vi "Washer HCC Newfi Main.vi"() -> ()   [LabVIEW 2018]
uses:
  Utility/Save File/Public/Type Definitions/Save File Washer.ctl
  Utility/Save File/File Setup (Public)/Type Definition/Save File DISH Dishwasher Details.ctl
  <vilib>/Platform/fileVersionInfo.llb/FileVersionInformation.ctl
  Washer DOE/Type Definitions/DOE Appliance Common.ctl
  Utility/Custom Pallet Controls/Custom Pallet String.ctl
  Utility/Save File/File Setup (Public)/Type Definition/DPT IMC Data.ctl
  Washer DOE/Type Definitions/DOE Dryer Standard.ctl
  Utility/Save File/Public/Type Definitions/Save File Appliance Display.ctl
  Utility/Save File/Public/Type Definitions/Save File Unit Type.ctl
  Utility/Save File/File Setup (Public)/Type Definition/Save File DOE File Path Control.ctl
  Utility/Save File/File Setup (Public)/Type Definition/Save File DOE Data Save Filepaths.ctl
  Type Definitions/HCC Station Group.ctl
  Utility/Save File/Save File.lvlib
  Drivers/Agilent 34972/Agilent 34970.lvlib
  Utility/Save File/File Setup.lvlib
panel:
  out "Network Var Set":u8
  in  "Quit":bool
  in  "Tab Control":enum32{"Main", "Settings"}(tab)
  in  "Array 4":T1[](array[typedef])=[{"Appliance Details"={"FileVersionInfo"={"FileVersion"="", "ProductName"="", "InternalName"="", "CompanyName"="", "LegalCopyright"="", "FileDescription"=""}, "Dishwasher Info"={"Open Cup Weight (gm):"=0.0, "Auto Cup Weight (gm):"=0.0, "Detergent-Dish:"="", "Inlet Temperature-Dish:"="", "Cycle Mode-Dish:"="", "Unit Control-Dish:"="", "Manufacturer-Dish:"=""}, "Washer Info"={"Hot Water Temperature (Fahrenheit):"="", "Cold Water Temperature (Fahrenheit):"="", "Capacity (cu.ft):"=0.0, "Initial Cloth Weight:"=0.0, "Cloth Lot:"=0, "Model Family:"="", "Program Name:"="", "Cycle Selection:"="", "Wash Temperature:"="", "Rinse Temperature:"="", "Load Size:"=""}, "File Name Output Array"=[], "Calibration Output Array"=[], "Appliance Common"={"Engineer:"="", "Model Number:"="", "Serial Number:"="", "Comments:"="", "Station ID:"="", "Technician:"="", "TR Number:"="", "Lab ID:"="", "Voltage:"="", "Water Pressure (PSI):"="", "Test Date:"="", "Computer Name:"="", "IP Address:"="", "Ambient RH:"="", "Frequency:"="", "Build:"="", "Filename:"="", "Test Type:"="", "Load Run #:"=0, "Ambient Temperature (F):"="", "File Path:"=path "", "Cycles Per Year"=60}, "Water Heater"={"Heating Mode:"=""}, "Dryer"={"Heat Setting:"="", "Washer Water Temperature (60 ± 5°F):"=60, "Water Hardness (PPM):"=17, "Dryness Setting:"="", "Dryer Type:"="", "Exhaust:"="", "Drying Cycle:"="", "Load Type:"="", "Nominal Load Weight"="", "Dryer Initial IMC Data"={"Measured IMC (lbs)"=7.0, "Actual Initial RMC (%)"=7.0, "RMC (Desired %)"=100.0, "Bone Dry Wt(lbs)"=7.0, "Tolerance(%)"=5.0, "Actual Final RMC (%)"=7.0, "CEF (lbf/kWh)"=0.0, "Minimum Weight (lbf)"=0.0, "Average Weight (lbf)"=0.0, "Maximum Weight (lbf)"=0.0, "Measured IMC In Range?"=FALSE, "Moisture Reduction Factor"=55.5, "Field Use Factor"=1.04, "Empty Dryer Cold Weigth"=0.0, "Energy Standard"=enum."D2-Automatic Dryer", "Weight Cloth (lbs)"=0.0, "Relative Moisture Content (%)"=0.0, "Relative Moisture Content - Avg (%)"=0.0}}}, "Display Data (RLT)"={"Status Color"=0, "Serial Number Display"="", "Cycle Count Display"=0, "Station Label Display"="", "Current Run Start Time Display"=0.0, "Board ID Display"="", "RPM Display"=0, "Current Display"=0.0, "Current Path Display"=path "", "Saving Display"=FALSE, "Unit Type Display"=enum."", "Total Time On Display"=0.0, "UI Button"=FALSE}}, {"Appliance Details"={"FileVersionInfo"={"FileVersion"="", "ProductName"="", "InternalName"="", "CompanyName"="", "LegalCopyright"="", "FileDescription"=""}, "Dishwasher Info"={"Open Cup Weight (gm):"=0.0, "Auto Cup Weight (gm):"=0.0, "Detergent-Dish:"="", "Inlet Temperature-Dish:"="", "Cycle Mode-Dish:"="", "Unit Control-Dish:"="", "Manufacturer-Dish:"=""}, "Washer Info"={"Hot Water Temperature (Fahrenheit):"="", "Cold Water Temperature (Fahrenheit):"="", "Capacity (cu.ft):"=0.0, "Initial Cloth Weight:"=0.0, "Cloth Lot:"=0, "Model Family:"="", "Program Name:"="", "Cycle Selection:"="", "Wash Temperature:"="", "Rinse Temperature:"="", "Load Size:"=""}, "File Name Output Array"=[], "Calibration Output Array"=[], "Appliance Common"={"Engineer:"="", "Model Number:"="", "Serial Number:"="", "Comments:"="", "Station ID:"="", "Technician:"="", "TR Number:"="", "Lab ID:"="", "Voltage:"="", "Water Pressure (PSI):"="", "Test Date:"="", "Computer Name:"="", "IP Address:"="", "Ambient RH:"="", "Frequency:"="", "Build:"="", "Filename:"="", "Test Type:"="", "Load Run #:"=0, "Ambient Temperature (F):"="", "File Path:"=path "", "Cycles Per Year"=60}, "Water Heater"={"Heating Mode:"=""}, "Dryer"={"Heat Setting:"="", "Washer Water Temperature (60 ± 5°F):"=60, "Water Hardness (PPM):"=17, "Dryness Setting:"="", "Dryer Type:"="", "Exhaust:"="", "Drying Cycle:"="", "Load Type:"="", "Nominal Load Weight"="", "Dryer Initial IMC Data"={"Measured IMC (lbs)"=7.0, "Actual Initial RMC (%)"=7.0, "RMC (Desired %)"=100.0, "Bone Dry Wt(lbs)"=7.0, "Tolerance(%)"=5.0, "Actual Final RMC (%)"=7.0, "CEF (lbf/kWh)"=0.0, "Minimum Weight (lbf)"=0.0, "Average Weight (lbf)"=0.0, "Maximum Weight (lbf)"=0.0, "Measured IMC In Range?"=FALSE, "Moisture Reduction Factor"=55.5, "Field Use Factor"=1.04, "Empty Dryer Cold Weigth"=0.0, "Energy Standard"=enum."D2-Automatic Dryer", "Weight Cloth (lbs)"=0.0, "Relative Moisture Content (%)"=0.0, "Relative Moisture Content - Avg (%)"=0.0}}}, "Display Data (RLT)"={"Status Color"=0, "Serial Number Display"="", "Cycle Count Display"=0, "Station Label Display"="", "Current Run Start Time Display"=0.0, "Board ID Display"="", "RPM Display"=0, "Current Display"=0.0, "Current Path Display"=path "", "Saving Display"=FALSE, "Unit Type Display"=enum."", "Total Time On Display"=0.0, "UI Button"=FALSE}}, {"Appliance Details"={"FileVersionInfo"={"FileVersion"="", "ProductName"="", "InternalName"="", "CompanyName"="", "LegalCopyright"="", "FileDescription"=""}, "Dishwasher Info"={"Open Cup Weight (gm):"=0.0, "Auto Cup Weight (gm):"=0.0, "Detergent-Dish:"="", "Inlet Temperature-Dish:"="", "Cycle Mode-Dish:"="", "Unit Control-Dish:"="", "Manufacturer-Dish:"=""}, "Washer Info"={"Hot Water Temperature (Fahrenheit):"="", "Cold Water Temperature (Fahrenheit):"="", "Capacity (cu.ft):"=0.0, "Initial Cloth Weight:"=0.0, "Cloth Lot:"=0, "Model Family:"="", "Program Name:"="", "Cycle Selection:"="", "Wash Temperature:"="", "Rinse Temperature:"="", "Load Size:"=""}, "File Name Output Array"=[], "Calibration Output Array"=[], "Appliance Common"={"Engineer:"="", "Model Number:"="", "Serial Number:"="", "Comments:"="", "Station ID:"="", "Technician:"="", "TR Number:"="", "Lab ID:"="", "Voltage:"="", "Water Pressure (PSI):"="", "Test Date:"="", "Computer Name:"="", "IP Address:"="", "Ambient RH:"="", "Frequency:"="", "Build:"="", "Filename:"="", "Test Type:"="", "Load Run #:"=0, "Ambient Temperature (F):"="", "File Path:"=path "", "Cycles Per Year"=60}, "Water Heater"={"Heating Mode:"=""}, "Dryer"={"Heat Setting:"="", "Washer Water Temperature (60 ± 5°F):"=60, "Water Hardness (PPM):"=17, "Dryness Setting:"="", "Dryer Type:"="", "Exhaust:"="", "Drying Cycle:"="", "Load Type:"="", "Nominal Load Weight"="", "Dryer Initial IMC Data"={"Measured IMC (lbs)"=7.0, "Actual Initial RMC (%)"=7.0, "RMC (Desired %)"=100.0, "Bone Dry Wt(lbs)"=7.0, "Tolerance(%)"=5.0, "Actual Final RMC (%)"=7.0, "CEF (lbf/kWh)"=0.0, "Minimum Weight (lbf)"=0.0, "Average Weight (lbf)"=0.0, "Maximum Weight (lbf)"=0.0, "Measured IMC In Range?"=FALSE, "Moisture Reduction Factor"=55.5, "Field Use Factor"=1.04, "Empty Dryer Cold Weigth"=0.0, "Energy Standard"=enum."D2-Automatic Dryer", "Weight Cloth (lbs)"=0.0, "Relative Moisture Content (%)"=0.0, "Relative Moisture Content - Avg (%)"=0.0}}}, "Display Data (RLT)"={"Status Color"=0, "Serial Number Display"="", "Cycle Count Display"=0, "Station Label Display"="", "Current Run Start Time Display"=0.0, "Board ID Display"="", "RPM Display"=0, "Current Display"=0.0, "Current Path Display"=path "", "Saving Display"=FALSE, "Unit Type Display"=enum."", "Total Time On Display"=0.0, "UI Button"=FALSE}}, {"Appliance Details"={"FileVersionInfo"={"FileVersion"="", "ProductName"="", "InternalName"="", "CompanyName"="", "LegalCopyright"="", "FileDescription"=""}, "Dishwasher Info"={"Open Cup Weight (gm):"=0.0, "Auto Cup Weight (gm):"=0.0, "Detergent-Dish:"="", "Inlet Temperature-Dish:"="", "Cycle Mode-Dish:"="", "Unit Control-Dish:"="", "Manufacturer-Dish:"=""}, "Washer Info"={"Hot Water Temperature (Fahrenheit):"="", "Cold Water Temperature (Fahrenheit):"="", "Capacity (cu.ft):"=0.0, "Initial Cloth Weight:"=0.0, "Cloth Lot:"=0, "Model Family:"="", "Program Name:"="", "Cycle Selection:"="", "Wash Temperature:"="", "Rinse Temperature:"="", "Load Size:"=""}, "File Name Output Array"=[], "Calibration Output Array"=[], "Appliance Common"={"Engineer:"="", "Model Number:"="", "Serial Number:"="", "Comments:"="", "Station ID:"="", "Technician:"="", "TR Number:"="", "Lab ID:"="", "Voltage:"="", "Water Pressure (PSI):"="", "Test Date:"="", "Computer Name:"="", "IP Address:"="", "Ambient RH:"="", "Frequency:"="", "Build:"="", "Filename:"="", "Test Type:"="", "Load Run #:"=0, "Ambient Temperature (F):"="", "File Path:"=path "", "Cycles Per Year"=60}, "Water Heater"={"Heating Mode:"=""}, "Dryer"={"Heat Setting:"="", "Washer Water Temperature (60 ± 5°F):"=60, "Water Hardness (PPM):"=17, "Dryness Setting:"="", "Dryer Type:"="", "Exhaust:"="", "Drying Cycle:"="", "Load Type:"="", "Nominal Load Weight"="", "Dryer Initial IMC Data"={"Measured IMC (lbs)"=7.0, "Actual Initial RMC (%)"=7.0, "RMC (Desired %)"=100.0, "Bone Dry Wt(lbs)"=7.0, "Tolerance(%)"=5.0, "Actual Final RMC (%)"=7.0, "CEF (lbf/kWh)"=0.0, "Minimum Weight (lbf)"=0.0, "Average Weight (lbf)"=0.0, "Maximum Weight (lbf)"=0.0, "Measured IMC In Range?"=FALSE, "Moisture Reduction Factor"=55.5, "Field Use Factor"=1.04, "Empty Dryer Cold Weigth"=0.0, "Energy Standard"=enum."D2-Automatic Dryer", "Weight Cloth (lbs)"=0.0, "Relative Moisture Content (%)"=0.0, "Relative Moisture Content - Avg (%)"=0.0}}}, "Display Data (RLT)"={"Status Color"=0, "Serial Number Display"="", "Cycle Count Display"=0, "Station Label Display"="", "Current Run Start Time Display"=0.0, "Board ID Display"="", "RPM Display"=0, "Current Display"=0.0, "Current Path Display"=path "", "Saving Display"=FALSE, "Unit Type Display"=enum."", "Total Time On Display"=0.0, "UI Button"=FALSE}}, {"Appliance Details"={"FileVersionInfo"={"FileVersion"="", "ProductName"="", "InternalName"="", "CompanyName"="", "LegalCopyright"="", "FileDescription"=""}, "Dishwasher Info"={"Open Cup Weight (gm):"=0.0, "Auto Cup Weight (gm):"=0.0, "Detergent-Dish:"="", "Inlet Temperature-Dish:"="", "Cycle Mode-Dish:"="", "Unit Control-Dish:"="", "Manufacturer-Dish:"=""}, "Washer Info"={"Hot Water Temperature (Fahrenheit):"="", "Cold Water Temperature (Fahrenheit):"="", "Capacity (cu.ft):"=0.0, "Initial Cloth Weight:"=0.0, "Cloth Lot:"=0, "Model Family:"="", "Program Name:"="", "Cycle Selection:"="", "Wash Temperature:"="", "Rinse Temperature:"="", "Load Size:"=""}, "File Name Output Array"=[], "Calibration Output Array"=[], "Appliance Common"={"Engineer:"="", "Model Number:"="", "Serial Number:"="", "Comments:"="", "Station ID:"="", "Technician:"="", "TR Number:"="", "Lab ID:"="", "Voltage:"="", "Water Pressure (PSI):"="", "Test Date:"="", "Computer Name:"="", "IP Address:"="", "Ambient RH:"="", "Frequency:"="", "Build:"="", "Filename:"="", "Test Type:"="", "Load Run #:"=0, "Ambient Temperature (F):"="", "File Path:"=path "", "Cycles Per Year"=60}, "Water Heater"={"Heating Mode:"=""}, "Dryer"={"Heat Setting:"="", "Washer Water Temperature (60 ± 5°F):"=60, "Water Hardness (PPM):"=17, "Dryness Setting:"="", "Dryer Type:"="", "Exhaust:"="", "Drying Cycle:"="", "Load Type:"="", "Nominal Load Weight"="", "Dryer Initial IMC Data"={"Measured IMC (lbs)"=7.0, "Actual Initial RMC (%)"=7.0, "RMC (Desired %)"=100.0, "Bone Dry Wt(lbs)"=7.0, "Tolerance(%)"=5.0, "Actual Final RMC (%)"=7.0, "CEF (lbf/kWh)"=0.0, "Minimum Weight (lbf)"=0.0, "Average Weight (lbf)"=0.0, "Maximum Weight (lbf)"=0.0, "Measured IMC In Range?"=FALSE, "Moisture Reduction Factor"=55.5, "Field Use Factor"=1.04, "Empty Dryer Cold Weigth"=0.0, "Energy Standard"=enum."D2-Automatic Dryer", "Weight Cloth (lbs)"=0.0, "Relative Moisture Content (%)"=0.0, "Relative Moisture Content - Avg (%)"=0.0}}}, "Display Data (RLT)"={"Status Color"=0, "Serial Number Display"="", "Cycle Count Display"=0, "Station Label Display"="", "Current Run Start Time Display"=0.0, "Board ID Display"="", "RPM Display"=0, "Current Display"=0.0, "Current Path Display"=path "", "Saving Display"=FALSE, "Unit Type Display"=enum."", "Total Time On Display"=0.0, "UI Button"=FALSE}}, {"Appliance Details"={"FileVersionInfo"={"FileVersion"="", "ProductName"="", "InternalName"="", "CompanyName"="", "LegalCopyright"="", "FileDescription"=""}, "Dishwasher Info"={"Open Cup Weight (gm):"=0.0, "Auto Cup Weight (gm):"=0.0, "Detergent-Dish:"="", "Inlet Temperature-Dish:"="", "Cycle Mode-Dish:"="", "Unit Control-Dish:"="", "Manufacturer-Dish:"=""}, "Washer Info"={"Hot Water Temperature (Fahrenheit):"="", "Cold Water Temperature (Fahrenheit):"="", "Capacity (cu.ft):"=0.0, "Initial Cloth Weight:"=0.0, "Cloth Lot:"=0, "Model Family:"="", "Program Name:"="", "Cycle Selection:"="", "Wash Temperature:"="", "Rinse Temperature:"="", "Load Size:"=""}, "File Name Output Array"=[], "Calibration Output Array"=[], "Appliance Common"={"Engineer:"="", "Model Number:"="", "Serial Number:"="", "Comments:"="", "Station ID:"="", "Technician:"="", "TR Number:"="", "Lab ID:"="", "Voltage:"="", "Water Pressure (PSI):"="", "Test Date:"="", "Computer Name:"="", "IP Address:"="", "Ambient RH:"="", "Frequency:"="", "Build:"="", "Filename:"="", "Test Type:"="", "Load Run #:"=0, "Ambient Temperature (F):"="", "File Path:"=path "", "Cycles Per Year"=60}, "Water Heater"={"Heating Mode:"=""}, "Dryer"={"Heat Setting:"="", "Washer Water Temperature (60 ± 5°F):"=60, "Water Hardness (PPM):"=17, "Dryness Setting:"="", "Dryer Type:"="", "Exhaust:"="", "Drying Cycle:"="", "Load Type:"="", "Nominal Load Weight"="", "Dryer Initial IMC Data"={"Measured IMC (lbs)"=7.0, "Actual Initial RMC (%)"=7.0, "RMC (Desired %)"=100.0, "Bone Dry Wt(lbs)"=7.0, "Tolerance(%)"=5.0, "Actual Final RMC (%)"=7.0, "CEF (lbf/kWh)"=0.0, "Minimum Weight (lbf)"=0.0, "Average Weight (lbf)"=0.0, "Maximum Weight (lbf)"=0.0, "Measured IMC In Range?"=FALSE, "Moisture Reduction Factor"=55.5, "Field Use Factor"=1.04, "Empty Dryer Cold Weigth"=0.0, "Energy Standard"=enum."D2-Automatic Dryer", "Weight Cloth (lbs)"=0.0, "Relative Moisture Content (%)"=0.0, "Relative Moisture Content - Avg (%)"=0.0}}}, "Display Data (RLT)"={"Status Color"=0, "Serial Number Display"="", "Cycle Count Display"=0, "Station Label Display"="", "Current Run Start Time Display"=0.0, "Board ID Display"="", "RPM Display"=0, "Current Display"=0.0, "Current Path Display"=path "", "Saving Display"=FALSE, "Unit Type Display"=enum."", "Total Time On Display"=0.0, "UI Button"=FALSE}}] {"Display Data (RLT)"."Current Display" format="%.2f"; "Display Data (RLT)"."Cycle Count Display" format="%04d"; "Appliance Details"."Dryer"."Dryer Initial IMC Data"."Maximum Weight (lbf)" format="%03_6g"; "Appliance Details"."Dryer"."Dryer Initial IMC Data"."Average Weight (lbf)" format="%03_6g"; "Appliance Details"."Dryer"."Dryer Initial IMC Data"."Minimum Weight (lbf)" format="%03_6g"; "Appliance Details"."Dryer"."Dryer Initial IMC Data"."CEF (lbf/kWh)" format="%03_6g"; "Appliance Details"."Dryer"."Dryer Initial IMC Data"."Actual Final RMC (%)" format="%03_6g"; "Appliance Details"."Dryer"."Dryer Initial IMC Data"."Tolerance(%)" format="%0#_6g"; "Appliance Details"."Dryer"."Dryer Initial IMC Data"."Bone Dry Wt(lbs)" format="%03_6g"; "Appliance Details"."Dryer"."Dryer Initial IMC Data"."RMC (Desired %)" format="%0#_6g"; "Appliance Details"."Dryer"."Dryer Initial IMC Data"."Actual Initial RMC (%)" format="%03_6g"; "Appliance Details"."Dryer"."Dryer Initial IMC Data"."Measured IMC (lbs)" format="%0#_6g"}
  in  "Array 3":T1[](array[typedef])=[{"Appliance Details"={"FileVersionInfo"={"FileVersion"="", "ProductName"="", "InternalName"="", "CompanyName"="", "LegalCopyright"="", "FileDescription"=""}, "Dishwasher Info"={"Open Cup Weight (gm):"=0.0, "Auto Cup Weight (gm):"=0.0, "Detergent-Dish:"="", "Inlet Temperature-Dish:"="", "Cycle Mode-Dish:"="", "Unit Control-Dish:"="", "Manufacturer-Dish:"=""}, "Washer Info"={"Hot Water Temperature (Fahrenheit):"="", "Cold Water Temperature (Fahrenheit):"="", "Capacity (cu.ft):"=0.0, "Initial Cloth Weight:"=0.0, "Cloth Lot:"=0, "Model Family:"="", "Program Name:"="", "Cycle Selection:"="", "Wash Temperature:"="", "Rinse Temperature:"="", "Load Size:"=""}, "File Name Output Array"=[], "Calibration Output Array"=[], "Appliance Common"={"Engineer:"="", "Model Number:"="", "Serial Number:"="", "Comments:"="", "Station ID:"="", "Technician:"="", "TR Number:"="", "Lab ID:"="", "Voltage:"="", "Water Pressure (PSI):"="", "Test Date:"="", "Computer Name:"="", "IP Address:"="", "Ambient RH:"="", "Frequency:"="", "Build:"="", "Filename:"="", "Test Type:"="", "Load Run #:"=0, "Ambient Temperature (F):"="", "File Path:"=path "", "Cycles Per Year"=60}, "Water Heater"={"Heating Mode:"=""}, "Dryer"={"Heat Setting:"="", "Washer Water Temperature (60 ± 5°F):"=60, "Water Hardness (PPM):"=17, "Dryness Setting:"="", "Dryer Type:"="", "Exhaust:"="", "Drying Cycle:"="", "Load Type:"="", "Nominal Load Weight"="", "Dryer Initial IMC Data"={"Measured IMC (lbs)"=7.0, "Actual Initial RMC (%)"=7.0, "RMC (Desired %)"=100.0, "Bone Dry Wt(lbs)"=7.0, "Tolerance(%)"=5.0, "Actual Final RMC (%)"=7.0, "CEF (lbf/kWh)"=0.0, "Minimum Weight (lbf)"=0.0, "Average Weight (lbf)"=0.0, "Maximum Weight (lbf)"=0.0, "Measured IMC In Range?"=FALSE, "Moisture Reduction Factor"=55.5, "Field Use Factor"=1.04, "Empty Dryer Cold Weigth"=0.0, "Energy Standard"=enum."D2-Automatic Dryer", "Weight Cloth (lbs)"=0.0, "Relative Moisture Content (%)"=0.0, "Relative Moisture Content - Avg (%)"=0.0}}}, "Display Data (RLT)"={"Status Color"=0, "Serial Number Display"="", "Cycle Count Display"=0, "Station Label Display"="", "Current Run Start Time Display"=0.0, "Board ID Display"="", "RPM Display"=0, "Current Display"=0.0, "Current Path Display"=path "", "Saving Display"=FALSE, "Unit Type Display"=enum."", "Total Time On Display"=0.0, "UI Button"=FALSE}}, {"Appliance Details"={"FileVersionInfo"={"FileVersion"="", "ProductName"="", "InternalName"="", "CompanyName"="", "LegalCopyright"="", "FileDescription"=""}, "Dishwasher Info"={"Open Cup Weight (gm):"=0.0, "Auto Cup Weight (gm):"=0.0, "Detergent-Dish:"="", "Inlet Temperature-Dish:"="", "Cycle Mode-Dish:"="", "Unit Control-Dish:"="", "Manufacturer-Dish:"=""}, "Washer Info"={"Hot Water Temperature (Fahrenheit):"="", "Cold Water Temperature (Fahrenheit):"="", "Capacity (cu.ft):"=0.0, "Initial Cloth Weight:"=0.0, "Cloth Lot:"=0, "Model Family:"="", "Program Name:"="", "Cycle Selection:"="", "Wash Temperature:"="", "Rinse Temperature:"="", "Load Size:"=""}, "File Name Output Array"=[], "Calibration Output Array"=[], "Appliance Common"={"Engineer:"="", "Model Number:"="", "Serial Number:"="", "Comments:"="", "Station ID:"="", "Technician:"="", "TR Number:"="", "Lab ID:"="", "Voltage:"="", "Water Pressure (PSI):"="", "Test Date:"="", "Computer Name:"="", "IP Address:"="", "Ambient RH:"="", "Frequency:"="", "Build:"="", "Filename:"="", "Test Type:"="", "Load Run #:"=0, "Ambient Temperature (F):"="", "File Path:"=path "", "Cycles Per Year"=60}, "Water Heater"={"Heating Mode:"=""}, "Dryer"={"Heat Setting:"="", "Washer Water Temperature (60 ± 5°F):"=60, "Water Hardness (PPM):"=17, "Dryness Setting:"="", "Dryer Type:"="", "Exhaust:"="", "Drying Cycle:"="", "Load Type:"="", "Nominal Load Weight"="", "Dryer Initial IMC Data"={"Measured IMC (lbs)"=7.0, "Actual Initial RMC (%)"=7.0, "RMC (Desired %)"=100.0, "Bone Dry Wt(lbs)"=7.0, "Tolerance(%)"=5.0, "Actual Final RMC (%)"=7.0, "CEF (lbf/kWh)"=0.0, "Minimum Weight (lbf)"=0.0, "Average Weight (lbf)"=0.0, "Maximum Weight (lbf)"=0.0, "Measured IMC In Range?"=FALSE, "Moisture Reduction Factor"=55.5, "Field Use Factor"=1.04, "Empty Dryer Cold Weigth"=0.0, "Energy Standard"=enum."D2-Automatic Dryer", "Weight Cloth (lbs)"=0.0, "Relative Moisture Content (%)"=0.0, "Relative Moisture Content - Avg (%)"=0.0}}}, "Display Data (RLT)"={"Status Color"=0, "Serial Number Display"="", "Cycle Count Display"=0, "Station Label Display"="", "Current Run Start Time Display"=0.0, "Board ID Display"="", "RPM Display"=0, "Current Display"=0.0, "Current Path Display"=path "", "Saving Display"=FALSE, "Unit Type Display"=enum."", "Total Time On Display"=0.0, "UI Button"=FALSE}}, {"Appliance Details"={"FileVersionInfo"={"FileVersion"="", "ProductName"="", "InternalName"="", "CompanyName"="", "LegalCopyright"="", "FileDescription"=""}, "Dishwasher Info"={"Open Cup Weight (gm):"=0.0, "Auto Cup Weight (gm):"=0.0, "Detergent-Dish:"="", "Inlet Temperature-Dish:"="", "Cycle Mode-Dish:"="", "Unit Control-Dish:"="", "Manufacturer-Dish:"=""}, "Washer Info"={"Hot Water Temperature (Fahrenheit):"="", "Cold Water Temperature (Fahrenheit):"="", "Capacity (cu.ft):"=0.0, "Initial Cloth Weight:"=0.0, "Cloth Lot:"=0, "Model Family:"="", "Program Name:"="", "Cycle Selection:"="", "Wash Temperature:"="", "Rinse Temperature:"="", "Load Size:"=""}, "File Name Output Array"=[], "Calibration Output Array"=[], "Appliance Common"={"Engineer:"="", "Model Number:"="", "Serial Number:"="", "Comments:"="", "Station ID:"="", "Technician:"="", "TR Number:"="", "Lab ID:"="", "Voltage:"="", "Water Pressure (PSI):"="", "Test Date:"="", "Computer Name:"="", "IP Address:"="", "Ambient RH:"="", "Frequency:"="", "Build:"="", "Filename:"="", "Test Type:"="", "Load Run #:"=0, "Ambient Temperature (F):"="", "File Path:"=path "", "Cycles Per Year"=60}, "Water Heater"={"Heating Mode:"=""}, "Dryer"={"Heat Setting:"="", "Washer Water Temperature (60 ± 5°F):"=60, "Water Hardness (PPM):"=17, "Dryness Setting:"="", "Dryer Type:"="", "Exhaust:"="", "Drying Cycle:"="", "Load Type:"="", "Nominal Load Weight"="", "Dryer Initial IMC Data"={"Measured IMC (lbs)"=7.0, "Actual Initial RMC (%)"=7.0, "RMC (Desired %)"=100.0, "Bone Dry Wt(lbs)"=7.0, "Tolerance(%)"=5.0, "Actual Final RMC (%)"=7.0, "CEF (lbf/kWh)"=0.0, "Minimum Weight (lbf)"=0.0, "Average Weight (lbf)"=0.0, "Maximum Weight (lbf)"=0.0, "Measured IMC In Range?"=FALSE, "Moisture Reduction Factor"=55.5, "Field Use Factor"=1.04, "Empty Dryer Cold Weigth"=0.0, "Energy Standard"=enum."D2-Automatic Dryer", "Weight Cloth (lbs)"=0.0, "Relative Moisture Content (%)"=0.0, "Relative Moisture Content - Avg (%)"=0.0}}}, "Display Data (RLT)"={"Status Color"=0, "Serial Number Display"="", "Cycle Count Display"=0, "Station Label Display"="", "Current Run Start Time Display"=0.0, "Board ID Display"="", "RPM Display"=0, "Current Display"=0.0, "Current Path Display"=path "", "Saving Display"=FALSE, "Unit Type Display"=enum."", "Total Time On Display"=0.0, "UI Button"=FALSE}}, {"Appliance Details"={"FileVersionInfo"={"FileVersion"="", "ProductName"="", "InternalName"="", "CompanyName"="", "LegalCopyright"="", "FileDescription"=""}, "Dishwasher Info"={"Open Cup Weight (gm):"=0.0, "Auto Cup Weight (gm):"=0.0, "Detergent-Dish:"="", "Inlet Temperature-Dish:"="", "Cycle Mode-Dish:"="", "Unit Control-Dish:"="", "Manufacturer-Dish:"=""}, "Washer Info"={"Hot Water Temperature (Fahrenheit):"="", "Cold Water Temperature (Fahrenheit):"="", "Capacity (cu.ft):"=0.0, "Initial Cloth Weight:"=0.0, "Cloth Lot:"=0, "Model Family:"="", "Program Name:"="", "Cycle Selection:"="", "Wash Temperature:"="", "Rinse Temperature:"="", "Load Size:"=""}, "File Name Output Array"=[], "Calibration Output Array"=[], "Appliance Common"={"Engineer:"="", "Model Number:"="", "Serial Number:"="", "Comments:"="", "Station ID:"="", "Technician:"="", "TR Number:"="", "Lab ID:"="", "Voltage:"="", "Water Pressure (PSI):"="", "Test Date:"="", "Computer Name:"="", "IP Address:"="", "Ambient RH:"="", "Frequency:"="", "Build:"="", "Filename:"="", "Test Type:"="", "Load Run #:"=0, "Ambient Temperature (F):"="", "File Path:"=path "", "Cycles Per Year"=60}, "Water Heater"={"Heating Mode:"=""}, "Dryer"={"Heat Setting:"="", "Washer Water Temperature (60 ± 5°F):"=60, "Water Hardness (PPM):"=17, "Dryness Setting:"="", "Dryer Type:"="", "Exhaust:"="", "Drying Cycle:"="", "Load Type:"="", "Nominal Load Weight"="", "Dryer Initial IMC Data"={"Measured IMC (lbs)"=7.0, "Actual Initial RMC (%)"=7.0, "RMC (Desired %)"=100.0, "Bone Dry Wt(lbs)"=7.0, "Tolerance(%)"=5.0, "Actual Final RMC (%)"=7.0, "CEF (lbf/kWh)"=0.0, "Minimum Weight (lbf)"=0.0, "Average Weight (lbf)"=0.0, "Maximum Weight (lbf)"=0.0, "Measured IMC In Range?"=FALSE, "Moisture Reduction Factor"=55.5, "Field Use Factor"=1.04, "Empty Dryer Cold Weigth"=0.0, "Energy Standard"=enum."D2-Automatic Dryer", "Weight Cloth (lbs)"=0.0, "Relative Moisture Content (%)"=0.0, "Relative Moisture Content - Avg (%)"=0.0}}}, "Display Data (RLT)"={"Status Color"=0, "Serial Number Display"="", "Cycle Count Display"=0, "Station Label Display"="", "Current Run Start Time Display"=0.0, "Board ID Display"="", "RPM Display"=0, "Current Display"=0.0, "Current Path Display"=path "", "Saving Display"=FALSE, "Unit Type Display"=enum."", "Total Time On Display"=0.0, "UI Button"=FALSE}}, {"Appliance Details"={"FileVersionInfo"={"FileVersion"="", "ProductName"="", "InternalName"="", "CompanyName"="", "LegalCopyright"="", "FileDescription"=""}, "Dishwasher Info"={"Open Cup Weight (gm):"=0.0, "Auto Cup Weight (gm):"=0.0, "Detergent-Dish:"="", "Inlet Temperature-Dish:"="", "Cycle Mode-Dish:"="", "Unit Control-Dish:"="", "Manufacturer-Dish:"=""}, "Washer Info"={"Hot Water Temperature (Fahrenheit):"="", "Cold Water Temperature (Fahrenheit):"="", "Capacity (cu.ft):"=0.0, "Initial Cloth Weight:"=0.0, "Cloth Lot:"=0, "Model Family:"="", "Program Name:"="", "Cycle Selection:"="", "Wash Temperature:"="", "Rinse Temperature:"="", "Load Size:"=""}, "File Name Output Array"=[], "Calibration Output Array"=[], "Appliance Common"={"Engineer:"="", "Model Number:"="", "Serial Number:"="", "Comments:"="", "Station ID:"="", "Technician:"="", "TR Number:"="", "Lab ID:"="", "Voltage:"="", "Water Pressure (PSI):"="", "Test Date:"="", "Computer Name:"="", "IP Address:"="", "Ambient RH:"="", "Frequency:"="", "Build:"="", "Filename:"="", "Test Type:"="", "Load Run #:"=0, "Ambient Temperature (F):"="", "File Path:"=path "", "Cycles Per Year"=60}, "Water Heater"={"Heating Mode:"=""}, "Dryer"={"Heat Setting:"="", "Washer Water Temperature (60 ± 5°F):"=60, "Water Hardness (PPM):"=17, "Dryness Setting:"="", "Dryer Type:"="", "Exhaust:"="", "Drying Cycle:"="", "Load Type:"="", "Nominal Load Weight"="", "Dryer Initial IMC Data"={"Measured IMC (lbs)"=7.0, "Actual Initial RMC (%)"=7.0, "RMC (Desired %)"=100.0, "Bone Dry Wt(lbs)"=7.0, "Tolerance(%)"=5.0, "Actual Final RMC (%)"=7.0, "CEF (lbf/kWh)"=0.0, "Minimum Weight (lbf)"=0.0, "Average Weight (lbf)"=0.0, "Maximum Weight (lbf)"=0.0, "Measured IMC In Range?"=FALSE, "Moisture Reduction Factor"=55.5, "Field Use Factor"=1.04, "Empty Dryer Cold Weigth"=0.0, "Energy Standard"=enum."D2-Automatic Dryer", "Weight Cloth (lbs)"=0.0, "Relative Moisture Content (%)"=0.0, "Relative Moisture Content - Avg (%)"=0.0}}}, "Display Data (RLT)"={"Status Color"=0, "Serial Number Display"="", "Cycle Count Display"=0, "Station Label Display"="", "Current Run Start Time Display"=0.0, "Board ID Display"="", "RPM Display"=0, "Current Display"=0.0, "Current Path Display"=path "", "Saving Display"=FALSE, "Unit Type Display"=enum."", "Total Time On Display"=0.0, "UI Button"=FALSE}}, {"Appliance Details"={"FileVersionInfo"={"FileVersion"="", "ProductName"="", "InternalName"="", "CompanyName"="", "LegalCopyright"="", "FileDescription"=""}, "Dishwasher Info"={"Open Cup Weight (gm):"=0.0, "Auto Cup Weight (gm):"=0.0, "Detergent-Dish:"="", "Inlet Temperature-Dish:"="", "Cycle Mode-Dish:"="", "Unit Control-Dish:"="", "Manufacturer-Dish:"=""}, "Washer Info"={"Hot Water Temperature (Fahrenheit):"="", "Cold Water Temperature (Fahrenheit):"="", "Capacity (cu.ft):"=0.0, "Initial Cloth Weight:"=0.0, "Cloth Lot:"=0, "Model Family:"="", "Program Name:"="", "Cycle Selection:"="", "Wash Temperature:"="", "Rinse Temperature:"="", "Load Size:"=""}, "File Name Output Array"=[], "Calibration Output Array"=[], "Appliance Common"={"Engineer:"="", "Model Number:"="", "Serial Number:"="", "Comments:"="", "Station ID:"="", "Technician:"="", "TR Number:"="", "Lab ID:"="", "Voltage:"="", "Water Pressure (PSI):"="", "Test Date:"="", "Computer Name:"="", "IP Address:"="", "Ambient RH:"="", "Frequency:"="", "Build:"="", "Filename:"="", "Test Type:"="", "Load Run #:"=0, "Ambient Temperature (F):"="", "File Path:"=path "", "Cycles Per Year"=60}, "Water Heater"={"Heating Mode:"=""}, "Dryer"={"Heat Setting:"="", "Washer Water Temperature (60 ± 5°F):"=60, "Water Hardness (PPM):"=17, "Dryness Setting:"="", "Dryer Type:"="", "Exhaust:"="", "Drying Cycle:"="", "Load Type:"="", "Nominal Load Weight"="", "Dryer Initial IMC Data"={"Measured IMC (lbs)"=7.0, "Actual Initial RMC (%)"=7.0, "RMC (Desired %)"=100.0, "Bone Dry Wt(lbs)"=7.0, "Tolerance(%)"=5.0, "Actual Final RMC (%)"=7.0, "CEF (lbf/kWh)"=0.0, "Minimum Weight (lbf)"=0.0, "Average Weight (lbf)"=0.0, "Maximum Weight (lbf)"=0.0, "Measured IMC In Range?"=FALSE, "Moisture Reduction Factor"=55.5, "Field Use Factor"=1.04, "Empty Dryer Cold Weigth"=0.0, "Energy Standard"=enum."D2-Automatic Dryer", "Weight Cloth (lbs)"=0.0, "Relative Moisture Content (%)"=0.0, "Relative Moisture Content - Avg (%)"=0.0}}}, "Display Data (RLT)"={"Status Color"=0, "Serial Number Display"="", "Cycle Count Display"=0, "Station Label Display"="", "Current Run Start Time Display"=0.0, "Board ID Display"="", "RPM Display"=0, "Current Display"=0.0, "Current Path Display"=path "", "Saving Display"=FALSE, "Unit Type Display"=enum."", "Total Time On Display"=0.0, "UI Button"=FALSE}}] {"Display Data (RLT)"."Current Display" format="%.2f"; "Display Data (RLT)"."Cycle Count Display" format="%04d"; "Appliance Details"."Dryer"."Dryer Initial IMC Data"."Maximum Weight (lbf)" format="%03_6g"; "Appliance Details"."Dryer"."Dryer Initial IMC Data"."Average Weight (lbf)" format="%03_6g"; "Appliance Details"."Dryer"."Dryer Initial IMC Data"."Minimum Weight (lbf)" format="%03_6g"; "Appliance Details"."Dryer"."Dryer Initial IMC Data"."CEF (lbf/kWh)" format="%03_6g"; "Appliance Details"."Dryer"."Dryer Initial IMC Data"."Actual Final RMC (%)" format="%03_6g"; "Appliance Details"."Dryer"."Dryer Initial IMC Data"."Tolerance(%)" format="%0#_6g"; "Appliance Details"."Dryer"."Dryer Initial IMC Data"."Bone Dry Wt(lbs)" format="%03_6g"; "Appliance Details"."Dryer"."Dryer Initial IMC Data"."RMC (Desired %)" format="%0#_6g"; "Appliance Details"."Dryer"."Dryer Initial IMC Data"."Actual Initial RMC (%)" format="%03_6g"; "Appliance Details"."Dryer"."Dryer Initial IMC Data"."Measured IMC (lbs)" format="%0#_6g"}
  in  "Array":T1[](array[typedef])=[{"Appliance Details"={"FileVersionInfo"={"FileVersion"="", "ProductName"="", "InternalName"="", "CompanyName"="", "LegalCopyright"="", "FileDescription"=""}, "Dishwasher Info"={"Open Cup Weight (gm):"=0.0, "Auto Cup Weight (gm):"=0.0, "Detergent-Dish:"="", "Inlet Temperature-Dish:"="", "Cycle Mode-Dish:"="", "Unit Control-Dish:"="", "Manufacturer-Dish:"=""}, "Washer Info"={"Hot Water Temperature (Fahrenheit):"="", "Cold Water Temperature (Fahrenheit):"="", "Capacity (cu.ft):"=0.0, "Initial Cloth Weight:"=0.0, "Cloth Lot:"=0, "Model Family:"="", "Program Name:"="", "Cycle Selection:"="", "Wash Temperature:"="", "Rinse Temperature:"="", "Load Size:"=""}, "File Name Output Array"=[], "Calibration Output Array"=[], "Appliance Common"={"Engineer:"="", "Model Number:"="", "Serial Number:"="", "Comments:"="", "Station ID:"="", "Technician:"="", "TR Number:"="", "Lab ID:"="", "Voltage:"="", "Water Pressure (PSI):"="", "Test Date:"="", "Computer Name:"="", "IP Address:"="", "Ambient RH:"="", "Frequency:"="", "Build:"="", "Filename:"="", "Test Type:"="", "Load Run #:"=0, "Ambient Temperature (F):"="", "File Path:"=path "", "Cycles Per Year"=60}, "Water Heater"={"Heating Mode:"=""}, "Dryer"={"Heat Setting:"="", "Washer Water Temperature (60 ± 5°F):"=60, "Water Hardness (PPM):"=17, "Dryness Setting:"="", "Dryer Type:"="", "Exhaust:"="", "Drying Cycle:"="", "Load Type:"="", "Nominal Load Weight"="", "Dryer Initial IMC Data"={"Measured IMC (lbs)"=7.0, "Actual Initial RMC (%)"=7.0, "RMC (Desired %)"=100.0, "Bone Dry Wt(lbs)"=7.0, "Tolerance(%)"=5.0, "Actual Final RMC (%)"=7.0, "CEF (lbf/kWh)"=0.0, "Minimum Weight (lbf)"=0.0, "Average Weight (lbf)"=0.0, "Maximum Weight (lbf)"=0.0, "Measured IMC In Range?"=FALSE, "Moisture Reduction Factor"=55.5, "Field Use Factor"=1.04, "Empty Dryer Cold Weigth"=0.0, "Energy Standard"=enum."D2-Automatic Dryer", "Weight Cloth (lbs)"=0.0, "Relative Moisture Content (%)"=0.0, "Relative Moisture Content - Avg (%)"=0.0}}}, "Display Data (RLT)"={"Status Color"=0, "Serial Number Display"="", "Cycle Count Display"=0, "Station Label Display"="", "Current Run Start Time Display"=0.0, "Board ID Display"="", "RPM Display"=0, "Current Display"=0.0, "Current Path Display"=path "", "Saving Display"=FALSE, "Unit Type Display"=enum."", "Total Time On Display"=0.0, "UI Button"=FALSE}}, {"Appliance Details"={"FileVersionInfo"={"FileVersion"="", "ProductName"="", "InternalName"="", "CompanyName"="", "LegalCopyright"="", "FileDescription"=""}, "Dishwasher Info"={"Open Cup Weight (gm):"=0.0, "Auto Cup Weight (gm):"=0.0, "Detergent-Dish:"="", "Inlet Temperature-Dish:"="", "Cycle Mode-Dish:"="", "Unit Control-Dish:"="", "Manufacturer-Dish:"=""}, "Washer Info"={"Hot Water Temperature (Fahrenheit):"="", "Cold Water Temperature (Fahrenheit):"="", "Capacity (cu.ft):"=0.0, "Initial Cloth Weight:"=0.0, "Cloth Lot:"=0, "Model Family:"="", "Program Name:"="", "Cycle Selection:"="", "Wash Temperature:"="", "Rinse Temperature:"="", "Load Size:"=""}, "File Name Output Array"=[], "Calibration Output Array"=[], "Appliance Common"={"Engineer:"="", "Model Number:"="", "Serial Number:"="", "Comments:"="", "Station ID:"="", "Technician:"="", "TR Number:"="", "Lab ID:"="", "Voltage:"="", "Water Pressure (PSI):"="", "Test Date:"="", "Computer Name:"="", "IP Address:"="", "Ambient RH:"="", "Frequency:"="", "Build:"="", "Filename:"="", "Test Type:"="", "Load Run #:"=0, "Ambient Temperature (F):"="", "File Path:"=path "", "Cycles Per Year"=60}, "Water Heater"={"Heating Mode:"=""}, "Dryer"={"Heat Setting:"="", "Washer Water Temperature (60 ± 5°F):"=60, "Water Hardness (PPM):"=17, "Dryness Setting:"="", "Dryer Type:"="", "Exhaust:"="", "Drying Cycle:"="", "Load Type:"="", "Nominal Load Weight"="", "Dryer Initial IMC Data"={"Measured IMC (lbs)"=7.0, "Actual Initial RMC (%)"=7.0, "RMC (Desired %)"=100.0, "Bone Dry Wt(lbs)"=7.0, "Tolerance(%)"=5.0, "Actual Final RMC (%)"=7.0, "CEF (lbf/kWh)"=0.0, "Minimum Weight (lbf)"=0.0, "Average Weight (lbf)"=0.0, "Maximum Weight (lbf)"=0.0, "Measured IMC In Range?"=FALSE, "Moisture Reduction Factor"=55.5, "Field Use Factor"=1.04, "Empty Dryer Cold Weigth"=0.0, "Energy Standard"=enum."D2-Automatic Dryer", "Weight Cloth (lbs)"=0.0, "Relative Moisture Content (%)"=0.0, "Relative Moisture Content - Avg (%)"=0.0}}}, "Display Data (RLT)"={"Status Color"=0, "Serial Number Display"="", "Cycle Count Display"=0, "Station Label Display"="", "Current Run Start Time Display"=0.0, "Board ID Display"="", "RPM Display"=0, "Current Display"=0.0, "Current Path Display"=path "", "Saving Display"=FALSE, "Unit Type Display"=enum."", "Total Time On Display"=0.0, "UI Button"=FALSE}}, {"Appliance Details"={"FileVersionInfo"={"FileVersion"="", "ProductName"="", "InternalName"="", "CompanyName"="", "LegalCopyright"="", "FileDescription"=""}, "Dishwasher Info"={"Open Cup Weight (gm):"=0.0, "Auto Cup Weight (gm):"=0.0, "Detergent-Dish:"="", "Inlet Temperature-Dish:"="", "Cycle Mode-Dish:"="", "Unit Control-Dish:"="", "Manufacturer-Dish:"=""}, "Washer Info"={"Hot Water Temperature (Fahrenheit):"="", "Cold Water Temperature (Fahrenheit):"="", "Capacity (cu.ft):"=0.0, "Initial Cloth Weight:"=0.0, "Cloth Lot:"=0, "Model Family:"="", "Program Name:"="", "Cycle Selection:"="", "Wash Temperature:"="", "Rinse Temperature:"="", "Load Size:"=""}, "File Name Output Array"=[], "Calibration Output Array"=[], "Appliance Common"={"Engineer:"="", "Model Number:"="", "Serial Number:"="", "Comments:"="", "Station ID:"="", "Technician:"="", "TR Number:"="", "Lab ID:"="", "Voltage:"="", "Water Pressure (PSI):"="", "Test Date:"="", "Computer Name:"="", "IP Address:"="", "Ambient RH:"="", "Frequency:"="", "Build:"="", "Filename:"="", "Test Type:"="", "Load Run #:"=0, "Ambient Temperature (F):"="", "File Path:"=path "", "Cycles Per Year"=60}, "Water Heater"={"Heating Mode:"=""}, "Dryer"={"Heat Setting:"="", "Washer Water Temperature (60 ± 5°F):"=60, "Water Hardness (PPM):"=17, "Dryness Setting:"="", "Dryer Type:"="", "Exhaust:"="", "Drying Cycle:"="", "Load Type:"="", "Nominal Load Weight"="", "Dryer Initial IMC Data"={"Measured IMC (lbs)"=7.0, "Actual Initial RMC (%)"=7.0, "RMC (Desired %)"=100.0, "Bone Dry Wt(lbs)"=7.0, "Tolerance(%)"=5.0, "Actual Final RMC (%)"=7.0, "CEF (lbf/kWh)"=0.0, "Minimum Weight (lbf)"=0.0, "Average Weight (lbf)"=0.0, "Maximum Weight (lbf)"=0.0, "Measured IMC In Range?"=FALSE, "Moisture Reduction Factor"=55.5, "Field Use Factor"=1.04, "Empty Dryer Cold Weigth"=0.0, "Energy Standard"=enum."D2-Automatic Dryer", "Weight Cloth (lbs)"=0.0, "Relative Moisture Content (%)"=0.0, "Relative Moisture Content - Avg (%)"=0.0}}}, "Display Data (RLT)"={"Status Color"=0, "Serial Number Display"="", "Cycle Count Display"=0, "Station Label Display"="", "Current Run Start Time Display"=0.0, "Board ID Display"="", "RPM Display"=0, "Current Display"=0.0, "Current Path Display"=path "", "Saving Display"=FALSE, "Unit Type Display"=enum."", "Total Time On Display"=0.0, "UI Button"=FALSE}}, {"Appliance Details"={"FileVersionInfo"={"FileVersion"="", "ProductName"="", "InternalName"="", "CompanyName"="", "LegalCopyright"="", "FileDescription"=""}, "Dishwasher Info"={"Open Cup Weight (gm):"=0.0, "Auto Cup Weight (gm):"=0.0, "Detergent-Dish:"="", "Inlet Temperature-Dish:"="", "Cycle Mode-Dish:"="", "Unit Control-Dish:"="", "Manufacturer-Dish:"=""}, "Washer Info"={"Hot Water Temperature (Fahrenheit):"="", "Cold Water Temperature (Fahrenheit):"="", "Capacity (cu.ft):"=0.0, "Initial Cloth Weight:"=0.0, "Cloth Lot:"=0, "Model Family:"="", "Program Name:"="", "Cycle Selection:"="", "Wash Temperature:"="", "Rinse Temperature:"="", "Load Size:"=""}, "File Name Output Array"=[], "Calibration Output Array"=[], "Appliance Common"={"Engineer:"="", "Model Number:"="", "Serial Number:"="", "Comments:"="", "Station ID:"="", "Technician:"="", "TR Number:"="", "Lab ID:"="", "Voltage:"="", "Water Pressure (PSI):"="", "Test Date:"="", "Computer Name:"="", "IP Address:"="", "Ambient RH:"="", "Frequency:"="", "Build:"="", "Filename:"="", "Test Type:"="", "Load Run #:"=0, "Ambient Temperature (F):"="", "File Path:"=path "", "Cycles Per Year"=60}, "Water Heater"={"Heating Mode:"=""}, "Dryer"={"Heat Setting:"="", "Washer Water Temperature (60 ± 5°F):"=60, "Water Hardness (PPM):"=17, "Dryness Setting:"="", "Dryer Type:"="", "Exhaust:"="", "Drying Cycle:"="", "Load Type:"="", "Nominal Load Weight"="", "Dryer Initial IMC Data"={"Measured IMC (lbs)"=7.0, "Actual Initial RMC (%)"=7.0, "RMC (Desired %)"=100.0, "Bone Dry Wt(lbs)"=7.0, "Tolerance(%)"=5.0, "Actual Final RMC (%)"=7.0, "CEF (lbf/kWh)"=0.0, "Minimum Weight (lbf)"=0.0, "Average Weight (lbf)"=0.0, "Maximum Weight (lbf)"=0.0, "Measured IMC In Range?"=FALSE, "Moisture Reduction Factor"=55.5, "Field Use Factor"=1.04, "Empty Dryer Cold Weigth"=0.0, "Energy Standard"=enum."D2-Automatic Dryer", "Weight Cloth (lbs)"=0.0, "Relative Moisture Content (%)"=0.0, "Relative Moisture Content - Avg (%)"=0.0}}}, "Display Data (RLT)"={"Status Color"=0, "Serial Number Display"="", "Cycle Count Display"=0, "Station Label Display"="", "Current Run Start Time Display"=0.0, "Board ID Display"="", "RPM Display"=0, "Current Display"=0.0, "Current Path Display"=path "", "Saving Display"=FALSE, "Unit Type Display"=enum."", "Total Time On Display"=0.0, "UI Button"=FALSE}}, {"Appliance Details"={"FileVersionInfo"={"FileVersion"="", "ProductName"="", "InternalName"="", "CompanyName"="", "LegalCopyright"="", "FileDescription"=""}, "Dishwasher Info"={"Open Cup Weight (gm):"=0.0, "Auto Cup Weight (gm):"=0.0, "Detergent-Dish:"="", "Inlet Temperature-Dish:"="", "Cycle Mode-Dish:"="", "Unit Control-Dish:"="", "Manufacturer-Dish:"=""}, "Washer Info"={"Hot Water Temperature (Fahrenheit):"="", "Cold Water Temperature (Fahrenheit):"="", "Capacity (cu.ft):"=0.0, "Initial Cloth Weight:"=0.0, "Cloth Lot:"=0, "Model Family:"="", "Program Name:"="", "Cycle Selection:"="", "Wash Temperature:"="", "Rinse Temperature:"="", "Load Size:"=""}, "File Name Output Array"=[], "Calibration Output Array"=[], "Appliance Common"={"Engineer:"="", "Model Number:"="", "Serial Number:"="", "Comments:"="", "Station ID:"="", "Technician:"="", "TR Number:"="", "Lab ID:"="", "Voltage:"="", "Water Pressure (PSI):"="", "Test Date:"="", "Computer Name:"="", "IP Address:"="", "Ambient RH:"="", "Frequency:"="", "Build:"="", "Filename:"="", "Test Type:"="", "Load Run #:"=0, "Ambient Temperature (F):"="", "File Path:"=path "", "Cycles Per Year"=60}, "Water Heater"={"Heating Mode:"=""}, "Dryer"={"Heat Setting:"="", "Washer Water Temperature (60 ± 5°F):"=60, "Water Hardness (PPM):"=17, "Dryness Setting:"="", "Dryer Type:"="", "Exhaust:"="", "Drying Cycle:"="", "Load Type:"="", "Nominal Load Weight"="", "Dryer Initial IMC Data"={"Measured IMC (lbs)"=7.0, "Actual Initial RMC (%)"=7.0, "RMC (Desired %)"=100.0, "Bone Dry Wt(lbs)"=7.0, "Tolerance(%)"=5.0, "Actual Final RMC (%)"=7.0, "CEF (lbf/kWh)"=0.0, "Minimum Weight (lbf)"=0.0, "Average Weight (lbf)"=0.0, "Maximum Weight (lbf)"=0.0, "Measured IMC In Range?"=FALSE, "Moisture Reduction Factor"=55.5, "Field Use Factor"=1.04, "Empty Dryer Cold Weigth"=0.0, "Energy Standard"=enum."D2-Automatic Dryer", "Weight Cloth (lbs)"=0.0, "Relative Moisture Content (%)"=0.0, "Relative Moisture Content - Avg (%)"=0.0}}}, "Display Data (RLT)"={"Status Color"=0, "Serial Number Display"="", "Cycle Count Display"=0, "Station Label Display"="", "Current Run Start Time Display"=0.0, "Board ID Display"="", "RPM Display"=0, "Current Display"=0.0, "Current Path Display"=path "", "Saving Display"=FALSE, "Unit Type Display"=enum."", "Total Time On Display"=0.0, "UI Button"=FALSE}}, {"Appliance Details"={"FileVersionInfo"={"FileVersion"="", "ProductName"="", "InternalName"="", "CompanyName"="", "LegalCopyright"="", "FileDescription"=""}, "Dishwasher Info"={"Open Cup Weight (gm):"=0.0, "Auto Cup Weight (gm):"=0.0, "Detergent-Dish:"="", "Inlet Temperature-Dish:"="", "Cycle Mode-Dish:"="", "Unit Control-Dish:"="", "Manufacturer-Dish:"=""}, "Washer Info"={"Hot Water Temperature (Fahrenheit):"="", "Cold Water Temperature (Fahrenheit):"="", "Capacity (cu.ft):"=0.0, "Initial Cloth Weight:"=0.0, "Cloth Lot:"=0, "Model Family:"="", "Program Name:"="", "Cycle Selection:"="", "Wash Temperature:"="", "Rinse Temperature:"="", "Load Size:"=""}, "File Name Output Array"=[], "Calibration Output Array"=[], "Appliance Common"={"Engineer:"="", "Model Number:"="", "Serial Number:"="", "Comments:"="", "Station ID:"="", "Technician:"="", "TR Number:"="", "Lab ID:"="", "Voltage:"="", "Water Pressure (PSI):"="", "Test Date:"="", "Computer Name:"="", "IP Address:"="", "Ambient RH:"="", "Frequency:"="", "Build:"="", "Filename:"="", "Test Type:"="", "Load Run #:"=0, "Ambient Temperature (F):"="", "File Path:"=path "", "Cycles Per Year"=60}, "Water Heater"={"Heating Mode:"=""}, "Dryer"={"Heat Setting:"="", "Washer Water Temperature (60 ± 5°F):"=60, "Water Hardness (PPM):"=17, "Dryness Setting:"="", "Dryer Type:"="", "Exhaust:"="", "Drying Cycle:"="", "Load Type:"="", "Nominal Load Weight"="", "Dryer Initial IMC Data"={"Measured IMC (lbs)"=7.0, "Actual Initial RMC (%)"=7.0, "RMC (Desired %)"=100.0, "Bone Dry Wt(lbs)"=7.0, "Tolerance(%)"=5.0, "Actual Final RMC (%)"=7.0, "CEF (lbf/kWh)"=0.0, "Minimum Weight (lbf)"=0.0, "Average Weight (lbf)"=0.0, "Maximum Weight (lbf)"=0.0, "Measured IMC In Range?"=FALSE, "Moisture Reduction Factor"=55.5, "Field Use Factor"=1.04, "Empty Dryer Cold Weigth"=0.0, "Energy Standard"=enum."D2-Automatic Dryer", "Weight Cloth (lbs)"=0.0, "Relative Moisture Content (%)"=0.0, "Relative Moisture Content - Avg (%)"=0.0}}}, "Display Data (RLT)"={"Status Color"=0, "Serial Number Display"="", "Cycle Count Display"=0, "Station Label Display"="", "Current Run Start Time Display"=0.0, "Board ID Display"="", "RPM Display"=0, "Current Display"=0.0, "Current Path Display"=path "", "Saving Display"=FALSE, "Unit Type Display"=enum."", "Total Time On Display"=0.0, "UI Button"=FALSE}}] {"Display Data (RLT)"."Current Display" format="%.2f"; "Display Data (RLT)"."Cycle Count Display" format="%04d"; "Appliance Details"."Dryer"."Dryer Initial IMC Data"."Maximum Weight (lbf)" format="%03_6g"; "Appliance Details"."Dryer"."Dryer Initial IMC Data"."Average Weight (lbf)" format="%03_6g"; "Appliance Details"."Dryer"."Dryer Initial IMC Data"."Minimum Weight (lbf)" format="%03_6g"; "Appliance Details"."Dryer"."Dryer Initial IMC Data"."CEF (lbf/kWh)" format="%03_6g"; "Appliance Details"."Dryer"."Dryer Initial IMC Data"."Actual Final RMC (%)" format="%03_6g"; "Appliance Details"."Dryer"."Dryer Initial IMC Data"."Tolerance(%)" format="%0#_6g"; "Appliance Details"."Dryer"."Dryer Initial IMC Data"."Bone Dry Wt(lbs)" format="%03_6g"; "Appliance Details"."Dryer"."Dryer Initial IMC Data"."RMC (Desired %)" format="%0#_6g"; "Appliance Details"."Dryer"."Dryer Initial IMC Data"."Actual Initial RMC (%)" format="%03_6g"; "Appliance Details"."Dryer"."Dryer Initial IMC Data"."Measured IMC (lbs)" format="%0#_6g"}
  in  "Array 2":T1[](array[typedef])=[{"Appliance Details"={"FileVersionInfo"={"FileVersion"="", "ProductName"="", "InternalName"="", "CompanyName"="", "LegalCopyright"="", "FileDescription"=""}, "Dishwasher Info"={"Open Cup Weight (gm):"=0.0, "Auto Cup Weight (gm):"=0.0, "Detergent-Dish:"="", "Inlet Temperature-Dish:"="", "Cycle Mode-Dish:"="", "Unit Control-Dish:"="", "Manufacturer-Dish:"=""}, "Washer Info"={"Hot Water Temperature (Fahrenheit):"="", "Cold Water Temperature (Fahrenheit):"="", "Capacity (cu.ft):"=0.0, "Initial Cloth Weight:"=0.0, "Cloth Lot:"=0, "Model Family:"="", "Program Name:"="", "Cycle Selection:"="", "Wash Temperature:"="", "Rinse Temperature:"="", "Load Size:"=""}, "File Name Output Array"=[], "Calibration Output Array"=[], "Appliance Common"={"Engineer:"="", "Model Number:"="", "Serial Number:"="", "Comments:"="", "Station ID:"="", "Technician:"="", "TR Number:"="", "Lab ID:"="", "Voltage:"="", "Water Pressure (PSI):"="", "Test Date:"="", "Computer Name:"="", "IP Address:"="", "Ambient RH:"="", "Frequency:"="", "Build:"="", "Filename:"="", "Test Type:"="", "Load Run #:"=0, "Ambient Temperature (F):"="", "File Path:"=path "", "Cycles Per Year"=60}, "Water Heater"={"Heating Mode:"=""}, "Dryer"={"Heat Setting:"="", "Washer Water Temperature (60 ± 5°F):"=60, "Water Hardness (PPM):"=17, "Dryness Setting:"="", "Dryer Type:"="", "Exhaust:"="", "Drying Cycle:"="", "Load Type:"="", "Nominal Load Weight"="", "Dryer Initial IMC Data"={"Measured IMC (lbs)"=7.0, "Actual Initial RMC (%)"=7.0, "RMC (Desired %)"=100.0, "Bone Dry Wt(lbs)"=7.0, "Tolerance(%)"=5.0, "Actual Final RMC (%)"=7.0, "CEF (lbf/kWh)"=0.0, "Minimum Weight (lbf)"=0.0, "Average Weight (lbf)"=0.0, "Maximum Weight (lbf)"=0.0, "Measured IMC In Range?"=FALSE, "Moisture Reduction Factor"=55.5, "Field Use Factor"=1.04, "Empty Dryer Cold Weigth"=0.0, "Energy Standard"=enum."D2-Automatic Dryer", "Weight Cloth (lbs)"=0.0, "Relative Moisture Content (%)"=0.0, "Relative Moisture Content - Avg (%)"=0.0}}}, "Display Data (RLT)"={"Status Color"=0, "Serial Number Display"="", "Cycle Count Display"=0, "Station Label Display"="", "Current Run Start Time Display"=0.0, "Board ID Display"="", "RPM Display"=0, "Current Display"=0.0, "Current Path Display"=path "", "Saving Display"=FALSE, "Unit Type Display"=enum."", "Total Time On Display"=0.0, "UI Button"=FALSE}}, {"Appliance Details"={"FileVersionInfo"={"FileVersion"="", "ProductName"="", "InternalName"="", "CompanyName"="", "LegalCopyright"="", "FileDescription"=""}, "Dishwasher Info"={"Open Cup Weight (gm):"=0.0, "Auto Cup Weight (gm):"=0.0, "Detergent-Dish:"="", "Inlet Temperature-Dish:"="", "Cycle Mode-Dish:"="", "Unit Control-Dish:"="", "Manufacturer-Dish:"=""}, "Washer Info"={"Hot Water Temperature (Fahrenheit):"="", "Cold Water Temperature (Fahrenheit):"="", "Capacity (cu.ft):"=0.0, "Initial Cloth Weight:"=0.0, "Cloth Lot:"=0, "Model Family:"="", "Program Name:"="", "Cycle Selection:"="", "Wash Temperature:"="", "Rinse Temperature:"="", "Load Size:"=""}, "File Name Output Array"=[], "Calibration Output Array"=[], "Appliance Common"={"Engineer:"="", "Model Number:"="", "Serial Number:"="", "Comments:"="", "Station ID:"="", "Technician:"="", "TR Number:"="", "Lab ID:"="", "Voltage:"="", "Water Pressure (PSI):"="", "Test Date:"="", "Computer Name:"="", "IP Address:"="", "Ambient RH:"="", "Frequency:"="", "Build:"="", "Filename:"="", "Test Type:"="", "Load Run #:"=0, "Ambient Temperature (F):"="", "File Path:"=path "", "Cycles Per Year"=60}, "Water Heater"={"Heating Mode:"=""}, "Dryer"={"Heat Setting:"="", "Washer Water Temperature (60 ± 5°F):"=60, "Water Hardness (PPM):"=17, "Dryness Setting:"="", "Dryer Type:"="", "Exhaust:"="", "Drying Cycle:"="", "Load Type:"="", "Nominal Load Weight"="", "Dryer Initial IMC Data"={"Measured IMC (lbs)"=7.0, "Actual Initial RMC (%)"=7.0, "RMC (Desired %)"=100.0, "Bone Dry Wt(lbs)"=7.0, "Tolerance(%)"=5.0, "Actual Final RMC (%)"=7.0, "CEF (lbf/kWh)"=0.0, "Minimum Weight (lbf)"=0.0, "Average Weight (lbf)"=0.0, "Maximum Weight (lbf)"=0.0, "Measured IMC In Range?"=FALSE, "Moisture Reduction Factor"=55.5, "Field Use Factor"=1.04, "Empty Dryer Cold Weigth"=0.0, "Energy Standard"=enum."D2-Automatic Dryer", "Weight Cloth (lbs)"=0.0, "Relative Moisture Content (%)"=0.0, "Relative Moisture Content - Avg (%)"=0.0}}}, "Display Data (RLT)"={"Status Color"=0, "Serial Number Display"="", "Cycle Count Display"=0, "Station Label Display"="", "Current Run Start Time Display"=0.0, "Board ID Display"="", "RPM Display"=0, "Current Display"=0.0, "Current Path Display"=path "", "Saving Display"=FALSE, "Unit Type Display"=enum."", "Total Time On Display"=0.0, "UI Button"=FALSE}}, {"Appliance Details"={"FileVersionInfo"={"FileVersion"="", "ProductName"="", "InternalName"="", "CompanyName"="", "LegalCopyright"="", "FileDescription"=""}, "Dishwasher Info"={"Open Cup Weight (gm):"=0.0, "Auto Cup Weight (gm):"=0.0, "Detergent-Dish:"="", "Inlet Temperature-Dish:"="", "Cycle Mode-Dish:"="", "Unit Control-Dish:"="", "Manufacturer-Dish:"=""}, "Washer Info"={"Hot Water Temperature (Fahrenheit):"="", "Cold Water Temperature (Fahrenheit):"="", "Capacity (cu.ft):"=0.0, "Initial Cloth Weight:"=0.0, "Cloth Lot:"=0, "Model Family:"="", "Program Name:"="", "Cycle Selection:"="", "Wash Temperature:"="", "Rinse Temperature:"="", "Load Size:"=""}, "File Name Output Array"=[], "Calibration Output Array"=[], "Appliance Common"={"Engineer:"="", "Model Number:"="", "Serial Number:"="", "Comments:"="", "Station ID:"="", "Technician:"="", "TR Number:"="", "Lab ID:"="", "Voltage:"="", "Water Pressure (PSI):"="", "Test Date:"="", "Computer Name:"="", "IP Address:"="", "Ambient RH:"="", "Frequency:"="", "Build:"="", "Filename:"="", "Test Type:"="", "Load Run #:"=0, "Ambient Temperature (F):"="", "File Path:"=path "", "Cycles Per Year"=60}, "Water Heater"={"Heating Mode:"=""}, "Dryer"={"Heat Setting:"="", "Washer Water Temperature (60 ± 5°F):"=60, "Water Hardness (PPM):"=17, "Dryness Setting:"="", "Dryer Type:"="", "Exhaust:"="", "Drying Cycle:"="", "Load Type:"="", "Nominal Load Weight"="", "Dryer Initial IMC Data"={"Measured IMC (lbs)"=7.0, "Actual Initial RMC (%)"=7.0, "RMC (Desired %)"=100.0, "Bone Dry Wt(lbs)"=7.0, "Tolerance(%)"=5.0, "Actual Final RMC (%)"=7.0, "CEF (lbf/kWh)"=0.0, "Minimum Weight (lbf)"=0.0, "Average Weight (lbf)"=0.0, "Maximum Weight (lbf)"=0.0, "Measured IMC In Range?"=FALSE, "Moisture Reduction Factor"=55.5, "Field Use Factor"=1.04, "Empty Dryer Cold Weigth"=0.0, "Energy Standard"=enum."D2-Automatic Dryer", "Weight Cloth (lbs)"=0.0, "Relative Moisture Content (%)"=0.0, "Relative Moisture Content - Avg (%)"=0.0}}}, "Display Data (RLT)"={"Status Color"=0, "Serial Number Display"="", "Cycle Count Display"=0, "Station Label Display"="", "Current Run Start Time Display"=0.0, "Board ID Display"="", "RPM Display"=0, "Current Display"=0.0, "Current Path Display"=path "", "Saving Display"=FALSE, "Unit Type Display"=enum."", "Total Time On Display"=0.0, "UI Button"=FALSE}}, {"Appliance Details"={"FileVersionInfo"={"FileVersion"="", "ProductName"="", "InternalName"="", "CompanyName"="", "LegalCopyright"="", "FileDescription"=""}, "Dishwasher Info"={"Open Cup Weight (gm):"=0.0, "Auto Cup Weight (gm):"=0.0, "Detergent-Dish:"="", "Inlet Temperature-Dish:"="", "Cycle Mode-Dish:"="", "Unit Control-Dish:"="", "Manufacturer-Dish:"=""}, "Washer Info"={"Hot Water Temperature (Fahrenheit):"="", "Cold Water Temperature (Fahrenheit):"="", "Capacity (cu.ft):"=0.0, "Initial Cloth Weight:"=0.0, "Cloth Lot:"=0, "Model Family:"="", "Program Name:"="", "Cycle Selection:"="", "Wash Temperature:"="", "Rinse Temperature:"="", "Load Size:"=""}, "File Name Output Array"=[], "Calibration Output Array"=[], "Appliance Common"={"Engineer:"="", "Model Number:"="", "Serial Number:"="", "Comments:"="", "Station ID:"="", "Technician:"="", "TR Number:"="", "Lab ID:"="", "Voltage:"="", "Water Pressure (PSI):"="", "Test Date:"="", "Computer Name:"="", "IP Address:"="", "Ambient RH:"="", "Frequency:"="", "Build:"="", "Filename:"="", "Test Type:"="", "Load Run #:"=0, "Ambient Temperature (F):"="", "File Path:"=path "", "Cycles Per Year"=60}, "Water Heater"={"Heating Mode:"=""}, "Dryer"={"Heat Setting:"="", "Washer Water Temperature (60 ± 5°F):"=60, "Water Hardness (PPM):"=17, "Dryness Setting:"="", "Dryer Type:"="", "Exhaust:"="", "Drying Cycle:"="", "Load Type:"="", "Nominal Load Weight"="", "Dryer Initial IMC Data"={"Measured IMC (lbs)"=7.0, "Actual Initial RMC (%)"=7.0, "RMC (Desired %)"=100.0, "Bone Dry Wt(lbs)"=7.0, "Tolerance(%)"=5.0, "Actual Final RMC (%)"=7.0, "CEF (lbf/kWh)"=0.0, "Minimum Weight (lbf)"=0.0, "Average Weight (lbf)"=0.0, "Maximum Weight (lbf)"=0.0, "Measured IMC In Range?"=FALSE, "Moisture Reduction Factor"=55.5, "Field Use Factor"=1.04, "Empty Dryer Cold Weigth"=0.0, "Energy Standard"=enum."D2-Automatic Dryer", "Weight Cloth (lbs)"=0.0, "Relative Moisture Content (%)"=0.0, "Relative Moisture Content - Avg (%)"=0.0}}}, "Display Data (RLT)"={"Status Color"=0, "Serial Number Display"="", "Cycle Count Display"=0, "Station Label Display"="", "Current Run Start Time Display"=0.0, "Board ID Display"="", "RPM Display"=0, "Current Display"=0.0, "Current Path Display"=path "", "Saving Display"=FALSE, "Unit Type Display"=enum."", "Total Time On Display"=0.0, "UI Button"=FALSE}}, {"Appliance Details"={"FileVersionInfo"={"FileVersion"="", "ProductName"="", "InternalName"="", "CompanyName"="", "LegalCopyright"="", "FileDescription"=""}, "Dishwasher Info"={"Open Cup Weight (gm):"=0.0, "Auto Cup Weight (gm):"=0.0, "Detergent-Dish:"="", "Inlet Temperature-Dish:"="", "Cycle Mode-Dish:"="", "Unit Control-Dish:"="", "Manufacturer-Dish:"=""}, "Washer Info"={"Hot Water Temperature (Fahrenheit):"="", "Cold Water Temperature (Fahrenheit):"="", "Capacity (cu.ft):"=0.0, "Initial Cloth Weight:"=0.0, "Cloth Lot:"=0, "Model Family:"="", "Program Name:"="", "Cycle Selection:"="", "Wash Temperature:"="", "Rinse Temperature:"="", "Load Size:"=""}, "File Name Output Array"=[], "Calibration Output Array"=[], "Appliance Common"={"Engineer:"="", "Model Number:"="", "Serial Number:"="", "Comments:"="", "Station ID:"="", "Technician:"="", "TR Number:"="", "Lab ID:"="", "Voltage:"="", "Water Pressure (PSI):"="", "Test Date:"="", "Computer Name:"="", "IP Address:"="", "Ambient RH:"="", "Frequency:"="", "Build:"="", "Filename:"="", "Test Type:"="", "Load Run #:"=0, "Ambient Temperature (F):"="", "File Path:"=path "", "Cycles Per Year"=60}, "Water Heater"={"Heating Mode:"=""}, "Dryer"={"Heat Setting:"="", "Washer Water Temperature (60 ± 5°F):"=60, "Water Hardness (PPM):"=17, "Dryness Setting:"="", "Dryer Type:"="", "Exhaust:"="", "Drying Cycle:"="", "Load Type:"="", "Nominal Load Weight"="", "Dryer Initial IMC Data"={"Measured IMC (lbs)"=7.0, "Actual Initial RMC (%)"=7.0, "RMC (Desired %)"=100.0, "Bone Dry Wt(lbs)"=7.0, "Tolerance(%)"=5.0, "Actual Final RMC (%)"=7.0, "CEF (lbf/kWh)"=0.0, "Minimum Weight (lbf)"=0.0, "Average Weight (lbf)"=0.0, "Maximum Weight (lbf)"=0.0, "Measured IMC In Range?"=FALSE, "Moisture Reduction Factor"=55.5, "Field Use Factor"=1.04, "Empty Dryer Cold Weigth"=0.0, "Energy Standard"=enum."D2-Automatic Dryer", "Weight Cloth (lbs)"=0.0, "Relative Moisture Content (%)"=0.0, "Relative Moisture Content - Avg (%)"=0.0}}}, "Display Data (RLT)"={"Status Color"=0, "Serial Number Display"="", "Cycle Count Display"=0, "Station Label Display"="", "Current Run Start Time Display"=0.0, "Board ID Display"="", "RPM Display"=0, "Current Display"=0.0, "Current Path Display"=path "", "Saving Display"=FALSE, "Unit Type Display"=enum."", "Total Time On Display"=0.0, "UI Button"=FALSE}}, {"Appliance Details"={"FileVersionInfo"={"FileVersion"="", "ProductName"="", "InternalName"="", "CompanyName"="", "LegalCopyright"="", "FileDescription"=""}, "Dishwasher Info"={"Open Cup Weight (gm):"=0.0, "Auto Cup Weight (gm):"=0.0, "Detergent-Dish:"="", "Inlet Temperature-Dish:"="", "Cycle Mode-Dish:"="", "Unit Control-Dish:"="", "Manufacturer-Dish:"=""}, "Washer Info"={"Hot Water Temperature (Fahrenheit):"="", "Cold Water Temperature (Fahrenheit):"="", "Capacity (cu.ft):"=0.0, "Initial Cloth Weight:"=0.0, "Cloth Lot:"=0, "Model Family:"="", "Program Name:"="", "Cycle Selection:"="", "Wash Temperature:"="", "Rinse Temperature:"="", "Load Size:"=""}, "File Name Output Array"=[], "Calibration Output Array"=[], "Appliance Common"={"Engineer:"="", "Model Number:"="", "Serial Number:"="", "Comments:"="", "Station ID:"="", "Technician:"="", "TR Number:"="", "Lab ID:"="", "Voltage:"="", "Water Pressure (PSI):"="", "Test Date:"="", "Computer Name:"="", "IP Address:"="", "Ambient RH:"="", "Frequency:"="", "Build:"="", "Filename:"="", "Test Type:"="", "Load Run #:"=0, "Ambient Temperature (F):"="", "File Path:"=path "", "Cycles Per Year"=60}, "Water Heater"={"Heating Mode:"=""}, "Dryer"={"Heat Setting:"="", "Washer Water Temperature (60 ± 5°F):"=60, "Water Hardness (PPM):"=17, "Dryness Setting:"="", "Dryer Type:"="", "Exhaust:"="", "Drying Cycle:"="", "Load Type:"="", "Nominal Load Weight"="", "Dryer Initial IMC Data"={"Measured IMC (lbs)"=7.0, "Actual Initial RMC (%)"=7.0, "RMC (Desired %)"=100.0, "Bone Dry Wt(lbs)"=7.0, "Tolerance(%)"=5.0, "Actual Final RMC (%)"=7.0, "CEF (lbf/kWh)"=0.0, "Minimum Weight (lbf)"=0.0, "Average Weight (lbf)"=0.0, "Maximum Weight (lbf)"=0.0, "Measured IMC In Range?"=FALSE, "Moisture Reduction Factor"=55.5, "Field Use Factor"=1.04, "Empty Dryer Cold Weigth"=0.0, "Energy Standard"=enum."D2-Automatic Dryer", "Weight Cloth (lbs)"=0.0, "Relative Moisture Content (%)"=0.0, "Relative Moisture Content - Avg (%)"=0.0}}}, "Display Data (RLT)"={"Status Color"=0, "Serial Number Display"="", "Cycle Count Display"=0, "Station Label Display"="", "Current Run Start Time Display"=0.0, "Board ID Display"="", "RPM Display"=0, "Current Display"=0.0, "Current Path Display"=path "", "Saving Display"=FALSE, "Unit Type Display"=enum."", "Total Time On Display"=0.0, "UI Button"=FALSE}}] {"Display Data (RLT)"."Current Display" format="%.2f"; "Display Data (RLT)"."Cycle Count Display" format="%04d"; "Appliance Details"."Dryer"."Dryer Initial IMC Data"."Maximum Weight (lbf)" format="%03_6g"; "Appliance Details"."Dryer"."Dryer Initial IMC Data"."Average Weight (lbf)" format="%03_6g"; "Appliance Details"."Dryer"."Dryer Initial IMC Data"."Minimum Weight (lbf)" format="%03_6g"; "Appliance Details"."Dryer"."Dryer Initial IMC Data"."CEF (lbf/kWh)" format="%03_6g"; "Appliance Details"."Dryer"."Dryer Initial IMC Data"."Actual Final RMC (%)" format="%03_6g"; "Appliance Details"."Dryer"."Dryer Initial IMC Data"."Tolerance(%)" format="%0#_6g"; "Appliance Details"."Dryer"."Dryer Initial IMC Data"."Bone Dry Wt(lbs)" format="%03_6g"; "Appliance Details"."Dryer"."Dryer Initial IMC Data"."RMC (Desired %)" format="%0#_6g"; "Appliance Details"."Dryer"."Dryer Initial IMC Data"."Actual Initial RMC (%)" format="%03_6g"; "Appliance Details"."Dryer"."Dryer Initial IMC Data"."Measured IMC (lbs)" format="%0#_6g"}
  out "Collecting Agilent Data":bool
  in  "Agilent Scan Rate (Seconds)":i32=3
  in  "Status Output Locations":path[](array[path])
  out "Time":string="Settings"
  in  "34972-1":refnum<visa-resource-name>="AGILENT_HCC"
  in  "Start DAQ Loop":bool
  in  "Update Status":i32=1000
  in  "Debug Tab":enum32{"Debug Info", "Parsed Current", "States"}(tab)
  in  "Disable Agilent Collection":bool
  out "Agilent Channels DAQ":string
  out "Current":dbl[](array[numeric])
  out "Raw Data (Scaled)":dbl[](array[numeric]) format="%.2f"
  out "Connected Board IDs":string[](array[string])
  out "Find Newfi Error":errorcluster
  out "Save Array":bool[](array[boolean])
  out "Disable Channel = True":bool[](array[boolean])
  out "Unsorted Data":dbl[](array[numeric]) format="%.2f"
  out "read buffer":string
  out "Voltage Indexes":i32[](array[numeric])
  out "Voltage":dbl[](array[numeric])
  in  "Debug":bool
  out "Main Loop":string[](array[string])
  out "DAQ Loop":string[](array[string])
  out "error out":errorcluster
  in  "error in (no error)":errorcluster
  out "Timer 2":dbl format="%<%H:%M:%S>t"
  in  "Connected Board ID's (Newfi)":string[](array[string])
  in  "Board Index":i32[](array[numeric])
  in  "Open Panel":T1={"Appliance Details"={"FileVersionInfo"={"FileVersion"="", "ProductName"="", "InternalName"="", "CompanyName"="", "LegalCopyright"="", "FileDescription"=""}, "Dishwasher Info"={"Open Cup Weight (gm):"=0.0, "Auto Cup Weight (gm):"=0.0, "Detergent-Dish:"="", "Inlet Temperature-Dish:"="", "Cycle Mode-Dish:"="", "Unit Control-Dish:"="", "Manufacturer-Dish:"=""}, "Washer Info"={"Hot Water Temperature (Fahrenheit):"="", "Cold Water Temperature (Fahrenheit):"="", "Capacity (cu.ft):"=0.0, "Initial Cloth Weight:"=0.0, "Cloth Lot:"=0, "Model Family:"="", "Program Name:"="", "Cycle Selection:"="", "Wash Temperature:"="", "Rinse Temperature:"="", "Load Size:"=""}, "File Name Output Array"=[], "Calibration Output Array"=[], "Appliance Common"={"Engineer:"="", "Model Number:"="", "Serial Number:"="", "Comments:"="", "Station ID:"="", "Technician:"="", "TR Number:"="", "Lab ID:"="", "Voltage:"="", "Water Pressure (PSI):"="", "Test Date:"="", "Computer Name:"="", "IP Address:"="", "Ambient RH:"="", "Frequency:"="", "Build:"="", "Filename:"="", "Test Type:"="", "Load Run #:"=0, "Ambient Temperature (F):"="", "File Path:"=path "", "Cycles Per Year"=60}, "Water Heater"={"Heating Mode:"=""}, "Dryer"={"Heat Setting:"="", "Washer Water Temperature (60 ± 5°F):"=60, "Water Hardness (PPM):"=17, "Dryness Setting:"="", "Dryer Type:"="", "Exhaust:"="", "Drying Cycle:"="", "Load Type:"="", "Nominal Load Weight"="", "Dryer Initial IMC Data"={"Measured IMC (lbs)"=7.0, "Actual Initial RMC (%)"=7.0, "RMC (Desired %)"=100.0, "Bone Dry Wt(lbs)"=7.0, "Tolerance(%)"=5.0, "Actual Final RMC (%)"=7.0, "CEF (lbf/kWh)"=0.0, "Minimum Weight (lbf)"=0.0, "Average Weight (lbf)"=0.0, "Maximum Weight (lbf)"=0.0, "Measured IMC In Range?"=FALSE, "Moisture Reduction Factor"=55.5, "Field Use Factor"=1.04, "Empty Dryer Cold Weigth"=0.0, "Energy Standard"=enum."D2-Automatic Dryer", "Weight Cloth (lbs)"=0.0, "Relative Moisture Content (%)"=0.0, "Relative Moisture Content - Avg (%)"=0.0}}}, "Display Data (RLT)"={"Status Color"=0, "Serial Number Display"="", "Cycle Count Display"=0, "Station Label Display"="", "Current Run Start Time Display"=0.0, "Board ID Display"="", "RPM Display"=0, "Current Display"=0.0, "Current Path Display"=path "", "Saving Display"=FALSE, "Unit Type Display"=enum."", "Total Time On Display"=0.0, "UI Button"=FALSE}} {"Display Data (RLT)"."Current Display" format="%.2f"; "Display Data (RLT)"."Cycle Count Display" format="%04d"; "Appliance Details"."Dryer"."Dryer Initial IMC Data"."Maximum Weight (lbf)" format="%03_6g"; "Appliance Details"."Dryer"."Dryer Initial IMC Data"."Average Weight (lbf)" format="%03_6g"; "Appliance Details"."Dryer"."Dryer Initial IMC Data"."Minimum Weight (lbf)" format="%03_6g"; "Appliance Details"."Dryer"."Dryer Initial IMC Data"."CEF (lbf/kWh)" format="%03_6g"; "Appliance Details"."Dryer"."Dryer Initial IMC Data"."Actual Final RMC (%)" format="%03_6g"; "Appliance Details"."Dryer"."Dryer Initial IMC Data"."Tolerance(%)" format="%0#_6g"; "Appliance Details"."Dryer"."Dryer Initial IMC Data"."Bone Dry Wt(lbs)" format="%03_6g"; "Appliance Details"."Dryer"."Dryer Initial IMC Data"."RMC (Desired %)" format="%0#_6g"; "Appliance Details"."Dryer"."Dryer Initial IMC Data"."Actual Initial RMC (%)" format="%03_6g"; "Appliance Details"."Dryer"."Dryer Initial IMC Data"."Measured IMC (lbs)" format="%0#_6g"}
  # "Washer Reliability"
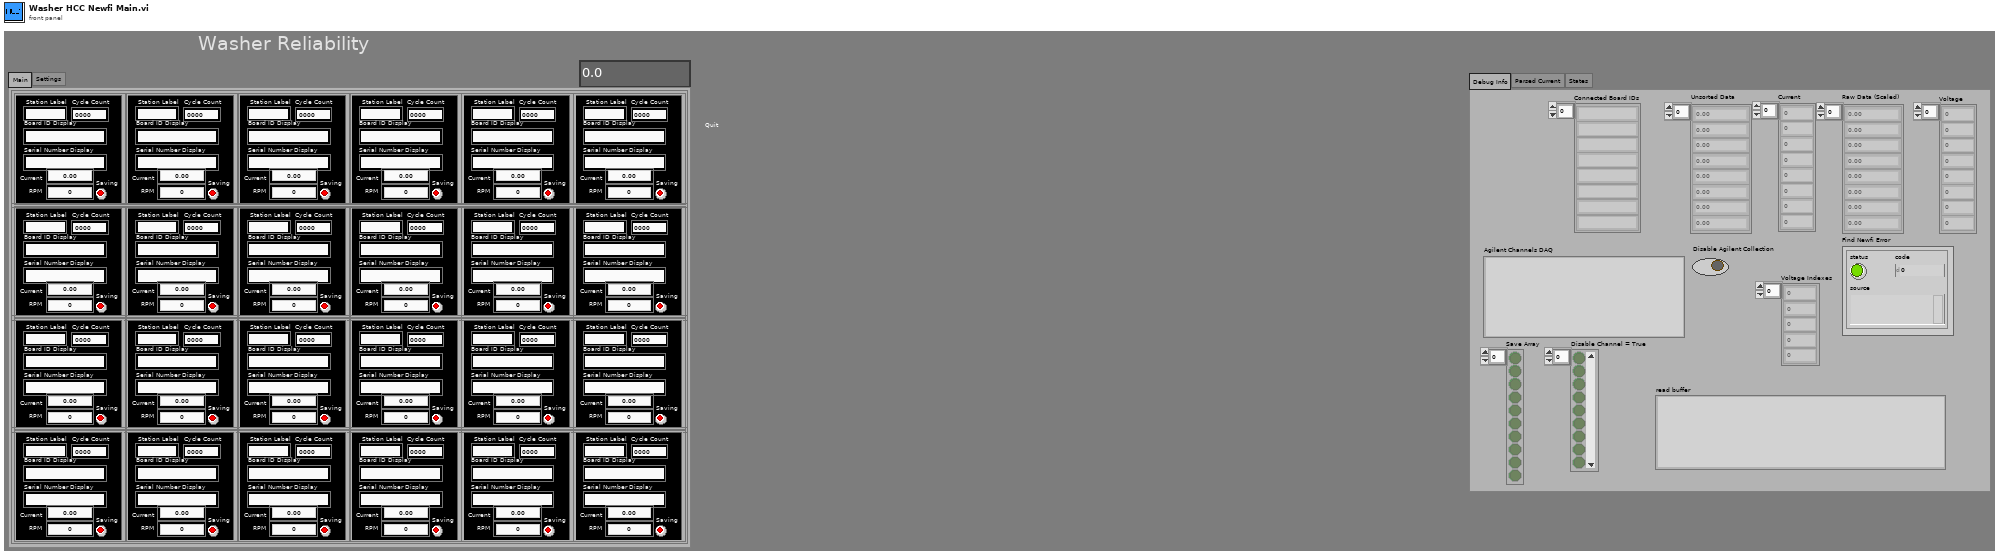
[diagram p1: front panel]
types:
  T1 = typedef "Save File.lvlib/Save File Washer.ctl" = cluster{"Appliance Details":T2, "Display Data (RLT)":T8}
  T2 = typedef "File Setup.lvlib/Save File DISH Dishwasher Details.ctl" = cluster{"FileVersionInfo":T3, "Dishwasher Info":cluster{"Open Cup Weight (gm):":dbl, "Auto Cup Weight (gm):":dbl, "Detergent-Dish:":string, "Inlet Temperature-Dish:":string, "Cycle Mode-Dish:":string, "Unit Control-Dish:":string, "Manufacturer-Dish:":string}, "Washer Info":cluster{"Hot Water Temperature (Fahrenheit):":string, "Cold Water Temperature (Fahrenheit):":string, "Capacity (cu.ft):":dbl, "Initial Cloth Weight:":dbl, "Cloth Lot:":i32, "Model Family:":string, "Program Name:":string, "Cycle Selection:":string, "Wash Temperature:":string, "Rinse Temperature:":string, "Load Size:":string}, "File Name Output Array":string[][], "Calibration Output Array":string[][], "Appliance Common":T4, "Water Heater":cluster{"Heating Mode:":string}, "Dryer":cluster{"Heat Setting:":T5, "Washer Water Temperature (60 ± 5°F):":u16, "Water Hardness (PPM):":u16, "Dryness Setting:":T5, "Dryer Type:":string, "Exhaust:":string, "Drying Cycle:":string, "Load Type:":string, "Nominal Load Weight":string, "Dryer Initial IMC Data":T6}}
  T3 = typedef "FileVersionInformation.ctl" = cluster{"FileVersion":string, "ProductName":string, "InternalName":string, "CompanyName":string, "LegalCopyright":string, "FileDescription":string}
  T4 = typedef "DOE Appliance Common.ctl" = cluster{"Engineer:":string, "Model Number:":string, "Serial Number:":string, "Comments:":string, "Station ID:":string, "Technician:":string, "TR Number:":string, "Lab ID:":string, "Voltage:":string, "Water Pressure (PSI):":string, "Test Date:":string, "Computer Name:":string, "IP Address:":string, "Ambient RH:":string, "Frequency:":string, "Build:":string, "Filename:":string, "Test Type:":string, "Load Run #:":i32, "Ambient Temperature (F):":string, "File Path:":path, "Cycles Per Year":u32}
  T5 = typedef "Custom Pallet String.ctl" = string
  T6 = typedef "DPT IMC Data.ctl" = cluster{"Measured IMC (lbs)":dbl, "Actual Initial RMC (%)":dbl, "RMC (Desired %)":dbl, "Bone Dry Wt(lbs)":dbl, "Tolerance(%)":dbl, "Actual Final RMC (%)":dbl, "CEF (lbf/kWh)":dbl, "Minimum Weight (lbf)":dbl, "Average Weight (lbf)":dbl, "Maximum Weight (lbf)":dbl, "Measured IMC In Range?":bool, "Moisture Reduction Factor":dbl, "Field Use Factor":dbl, "Empty Dryer Cold Weigth":dbl, "Energy Standard":T7, "Weight Cloth (lbs)":dbl, "Relative Moisture Content (%)":dbl, "Relative Moisture Content - Avg (%)":dbl}
  T7 = typedef "DOE Dryer Standard.ctl" = enum16{"D2-Automatic Dryer", "D2-Timer Dryer", "D1-Automatic Dryer", "D1-Timer Dryer", "Other"}
  T8 = typedef "Save File Appliance Display.ctl" = cluster{"Status Color":u32, "Serial Number Display":string, "Cycle Count Display":i32, "Station Label Display":string, "Current Run Start Time Display":dbl, "Board ID Display":string, "RPM Display":u32, "Current Display":dbl, "Current Path Display":path, "Saving Display":bool, "Unit Type Display":T9, "Total Time On Display":dbl, "UI Button":bool}
  T9 = typedef "Save File.lvlib/Save File Unit Type.ctl" = enum32{"", "Viper", "Hawk", "2015"}
  T10 = typedef "HCC Station Group.ctl" = enum16{"Station 1-6", "Station 7-12", "Station 13-18", "Station 19-24"}
  T11 = enum32{"invalid app kind", "Development System", "Run Time System", "Student Edition", "Embedded LabVIEW", "Evaluation", "Custom"}
  T12 = cluster{"Current VI Reference":refnum<vi>, "Close Panel on Exit?":bool}
  T13 = enum32{"Invalid", "Standard", "Closed", "Hidden", "Minimized", "Maximized"}
  T14 = cluster{"Core":cluster{"Current VI Reference":refnum<vi>, "Close Panel on Exit?":bool}, "Open Panel":T1, "Array":T1[], "Array 2":T1[], "Array 3":T1[], "Array 4":T1[], "Status Output Locations":path[], "Board Index":i32[], "Connected Board ID's (Newfi)":string[], "Agilent Channels":string, "Start DAQ Loop":bool, "Station IDs":string[], "Network Var Set":u8}
  T15 = cluster{"34972-1":refnum<visa-resource-name>, "Agilent Scan Rate (Seconds)":i32, "Current":dbl[], "Voltage":dbl[], "Agilent Channels DAQ":string}
  T16 = typedef "File Setup.lvlib/Save File DOE File Path Control.ctl" = cluster{"General Setup Paths":cluster{"Calibration File Path":path, "DOE Capacity Path":path, "Data Folder Path":path, "RLT Backup Data Path":path, "Tool Base Path":path, "General Startup Config Path":path, "File Save Previous Run Path":path, "File Save Configuration Data Path":path}, "Data File Paths":T17, "New Summary Created":bool, "Check Location Interval (Second)":i32}
  T17 = typedef "File Setup.lvlib/Save File DOE Data Save Filepaths.ctl" = cluster{"Data File Path":path, "Debug File Path":path, "Bus Log Path":path, "Current":path, "Summary":path}
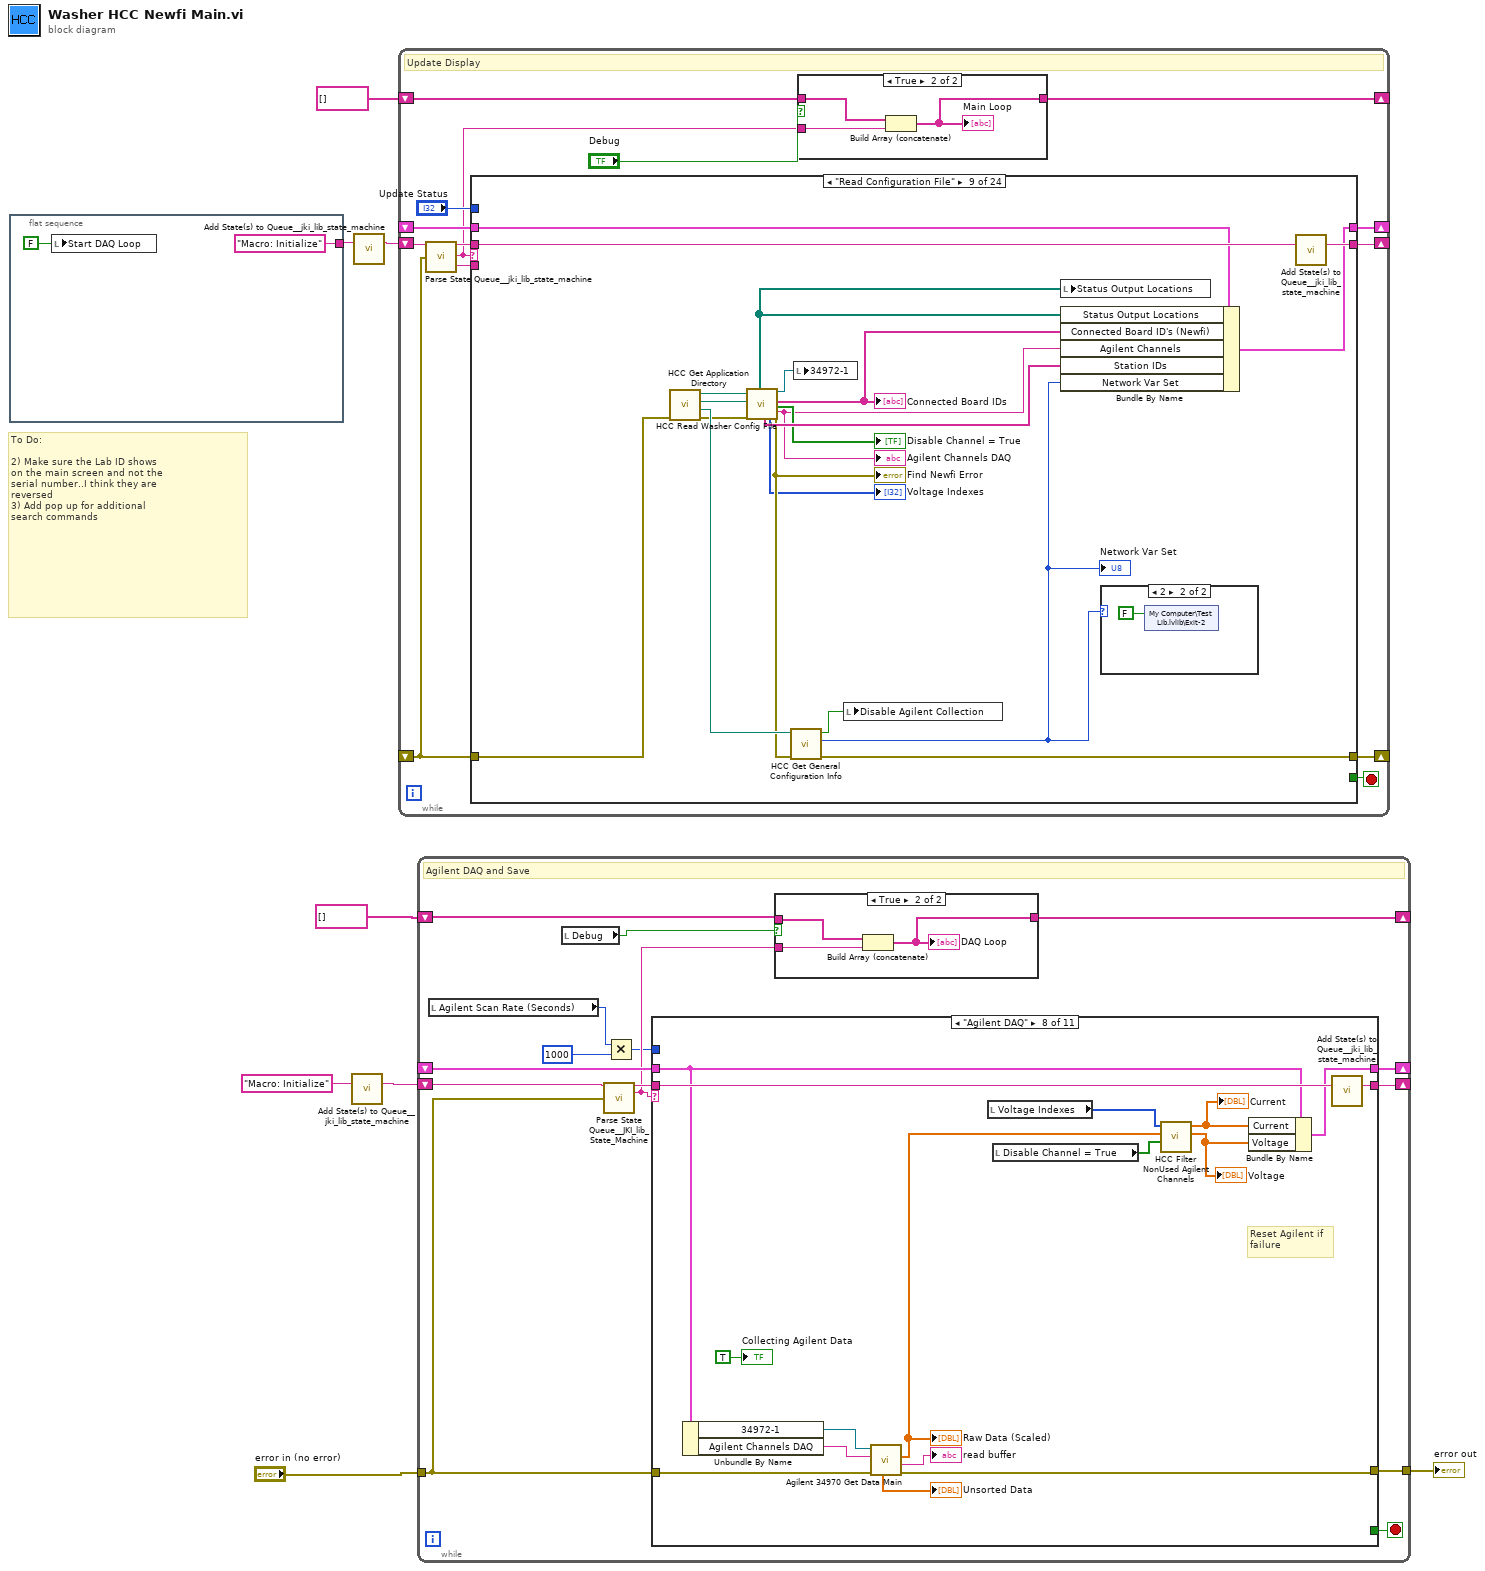
[diagram p0: block diagram]
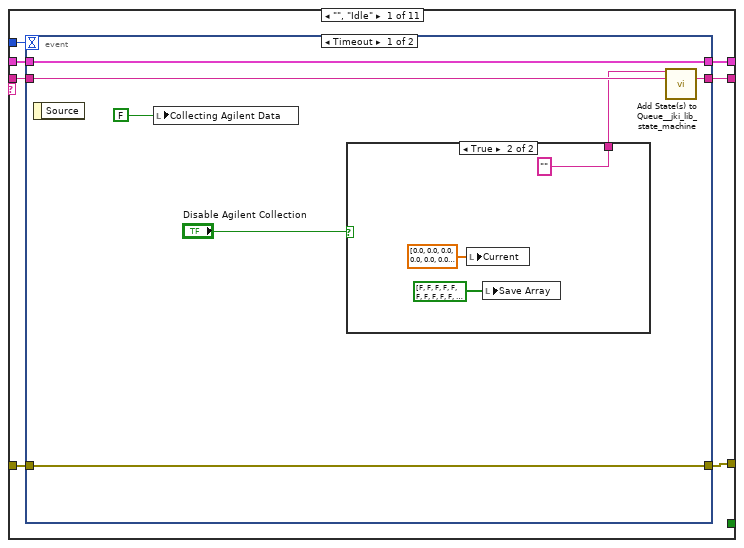
[diagram p3: hidden frame]
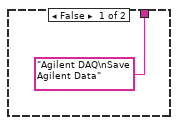
[diagram p4: hidden frame]
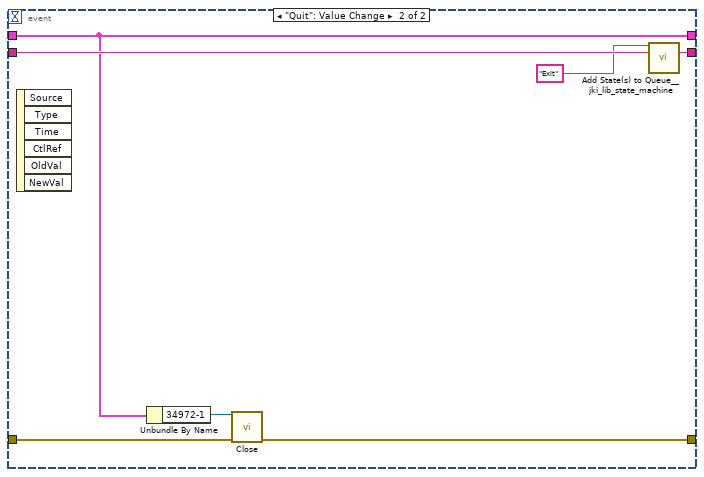
[diagram p5: hidden frame]
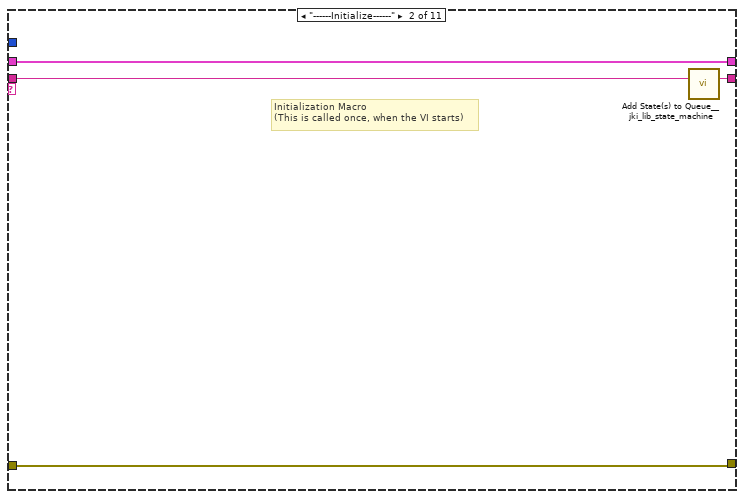
[diagram p6: hidden frame]
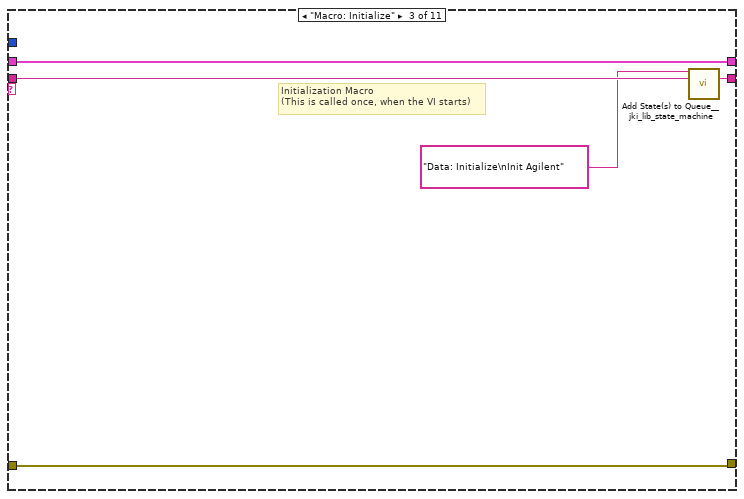
[diagram p7: hidden frame]
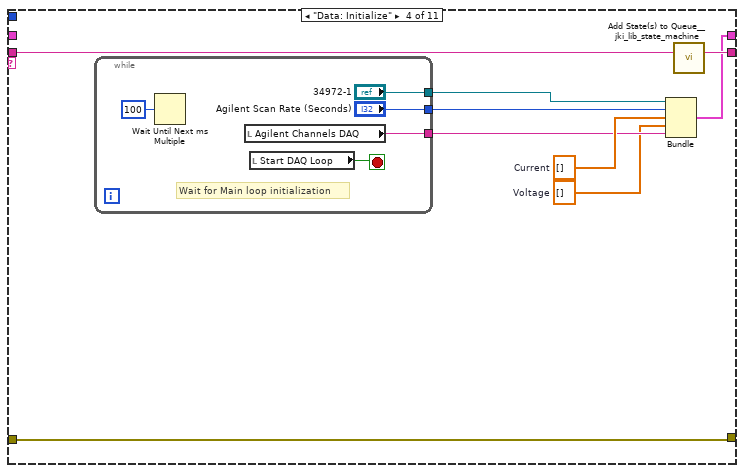
[diagram p8: hidden frame]
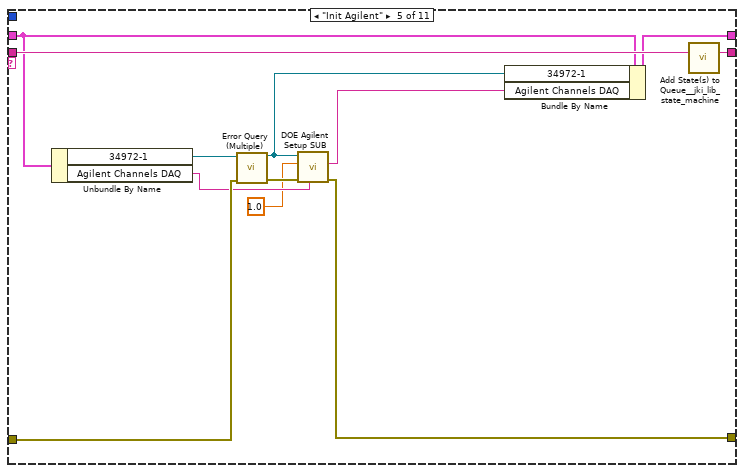
[diagram p9: hidden frame]
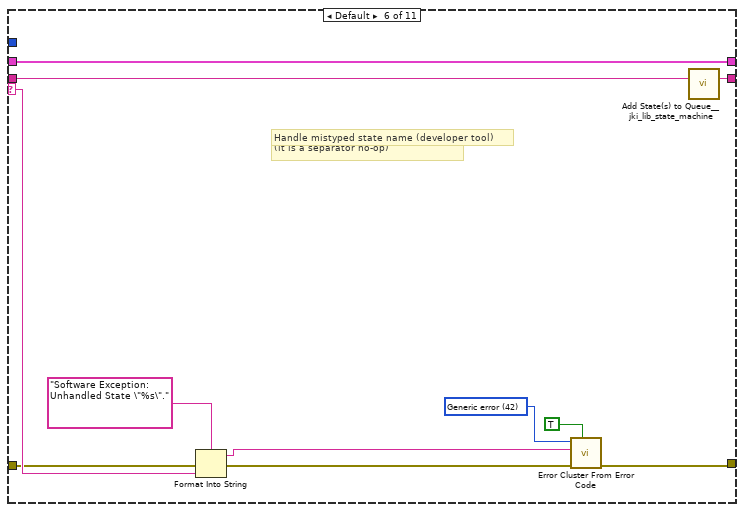
[diagram p10: hidden frame]
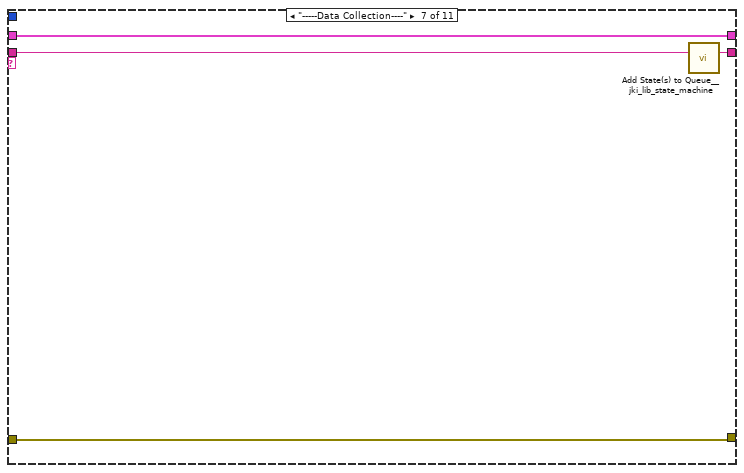
[diagram p11: hidden frame]
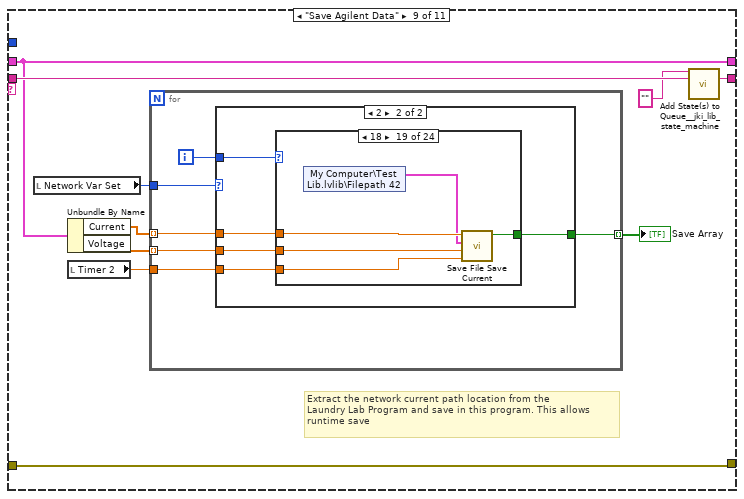
[diagram p12: hidden frame]
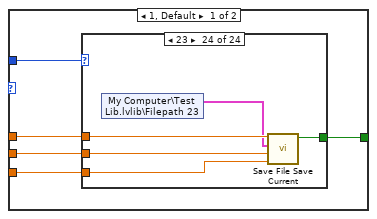
[diagram p13: hidden frame]
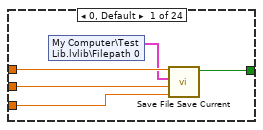
[diagram p14: hidden frame]
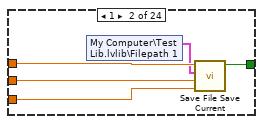
[diagram p15: hidden frame]
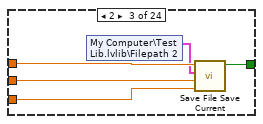
[diagram p16: hidden frame]
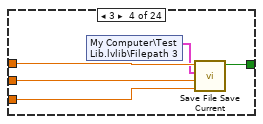
[diagram p17: hidden frame]
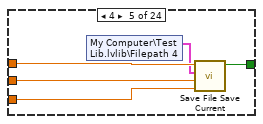
[diagram p18: hidden frame]
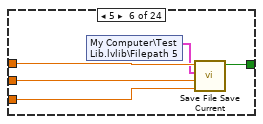
[diagram p19: hidden frame]
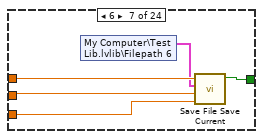
[diagram p20: hidden frame]
diagram:
  # "To Do:\n\n2) Make sure the Lab ID shows\non the main screen and not the \nserial number..I think they are \nreversed\n3) Add pop up for additional\nsearch commands"
  n1 = flat-sequence {
    tunnel: ["Macro: Initialize"] -> w5
    frame #0 {
      n2 = local write "Start DAQ Loop"(FALSE ("Start DAQ Loop")) -> ()
    }
  }
  n3 = call <vilib>:"Add State(s) to Queue__jki_lib_state_machine.vi"("State(s) in (\"\")"="Macro: Initialize") -> ("States Out"=w4:string)  [unwired: 14 in]
  n4 = call <vilib>:"Add State(s) to Queue__jki_lib_state_machine.vi"("State(s) in (\"\")"=w5) -> ("States Out"=w8:string)  [unwired: 14 in]
  n5 = while "Update Display" {
    shift-right: [w18] -> _
    shift-left: _ -> [w17]
    shift-right: [w21] -> _
    shift-left: _ -> [w16]
    shift-right: [w20] -> _
    shift-left: w8 -> [w22]
    shift-right: [w11] -> _
    shift-left: string[] [] -> [w13]
    stop <- w19 stop-if-true
    # "Update Display"
    n6 = call <vilib>:"Parse State Queue__jki_lib_state_machine.vi"("State Queue"=w22, "Error In (no error)"=w16) -> ("Remaining States"=w24:string, "Current State"=w12:string, "Arguments"=w23:string)  [unwired: 11 in]
    n7 = case shown="\"Read Configuration File\"" w12 {
      selector: w12 -> [_ _ w155 _ _ _ _ _ _ _ _ _ _ _ _ _ _ _ _ _ _ _ _ _]
      tunnel: w24 -> [w35 w154 w159 w177 w183 w188 w192 w209 w227 w255 w274 w278 w285 w299 w311 w337 w342 w352 w356 w369 w385 w401 w416 w422]
      tunnel: w23 -> [_ _ _ _ _ _ _ _ _ _ _ _ _ w294 w305 _ _ _ _ _ _ _ _ _]
      tunnel: w17 -> [w33 w151 w157 w168 w180 w186 w189 _ w226 w253 w269 w275 w279 w297 w307 w334 w339 w349 w353 w371 w387 w403 w419 w425]
      tunnel: [w32 w152 w161 w174 errorcluster {"status"=FALSE, "code"=0, "source"=""} ("error out") w185 w190 w206 w217 w254 w270 w276 w282 w295 w308 w335 w340 w350 w354 w362 w378 w394 w410 w424] -> w21
      tunnel: w16 -> [w31 w152 w160 w174 w179 w185 w190 w206 w212 w254 w271 w276 w283 w296 w309 w335 w340 w350 w354 w360 w376 w392 w408 w424]
      tunnel: [w34 w153 w158 w176 w182 w187 w191 w208 w229 w256 w273 w277 w284 w298 w310 w336 w341 w351 w355 w372 w388 w404 w420 w426] -> w20
      tunnel: [_ _ _ _ _ TRUE _ _ _ _ _ _ _ _ _ _ _ _ _ _ _ _ _ _] -> w19
      tunnel: [w30 w151 w157 w175 w180 w186 w189 w207 w225 w252 w269 w275 w280 w297 w307 w334 w339 w349 w353 w370 w386 w402 w418 w425] -> w18
      tunnel: "Update Status" -> [w29 _ _ _ _ _ _ _ _ _ _ _ _ _ _ _ _ _ _ _ _ _ _ _]
      frame "", "Idle" {
        # "This will tell which\nfile location to open (GEA2 or 2015)"
        n8 = event shown="[2] \"Array\": Value Change" {
          selector: _ -> [_ _ _ _ _ _ _]
          dyn-events: _ -> [_ _ _ _ _ _ _]
          timeout: w29 -> [_ _ _ _ _ _ _]
          tunnel: w35 -> [w41 w50 w69 w92 w115 w138 w150]
          tunnel: [w40 w49 w68 w91 w114 w137 w149] -> w34
          tunnel: w33 -> [w38 w43 w66 w87 w110 w133 w147]
          tunnel: [w39 w45 w64 w84 w107 w126 w148] -> w32
          tunnel: w31 -> [w39 w46 w59 w86 w109 w132 w148]
          tunnel: [w38 w43 w67 w89 w112 w135 w147] -> w30
          event Timeout {
            n9 = event-data() -> ()  [unwired: 1 in, 1 out]
            n10 = call "UTILITY E-Time.vi"() -> ("Elapsed Time (sec)"=→"Timer 2":dbl)  [unwired: 9 in, 2 out]
            n11 = call <vilib>:"Add State(s) to Queue__jki_lib_state_machine.vi"("State(s) in Front (\"\")"="Update Status 1\nUpdate Status 2\nUpdate Status 3\nUpdate Status 4", "State(s) in (\"\")"=w41) -> ("States Out"=w40:string)  [unwired: 13 in]
          }
          event "Quit": Value Change {
            n12 = event-data() -> ()  [unwired: 1 in, 1 out]
            n13 = Unbundle By Name(w43) -> ("Network Var Set"=w42:u8)
            n14 = case shown="1, Default" w42 {
              tunnel: "Quit" -> [w51 w52]
              frame 1, Default {
                n15 = shared-variable "My Computer\\Test Lib.lvlib\\Exit"(w51) -> ()  [unwired: 1 in, 1 out]
              }
              frame 2 {
                n16 = shared-variable "My Computer\\Test Lib.lvlib\\Exit-2"(w52) -> ()  [unwired: 1 in, 1 out]
              }
            }
            n17 = call "UTILITY Delay mS.vi"("Error In"=w46, "milliseconds to wait"=u32 6000) -> ("Error Out"=w45:errorcluster)  [unwired: 13 in]
            n18 = call <vilib>:"Add State(s) to Queue__jki_lib_state_machine.vi"("State(s) in Front (\"\")"="Macro: Exit", "State(s) in (\"\")"=w50) -> ("States Out"=w49:string)  [unwired: 13 in]
          }
          event "Array": Value Change {
            # "Search for which button has been\npressed"
            n19 = event-data() -> ("NewVal"=w57:T1[])  [unwired: 1 in, 5 out]
            n20 = Unbundle By Name(w66) -> ("Open Panel"=w65:T1, "Connected Board ID's (Newfi)"=w62:string[], "Status Output Locations"=w61:path[])
            n21 = for {
              tunnel: w57 -> [w75] mode=indexing
              tunnel: [w73] -> w60
              shift-right: [w71] -> w58
              shift-left: w59 -> [w71]
              tunnel: [w70] -> w56 mode=indexing
              i -> [w73]
              stop <- w72 stop-if-true
              n22 = Unbundle By Name(w75) -> ("Display Data (RLT).UI Button"=w70:bool)
              n23 = Equal?(x=w70, y=TRUE) -> (x = y?=w72:bool)
            }
            n24 = Or Array Elements(Boolean array=w56) -> (logical OR=w55:bool)
            n25 = call "HCC Open EXE Handle.vi"("Status Output Locations"=w61, "Connected Board ID's (Newfi)"=w62, "Open Panel"=w65, "Station Group"=HCC_Station_Group."Station 1-6", "NewVal"=w57, "True Or False Event? (Trigger on True)"=w55, "error in (no error)"=w58, "Exe Number"=w60) -> ("Output"=w54:T1, "error out"=w64:errorcluster)  [unwired: 6 in]
            n26 = Bundle By Name(cluster=w66, "Open Panel"=w54) -> (w67:T14)
            n27 = call <vilib>:"Add State(s) to Queue__jki_lib_state_machine.vi"("State(s) in Front (\"\")"="Open Newfi Panel", "State(s) in (\"\")"=w69) -> ("States Out"=w68:string)  [unwired: 13 in]
          }
          event "Array 2": Value Change {
            # "Search for which button has been\npressed"
            n28 = event-data() -> ("NewVal"=w79:T1[])  [unwired: 1 in, 5 out]
            n29 = Unbundle By Name(w87) -> ("Open Panel"=w80:T1, "Connected Board ID's (Newfi)"=w81:string[], "Status Output Locations"=w82:path[])  [unwired: 1 out]
            n30 = for {
              tunnel: w79 -> [w98] mode=indexing
              tunnel: [w95] -> w77
              tunnel: [w94] -> w88 mode=indexing
              shift-right: [w93] -> w85
              shift-left: w86 -> [w93]
              i -> [w95]
              stop <- w96 stop-if-true
              n31 = Unbundle By Name(w98) -> ("Display Data (RLT).UI Button"=w94:bool)
              n32 = Equal?(x=w94, y=TRUE) -> (x = y?=w96:bool)
            }
            n33 = Or Array Elements(Boolean array=w88) -> (logical OR=w78:bool)
            n34 = call "HCC Open EXE Handle.vi"("Status Output Locations"=w82, "Connected Board ID's (Newfi)"=w81, "Open Panel"=w80, "Station Group"=HCC_Station_Group."Station 7-12", "NewVal"=w79, "True Or False Event? (Trigger on True)"=w78, "error in (no error)"=w85, "Exe Number"=w77) -> ("Output"=w83:T1, "error out"=w84:errorcluster)  [unwired: 6 in]
            n35 = call <vilib>:"Add State(s) to Queue__jki_lib_state_machine.vi"("State(s) in Front (\"\")"="Open Newfi Panel", "State(s) in (\"\")"=w92) -> ("States Out"=w91:string)  [unwired: 13 in]
            n36 = Bundle By Name(cluster=w87, "Open Panel"=w83) -> (w89:T14)
          }
          event "Array 3": Value Change {
            # "Search for which button has been\npressed"
            n37 = event-data() -> ("NewVal"=w102:T1[])  [unwired: 1 in, 5 out]
            n38 = for {
              tunnel: w102 -> [w121] mode=indexing
              tunnel: [w118] -> w100
              tunnel: [w117] -> w111 mode=indexing
              shift-right: [w116] -> w108
              shift-left: w109 -> [w116]
              i -> [w118]
              stop <- w119 stop-if-true
              n39 = Unbundle By Name(w121) -> ("Display Data (RLT).UI Button"=w117:bool)
              n40 = Equal?(x=w117, y=TRUE) -> (x = y?=w119:bool)
            }
            n41 = Unbundle By Name(w110) -> ("Open Panel"=w104:T1, "Connected Board ID's (Newfi)"=w105:string[], "Status Output Locations"=w106:path[])
            n42 = Or Array Elements(Boolean array=w111) -> (logical OR=w101:bool)
            n43 = call "HCC Open EXE Handle.vi"("Status Output Locations"=w106, "Connected Board ID's (Newfi)"=w105, "Open Panel"=w104, "Station Group"=HCC_Station_Group."Station 13-18", "NewVal"=w102, "True Or False Event? (Trigger on True)"=w101, "error in (no error)"=w108, "Exe Number"=w100) -> ("Output"=w103:T1, "error out"=w107:errorcluster)  [unwired: 6 in]
            n44 = Bundle By Name(cluster=w110, "Open Panel"=w103) -> (w112:T14)
            n45 = call <vilib>:"Add State(s) to Queue__jki_lib_state_machine.vi"("State(s) in Front (\"\")"="Open Newfi Panel", "State(s) in (\"\")"=w115) -> ("States Out"=w114:string)  [unwired: 13 in]
          }
          event "Array 4": Value Change {
            # "Search for which button has been\npressed"
            n46 = event-data() -> ("NewVal"=w125:T1[])  [unwired: 1 in, 5 out]
            n47 = Unbundle By Name(w133) -> ("Open Panel"=w128:T1, "Connected Board ID's (Newfi)"=w129:string[], "Status Output Locations"=w130:path[])
            n48 = for {
              tunnel: w125 -> [w144] mode=indexing
              tunnel: [w141] -> w123
              tunnel: [w140] -> w134 mode=indexing
              shift-right: [w139] -> w131
              shift-left: w132 -> [w139]
              i -> [w141]
              stop <- w142 stop-if-true
              n49 = Unbundle By Name(w144) -> ("Display Data (RLT).UI Button"=w140:bool)
              n50 = Equal?(x=w140, y=TRUE) -> (x = y?=w142:bool)
            }
            n51 = Or Array Elements(Boolean array=w134) -> (logical OR=w124:bool)
            n52 = call "HCC Open EXE Handle.vi"("Status Output Locations"=w130, "Connected Board ID's (Newfi)"=w129, "Open Panel"=w128, "Station Group"=HCC_Station_Group."Station 19-24", "NewVal"=w125, "True Or False Event? (Trigger on True)"=w124, "error in (no error)"=w131, "Exe Number"=w123) -> ("Output"=w127:T1, "error out"=w126:errorcluster)  [unwired: 6 in]
            n53 = Bundle By Name(cluster=w133, "Open Panel"=w127) -> (w135:T14)
            n54 = call <vilib>:"Add State(s) to Queue__jki_lib_state_machine.vi"("State(s) in Front (\"\")"="Open Newfi Panel", "State(s) in (\"\")"=w138) -> ("States Out"=w137:string)  [unwired: 13 in]
          }
          event Panel Close? {
            n55 = event-data() -> ()  [unwired: 1 in, 1 out]
            n56 = call <vilib>:"Add State(s) to Queue__jki_lib_state_machine.vi"("State(s) in Front (\"\")"="Macro: Exit", "State(s) in (\"\")"=w150) -> ("States Out"=w149:string)  [unwired: 13 in]
            n57 = event-data("Discard?"=TRUE) -> ()  [unwired: 1 in, 1 out]
          }
        }
      }
      frame "---------- Core ----------" {
        n58 = call <vilib>:"Add State(s) to Queue__jki_lib_state_machine.vi"("State(s) in (\"\")"=w154) -> ("States Out"=w153:string)  [unwired: 14 in]
      }
      frame Default {
        w164 = 42 items=["No error", "Argument error", "Memory is full", "Out of zone", "End of file", "File already open", "Generic file I/O error", "File not found", "File permission error", "Disk is full", "Duplicate path", "Too many files open", "System feature not enabled", "Resource file not found", "Cannot add resource", "Resource not found", "Image not found", "Image memory error", "Pen does not exist", "Config type invalid", "Config token not found", "Config parse error", "Config memory error", "Bad external code format", "Bad external code offset", "External code not present", "Null window", "Destroy window error", "Null menu", "Print aborted", "Bad print record", "Print driver error", "Windows error during printing", "Memory error during printing", "Print dialog error", "Generic print error", "Invalid device refnum", "Device not found", "Device parameter error", "Device unit error", "Cannot open device", "Device call aborted", "Generic error", "Cancelled by user", "Object ID too low", "Object ID too high", "Object not in heap", "Unknown heap", "Unknown object (invalid DefProc)", "Unknown object (DefProc not in table)", "Message out of range", "Invalid (null) method", "Unknown message", "Manager call not supported", "Bad address", "Network operation in progress", "Network operation timed out", "Connection is busy", "Network attribute not supported", "Network error", "Address in use", "System out of memory", "Connection aborted", "Connection refused", "Not connected", "Already connected", "Connection closed", "Initialization error (interapplication manager)", "Bad occurrence", "Wait on unbound occurrence handler", "Occurrence queue overflow", "Datalog type conflict", "Unused", "Unrecognized type (interapplication manager)", "Memory corrupt", "Failed to make temporary DLL", "Old CIN version", "Drag socket not found", "Failed to load drop-object", "Failed to register OLE object", "Failed to release OLE object", "Format specifier type mismatch", "Unknown format specifier", "Too few format specifiers", "Too many format specifiers", "Scan failed", "Newer CIN version", "Error converting to variant", "Runtime menu error", "Password tampered", "Variant attribute not found", "Incompatible variant data type", "Event data is not available", "Event Store is not present", "Occurrence is not found", "Event Queue is not created", "Event info is not available", "Refnum passed is NULL", "Error retrieving Class GUID", "Error retrieving CoClass GUID", "Error retrieving TypeLib GUID.", "Bad built application magic bytes.", "Specific driver is different from the specific driver associated with the Logical Name.", "There is no session opened to the class driver.", "Max Error", "MAX - Error with config objects", "MAX - Error loading configuration", "MAX - Group not supported"]
        # "Current State"
        # "Handle mistyped state name (developer tool)"
        n59 = Format Into String(format string="Software Exception: Unhandled State \"%s\"." ("message"), error in=w160, w155) -> (resulting string=w163:string, error out=w162:errorcluster)  [unwired: 1 in]
        n60 = call <vilib>:"Error Cluster From Error Code.vi"("show call chain? (False)"=TRUE, "error in (no error)"=w162, "error message (\"\")"=w163, "error code (0)"=w164) -> ("error out"=w161:errorcluster)  [unwired: 5 in]
        n61 = call <vilib>:"Add State(s) to Queue__jki_lib_state_machine.vi"("State(s) in (\"\")"=w159) -> ("States Out"=w158:string)  [unwired: 14 in]
      }
      frame "Initialize Core Data" {
        # "originally closed?"
        # "exe?"
        # "If panel starts closed or is an EXE, then close it when we exit"
        n62 = property class="VI"() -> ("Front Panel.Open"=w173:bool)  [unwired: 2 in, 2 out]
        n63 = property class="App"() -> ("App.Kind"=w172:T11)  [unwired: 2 in, 2 out]
        n64 = control-ref of="Current VI Reference"() -> (w166:refnum<vi>)
        n65 = Not(x=w173) -> (.not. x?=w170:bool)
        n66 = Equal?(x=w172, y=T11."Run Time System" ("Application:Kind")) -> (x = y?=w169:bool)
        n67 = Or(x=w170, y=w169) -> (x .or. y?=w167:bool)
        n68 = Bundle By Name(cluster=w168, "Core.Current VI Reference"=w166, "Core.Close Panel on Exit?"=w167) -> (w175:T14)
        n69 = call <vilib>:"Add State(s) to Queue__jki_lib_state_machine.vi"("State(s) in (\"\")"=w177) -> ("States Out"=w176:string)  [unwired: 14 in]
      }
      frame "Error Handler" {
        # "Unhandled Error -- Display it"
        # "Handle any errors here.\nYou can also output any states to clean-up after errors occur"
        # "Clear error"
        n70 = call <vilib>:"General Error Handler.vi"("error in (no error)"=w179) -> ()  [unwired: 10 in, 5 out]
        n71 = call <vilib>:"Add State(s) to Queue__jki_lib_state_machine.vi"("State(s) in Front (\"\")"="/* Post Error States", "State(s) in (\"\")"=w183) -> ("States Out"=w182:string)  [unwired: 13 in]
      }
      frame "Exit" {
        n72 = call <vilib>:"Add State(s) to Queue__jki_lib_state_machine.vi"("State(s) in (\"\")"=w188) -> ("States Out"=w187:string)  [unwired: 14 in]
      }
      frame "---------- Data ----------" {
        # "Do not put any code in this frame.\n(It is a separator no-op. You can make a copy of this frame to create a new Data frame)"
        n73 = call <vilib>:"Add State(s) to Queue__jki_lib_state_machine.vi"("State(s) in (\"\")"=w192) -> ("States Out"=w191:string)  [unwired: 14 in]
      }
      frame "Data: Initialize" {
        w193 = u8 1  # Network Var Set
        w199 = string[] []  # Station IDs
        w201 = ""  # Agilent Channels
        n74 = call <vilib>:"Add State(s) to Queue__jki_lib_state_machine.vi"("State(s) in (\"\")"=w209) -> ("States Out"=w208:string)  [unwired: 14 in]
        n75 = Bundle("Core"=T12 {"Current VI Reference"=refnum, "Close Panel on Exit?"=FALSE}, "Open Panel"="Open Panel", "Array"="Array", "Array 2"="Array 2", "Array 3"="Array 3", "Array 4"="Array 4", "Status Output Locations"="Status Output Locations", "Board Index"="Board Index", "Connected Board ID's (Newfi)"="Connected Board ID's (Newfi)", "Agilent Channels"=w201, "Start DAQ Loop"="Start DAQ Loop", "Station IDs"=w199, "Network Var Set"=w193) -> (w207:T14)  [unwired: 1 in]
      }
      frame "Read Configuration File" {
        n76 = call "HCC Get Application Directory.vi"("Error In"=w212) -> ("Error Out"=w211:errorcluster, "General Configuration out"=w219:path, "Configuration Path out"=w228:path, "Station and Board IDs out"=w224:path)  [unwired: 5 in, 2 out]
        n77 = call "HCC Read Washer Config File.vi"("Station and Board IDs"=w224, "Configuration Path"=w228, "Error In"=w211) -> ("Status Output Locations"=w220:path[], "Station IDs"=w223:string[], "Voltage Indexes"=→"Voltage Indexes":i32[], "34972A_1"=w215:refnum<visa-resource-name>, "Board ID's"=w222:string[], "Disable Channel = True"=→"Disable Channel = True":bool[], "Agilent Channels DAQ"=w214:string, "Error Out"=w218:errorcluster)  [unwired: 8 in, 1 out]
        "Agilent Channels DAQ" <- w214
        "Connected Board IDs" <- w222
        "Find Newfi Error" <- w218
        n78 = call "HCC Get General Configuration Info.vi"("Error In"=w218, "General Configuration"=w219) -> ("Error Out"=w217:errorcluster, "Network Var Set"=w210:u8, "Disable Agilent Collection"=w216:bool)  [unwired: 7 in]
        "Network Var Set" <- w210
        n79 = local write "34972-1"(w215) -> ()
        n80 = local write "Disable Agilent Collection"(w216) -> ()
        n81 = local write "Status Output Locations"(w220) -> ()
        n82 = Bundle By Name(cluster=w226, "Status Output Locations"=w220, "Connected Board ID's (Newfi)"=w222, "Agilent Channels"=w214, "Station IDs"=w223, "Network Var Set"=w210) -> (w225:T14)
        n83 = case shown="2" w210 {
          frame 1, Default {
            n84 = shared-variable "My Computer\\Test Lib.lvlib\\Exit"(FALSE ("Exit")) -> ()  [unwired: 1 in, 1 out]
          }
          frame 2 {
            n85 = shared-variable "My Computer\\Test Lib.lvlib\\Exit-2"(FALSE ("Exit-2")) -> ()  [unwired: 1 in, 1 out]
          }
        }
        n86 = call <vilib>:"Add State(s) to Queue__jki_lib_state_machine.vi"("State(s) in (\"\")"=w227) -> ("States Out"=w229:string)  [unwired: 14 in]
      }
      frame "Show Station Labels" {
        n87 = Unbundle By Name(w253) -> ("Array"=w244:T1[], "Station IDs"=w246:string[], "Array 2"=w243:T1[], "Station IDs"=w241:string[], "Array 3"=w238:T1[], "Station IDs"=w236:string[], "Array 4"=w234:T1[], "Station IDs"=w233:string[])
        n88 = call "HCC Extract Rows.vi"("Station Group"=HCC_Station_Group."Station 1-6", "String"=w246) -> ("String Output"=w247:string[])  [unwired: 6 in, 3 out]
        n89 = call "HCC Extract Rows.vi"("Station Group"=HCC_Station_Group."Station 7-12", "String"=w241) -> ("String Output"=w242:string[])  [unwired: 6 in, 3 out]
        n90 = call "HCC Extract Rows.vi"("Station Group"=HCC_Station_Group."Station 13-18", "String"=w236) -> ("String Output"=w239:string[])  [unwired: 6 in, 3 out]
        n91 = call "HCC Extract Rows.vi"("Station Group"=HCC_Station_Group."Station 19-24", "String"=w233) -> ("String Output"=w235:string[])  [unwired: 6 in, 3 out]
        n92 = for {
          tunnel: w247 -> [w267] mode=indexing
          tunnel: w244 -> [w268] mode=indexing
          tunnel: [w266] -> w245 mode=indexing
          n93 = Bundle By Name(cluster=w268, "Display Data (RLT).Station Label Display"=w267) -> (w266:T1)
        }
        n94 = for {
          tunnel: w242 -> [w264] mode=indexing
          tunnel: w243 -> [w265] mode=indexing
          tunnel: [w263] -> w240 mode=indexing
          n95 = Bundle By Name(cluster=w265, "Display Data (RLT).Station Label Display"=w264) -> (w263:T1)
        }
        n96 = for {
          tunnel: w239 -> [w261] mode=indexing
          tunnel: w238 -> [w262] mode=indexing
          tunnel: [w260] -> w237 mode=indexing
          n97 = Bundle By Name(cluster=w262, "Display Data (RLT).Station Label Display"=w261) -> (w260:T1)
        }
        n98 = for {
          tunnel: w235 -> [w258] mode=indexing
          tunnel: w234 -> [w259] mode=indexing
          tunnel: [w257] -> w232 mode=indexing
          n99 = Bundle By Name(cluster=w259, "Display Data (RLT).Station Label Display"=w258) -> (w257:T1)
        }
        n100 = Bundle By Name(cluster=w253, "Array"=w245, "Array 2"=w240, "Array 3"=w237, "Array 4"=w232) -> (w252:T14)
        n101 = call <vilib>:"Add State(s) to Queue__jki_lib_state_machine.vi"("State(s) in (\"\")"=w255) -> ("States Out"=w256:string)  [unwired: 14 in]
      }
      frame "Data: Cleanup" {
        n102 = Unbundle By Name(w269) -> ("Core.Current VI Reference"=w272:refnum<vi>)
        n103 = Close Reference(reference=w272, error in (no error)=w271) -> (error out=w270:errorcluster)
        n104 = call <vilib>:"Add State(s) to Queue__jki_lib_state_machine.vi"("State(s) in (\"\")"=w274) -> ("States Out"=w273:string)  [unwired: 14 in]
      }
      frame "---------- UI ----------" {
        # "Do not put any code in this frame.\n(It is a separator no-op. You can make a copy of this frame to create a new UI frame)"
        n105 = call <vilib>:"Add State(s) to Queue__jki_lib_state_machine.vi"("State(s) in (\"\")"=w278) -> ("States Out"=w277:string)  [unwired: 14 in]
      }
      frame "UI: Initialize" {
        n106 = flat-sequence {
          tunnel: w283 -> [w289]
          tunnel: [w288] -> w281
          tunnel: w279 -> [w287]
          tunnel: [w293] -> w282
          tunnel: w281 -> [w293]
          tunnel: w279 -> [w291]
          tunnel: [w290] -> w280
          frame #0 {
            n107 = Unbundle By Name(w287) -> ("Network Var Set"=w286:u8)
            n108 = call "HCC Set Network Variables.vi"("Error In"=w289, "Network Var Set"=w286) -> ("Error Out"=w288:errorcluster)  [unwired: 9 in]
          }
          frame #1 {
            w292 = T1[] [{"Appliance Details"={"FileVersionInfo"={"FileVersion"="", "ProductName"="", "InternalName"="", "CompanyName"="", "LegalCopyright"="", "FileDescription"=""}, "Dishwasher Info"={"Open Cup Weight (gm):"=0.0, "Auto Cup Weight (gm):"=0.0, "Detergent-Dish:"="", "Inlet Temperature-Dish:"="", "Cycle Mode-Dish:"="", "Unit Control-Dish:"="", "Manufacturer-Dish:"=""}, "Washer Info"={"Hot Water Temperature (Fahrenheit):"="", "Cold Water Temperature (Fahrenheit):"="", "Capacity (cu.ft):"=0.0, "Initial Cloth Weight:"=0.0, "Cloth Lot:"=0, "Model Family:"="", "Program Name:"="", "Cycle Selection:"="", "Wash Temperature:"="", "Rinse Temperature:"="", "Load Size:"=""}, "File Name Output Array"=[], "Calibration Output Array"=[], "Appliance Common"={"Engineer:"="", "Model Number:"="", "Serial Number:"="", "Comments:"="", "Station ID:"="", "Technician:"="", "TR Number:"="", "Lab ID:"="", "Voltage:"="", "Water Pressure (PSI):"="", "Test Date:"="", "Computer Name:"="", "IP Address:"="", "Ambient RH:"="", "Frequency:"="", "Build:"="", "Filename:"="", "Test Type:"="", "Load Run #:"=0, "Ambient Temperature (F):"="", "File Path:"=path "", "Cycles Per Year"=60}, "Water Heater"={"Heating Mode:"=""}, "Dryer"={"Heat Setting:"="", "Washer Water Temperature (60 ± 5°F):"=60, "Water Hardness (PPM):"=17, "Dryness Setting:"="", "Dryer Type:"="", "Exhaust:"="", "Drying Cycle:"="", "Load Type:"="", "Nominal Load Weight"="", "Dryer Initial IMC Data"={"Measured IMC (lbs)"=7.0, "Actual Initial RMC (%)"=7.0, "RMC (Desired %)"=100.0, "Bone Dry Wt(lbs)"=7.0, "Tolerance(%)"=5.0, "Actual Final RMC (%)"=7.0, "CEF (lbf/kWh)"=0.0, "Minimum Weight (lbf)"=0.0, "Average Weight (lbf)"=0.0, "Maximum Weight (lbf)"=0.0, "Measured IMC In Range?"=FALSE, "Moisture Reduction Factor"=55.5, "Field Use Factor"=1.04, "Empty Dryer Cold Weigth"=0.0, "Energy Standard"=enum."D2-Automatic Dryer", "Weight Cloth (lbs)"=0.0, "Relative Moisture Content (%)"=0.0, "Relative Moisture Content - Avg (%)"=0.0}}}, "Display Data (RLT)"={"Status Color"=0, "Serial Number Display"="", "Cycle Count Display"=0, "Station Label Display"="", "Current Run Start Time Display"=0.0, "Board ID Display"="", "RPM Display"=0, "Current Display"=0.0, "Current Path Display"=path "", "Saving Display"=FALSE, "Unit Type Display"=enum."", "Total Time On Display"=0.0, "UI Button"=FALSE}}, {"Appliance Details"={"FileVersionInfo"={"FileVersion"="", "ProductName"="", "InternalName"="", "CompanyName"="", "LegalCopyright"="", "FileDescription"=""}, "Dishwasher Info"={"Open Cup Weight (gm):"=0.0, "Auto Cup Weight (gm):"=0.0, "Detergent-Dish:"="", "Inlet Temperature-Dish:"="", "Cycle Mode-Dish:"="", "Unit Control-Dish:"="", "Manufacturer-Dish:"=""}, "Washer Info"={"Hot Water Temperature (Fahrenheit):"="", "Cold Water Temperature (Fahrenheit):"="", "Capacity (cu.ft):"=0.0, "Initial Cloth Weight:"=0.0, "Cloth Lot:"=0, "Model Family:"="", "Program Name:"="", "Cycle Selection:"="", "Wash Temperature:"="", "Rinse Temperature:"="", "Load Size:"=""}, "File Name Output Array"=[], "Calibration Output Array"=[], "Appliance Common"={"Engineer:"="", "Model Number:"="", "Serial Number:"="", "Comments:"="", "Station ID:"="", "Technician:"="", "TR Number:"="", "Lab ID:"="", "Voltage:"="", "Water Pressure (PSI):"="", "Test Date:"="", "Computer Name:"="", "IP Address:"="", "Ambient RH:"="", "Frequency:"="", "Build:"="", "Filename:"="", "Test Type:"="", "Load Run #:"=0, "Ambient Temperature (F):"="", "File Path:"=path "", "Cycles Per Year"=60}, "Water Heater"={"Heating Mode:"=""}, "Dryer"={"Heat Setting:"="", "Washer Water Temperature (60 ± 5°F):"=60, "Water Hardness (PPM):"=17, "Dryness Setting:"="", "Dryer Type:"="", "Exhaust:"="", "Drying Cycle:"="", "Load Type:"="", "Nominal Load Weight"="", "Dryer Initial IMC Data"={"Measured IMC (lbs)"=7.0, "Actual Initial RMC (%)"=7.0, "RMC (Desired %)"=100.0, "Bone Dry Wt(lbs)"=7.0, "Tolerance(%)"=5.0, "Actual Final RMC (%)"=7.0, "CEF (lbf/kWh)"=0.0, "Minimum Weight (lbf)"=0.0, "Average Weight (lbf)"=0.0, "Maximum Weight (lbf)"=0.0, "Measured IMC In Range?"=FALSE, "Moisture Reduction Factor"=55.5, "Field Use Factor"=1.04, "Empty Dryer Cold Weigth"=0.0, "Energy Standard"=enum."D2-Automatic Dryer", "Weight Cloth (lbs)"=0.0, "Relative Moisture Content (%)"=0.0, "Relative Moisture Content - Avg (%)"=0.0}}}, "Display Data (RLT)"={"Status Color"=0, "Serial Number Display"="", "Cycle Count Display"=0, "Station Label Display"="", "Current Run Start Time Display"=0.0, "Board ID Display"="", "RPM Display"=0, "Current Display"=0.0, "Current Path Display"=path "", "Saving Display"=FALSE, "Unit Type Display"=enum."", "Total Time On Display"=0.0, "UI Button"=FALSE}}, {"Appliance Details"={"FileVersionInfo"={"FileVersion"="", "ProductName"="", "InternalName"="", "CompanyName"="", "LegalCopyright"="", "FileDescription"=""}, "Dishwasher Info"={"Open Cup Weight (gm):"=0.0, "Auto Cup Weight (gm):"=0.0, "Detergent-Dish:"="", "Inlet Temperature-Dish:"="", "Cycle Mode-Dish:"="", "Unit Control-Dish:"="", "Manufacturer-Dish:"=""}, "Washer Info"={"Hot Water Temperature (Fahrenheit):"="", "Cold Water Temperature (Fahrenheit):"="", "Capacity (cu.ft):"=0.0, "Initial Cloth Weight:"=0.0, "Cloth Lot:"=0, "Model Family:"="", "Program Name:"="", "Cycle Selection:"="", "Wash Temperature:"="", "Rinse Temperature:"="", "Load Size:"=""}, "File Name Output Array"=[], "Calibration Output Array"=[], "Appliance Common"={"Engineer:"="", "Model Number:"="", "Serial Number:"="", "Comments:"="", "Station ID:"="", "Technician:"="", "TR Number:"="", "Lab ID:"="", "Voltage:"="", "Water Pressure (PSI):"="", "Test Date:"="", "Computer Name:"="", "IP Address:"="", "Ambient RH:"="", "Frequency:"="", "Build:"="", "Filename:"="", "Test Type:"="", "Load Run #:"=0, "Ambient Temperature (F):"="", "File Path:"=path "", "Cycles Per Year"=60}, "Water Heater"={"Heating Mode:"=""}, "Dryer"={"Heat Setting:"="", "Washer Water Temperature (60 ± 5°F):"=60, "Water Hardness (PPM):"=17, "Dryness Setting:"="", "Dryer Type:"="", "Exhaust:"="", "Drying Cycle:"="", "Load Type:"="", "Nominal Load Weight"="", "Dryer Initial IMC Data"={"Measured IMC (lbs)"=7.0, "Actual Initial RMC (%)"=7.0, "RMC (Desired %)"=100.0, "Bone Dry Wt(lbs)"=7.0, "Tolerance(%)"=5.0, "Actual Final RMC (%)"=7.0, "CEF (lbf/kWh)"=0.0, "Minimum Weight (lbf)"=0.0, "Average Weight (lbf)"=0.0, "Maximum Weight (lbf)"=0.0, "Measured IMC In Range?"=FALSE, "Moisture Reduction Factor"=55.5, "Field Use Factor"=1.04, "Empty Dryer Cold Weigth"=0.0, "Energy Standard"=enum."D2-Automatic Dryer", "Weight Cloth (lbs)"=0.0, "Relative Moisture Content (%)"=0.0, "Relative Moisture Content - Avg (%)"=0.0}}}, "Display Data (RLT)"={"Status Color"=0, "Serial Number Display"="", "Cycle Count Display"=0, "Station Label Display"="", "Current Run Start Time Display"=0.0, "Board ID Display"="", "RPM Display"=0, "Current Display"=0.0, "Current Path Display"=path "", "Saving Display"=FALSE, "Unit Type Display"=enum."", "Total Time On Display"=0.0, "UI Button"=FALSE}}, {"Appliance Details"={"FileVersionInfo"={"FileVersion"="", "ProductName"="", "InternalName"="", "CompanyName"="", "LegalCopyright"="", "FileDescription"=""}, "Dishwasher Info"={"Open Cup Weight (gm):"=0.0, "Auto Cup Weight (gm):"=0.0, "Detergent-Dish:"="", "Inlet Temperature-Dish:"="", "Cycle Mode-Dish:"="", "Unit Control-Dish:"="", "Manufacturer-Dish:"=""}, "Washer Info"={"Hot Water Temperature (Fahrenheit):"="", "Cold Water Temperature (Fahrenheit):"="", "Capacity (cu.ft):"=0.0, "Initial Cloth Weight:"=0.0, "Cloth Lot:"=0, "Model Family:"="", "Program Name:"="", "Cycle Selection:"="", "Wash Temperature:"="", "Rinse Temperature:"="", "Load Size:"=""}, "File Name Output Array"=[], "Calibration Output Array"=[], "Appliance Common"={"Engineer:"="", "Model Number:"="", "Serial Number:"="", "Comments:"="", "Station ID:"="", "Technician:"="", "TR Number:"="", "Lab ID:"="", "Voltage:"="", "Water Pressure (PSI):"="", "Test Date:"="", "Computer Name:"="", "IP Address:"="", "Ambient RH:"="", "Frequency:"="", "Build:"="", "Filename:"="", "Test Type:"="", "Load Run #:"=0, "Ambient Temperature (F):"="", "File Path:"=path "", "Cycles Per Year"=60}, "Water Heater"={"Heating Mode:"=""}, "Dryer"={"Heat Setting:"="", "Washer Water Temperature (60 ± 5°F):"=60, "Water Hardness (PPM):"=17, "Dryness Setting:"="", "Dryer Type:"="", "Exhaust:"="", "Drying Cycle:"="", "Load Type:"="", "Nominal Load Weight"="", "Dryer Initial IMC Data"={"Measured IMC (lbs)"=7.0, "Actual Initial RMC (%)"=7.0, "RMC (Desired %)"=100.0, "Bone Dry Wt(lbs)"=7.0, "Tolerance(%)"=5.0, "Actual Final RMC (%)"=7.0, "CEF (lbf/kWh)"=0.0, "Minimum Weight (lbf)"=0.0, "Average Weight (lbf)"=0.0, "Maximum Weight (lbf)"=0.0, "Measured IMC In Range?"=FALSE, "Moisture Reduction Factor"=55.5, "Field Use Factor"=1.04, "Empty Dryer Cold Weigth"=0.0, "Energy Standard"=enum."D2-Automatic Dryer", "Weight Cloth (lbs)"=0.0, "Relative Moisture Content (%)"=0.0, "Relative Moisture Content - Avg (%)"=0.0}}}, "Display Data (RLT)"={"Status Color"=0, "Serial Number Display"="", "Cycle Count Display"=0, "Station Label Display"="", "Current Run Start Time Display"=0.0, "Board ID Display"="", "RPM Display"=0, "Current Display"=0.0, "Current Path Display"=path "", "Saving Display"=FALSE, "Unit Type Display"=enum."", "Total Time On Display"=0.0, "UI Button"=FALSE}}, {"Appliance Details"={"FileVersionInfo"={"FileVersion"="", "ProductName"="", "InternalName"="", "CompanyName"="", "LegalCopyright"="", "FileDescription"=""}, "Dishwasher Info"={"Open Cup Weight (gm):"=0.0, "Auto Cup Weight (gm):"=0.0, "Detergent-Dish:"="", "Inlet Temperature-Dish:"="", "Cycle Mode-Dish:"="", "Unit Control-Dish:"="", "Manufacturer-Dish:"=""}, "Washer Info"={"Hot Water Temperature (Fahrenheit):"="", "Cold Water Temperature (Fahrenheit):"="", "Capacity (cu.ft):"=0.0, "Initial Cloth Weight:"=0.0, "Cloth Lot:"=0, "Model Family:"="", "Program Name:"="", "Cycle Selection:"="", "Wash Temperature:"="", "Rinse Temperature:"="", "Load Size:"=""}, "File Name Output Array"=[], "Calibration Output Array"=[], "Appliance Common"={"Engineer:"="", "Model Number:"="", "Serial Number:"="", "Comments:"="", "Station ID:"="", "Technician:"="", "TR Number:"="", "Lab ID:"="", "Voltage:"="", "Water Pressure (PSI):"="", "Test Date:"="", "Computer Name:"="", "IP Address:"="", "Ambient RH:"="", "Frequency:"="", "Build:"="", "Filename:"="", "Test Type:"="", "Load Run #:"=0, "Ambient Temperature (F):"="", "File Path:"=path "", "Cycles Per Year"=60}, "Water Heater"={"Heating Mode:"=""}, "Dryer"={"Heat Setting:"="", "Washer Water Temperature (60 ± 5°F):"=60, "Water Hardness (PPM):"=17, "Dryness Setting:"="", "Dryer Type:"="", "Exhaust:"="", "Drying Cycle:"="", "Load Type:"="", "Nominal Load Weight"="", "Dryer Initial IMC Data"={"Measured IMC (lbs)"=7.0, "Actual Initial RMC (%)"=7.0, "RMC (Desired %)"=100.0, "Bone Dry Wt(lbs)"=7.0, "Tolerance(%)"=5.0, "Actual Final RMC (%)"=7.0, "CEF (lbf/kWh)"=0.0, "Minimum Weight (lbf)"=0.0, "Average Weight (lbf)"=0.0, "Maximum Weight (lbf)"=0.0, "Measured IMC In Range?"=FALSE, "Moisture Reduction Factor"=55.5, "Field Use Factor"=1.04, "Empty Dryer Cold Weigth"=0.0, "Energy Standard"=enum."D2-Automatic Dryer", "Weight Cloth (lbs)"=0.0, "Relative Moisture Content (%)"=0.0, "Relative Moisture Content - Avg (%)"=0.0}}}, "Display Data (RLT)"={"Status Color"=0, "Serial Number Display"="", "Cycle Count Display"=0, "Station Label Display"="", "Current Run Start Time Display"=0.0, "Board ID Display"="", "RPM Display"=0, "Current Display"=0.0, "Current Path Display"=path "", "Saving Display"=FALSE, "Unit Type Display"=enum."", "Total Time On Display"=0.0, "UI Button"=FALSE}}, {"Appliance Details"={"FileVersionInfo"={"FileVersion"="", "ProductName"="", "InternalName"="", "CompanyName"="", "LegalCopyright"="", "FileDescription"=""}, "Dishwasher Info"={"Open Cup Weight (gm):"=0.0, "Auto Cup Weight (gm):"=0.0, "Detergent-Dish:"="", "Inlet Temperature-Dish:"="", "Cycle Mode-Dish:"="", "Unit Control-Dish:"="", "Manufacturer-Dish:"=""}, "Washer Info"={"Hot Water Temperature (Fahrenheit):"="", "Cold Water Temperature (Fahrenheit):"="", "Capacity (cu.ft):"=0.0, "Initial Cloth Weight:"=0.0, "Cloth Lot:"=0, "Model Family:"="", "Program Name:"="", "Cycle Selection:"="", "Wash Temperature:"="", "Rinse Temperature:"="", "Load Size:"=""}, "File Name Output Array"=[], "Calibration Output Array"=[], "Appliance Common"={"Engineer:"="", "Model Number:"="", "Serial Number:"="", "Comments:"="", "Station ID:"="", "Technician:"="", "TR Number:"="", "Lab ID:"="", "Voltage:"="", "Water Pressure (PSI):"="", "Test Date:"="", "Computer Name:"="", "IP Address:"="", "Ambient RH:"="", "Frequency:"="", "Build:"="", "Filename:"="", "Test Type:"="", "Load Run #:"=0, "Ambient Temperature (F):"="", "File Path:"=path "", "Cycles Per Year"=60}, "Water Heater"={"Heating Mode:"=""}, "Dryer"={"Heat Setting:"="", "Washer Water Temperature (60 ± 5°F):"=60, "Water Hardness (PPM):"=17, "Dryness Setting:"="", "Dryer Type:"="", "Exhaust:"="", "Drying Cycle:"="", "Load Type:"="", "Nominal Load Weight"="", "Dryer Initial IMC Data"={"Measured IMC (lbs)"=7.0, "Actual Initial RMC (%)"=7.0, "RMC (Desired %)"=100.0, "Bone Dry Wt(lbs)"=7.0, "Tolerance(%)"=5.0, "Actual Final RMC (%)"=7.0, "CEF (lbf/kWh)"=0.0, "Minimum Weight (lbf)"=0.0, "Average Weight (lbf)"=0.0, "Maximum Weight (lbf)"=0.0, "Measured IMC In Range?"=FALSE, "Moisture Reduction Factor"=55.5, "Field Use Factor"=1.04, "Empty Dryer Cold Weigth"=0.0, "Energy Standard"=enum."D2-Automatic Dryer", "Weight Cloth (lbs)"=0.0, "Relative Moisture Content (%)"=0.0, "Relative Moisture Content - Avg (%)"=0.0}}}, "Display Data (RLT)"={"Status Color"=0, "Serial Number Display"="", "Cycle Count Display"=0, "Station Label Display"="", "Current Run Start Time Display"=0.0, "Board ID Display"="", "RPM Display"=0, "Current Display"=0.0, "Current Path Display"=path "", "Saving Display"=FALSE, "Unit Type Display"=enum."", "Total Time On Display"=0.0, "UI Button"=FALSE}}] ("Array")
            n109 = local write "Array"(w292) -> ()
            n110 = local write "Array 2"(w292) -> ()
            n111 = local write "Array 3"(w292) -> ()
            n112 = local write "Array 4"(w292) -> ()
            n113 = Bundle By Name(cluster=w291, "Array"=w292, "Array 2"=w292, "Array 3"=w292, "Array 4"=w292) -> (w290:T14)
          }
        }
        n114 = call <vilib>:"Add State(s) to Queue__jki_lib_state_machine.vi"("State(s) in (\"\")"=w285) -> ("States Out"=w284:string)  [unwired: 14 in]
      }
      frame "UI: Cursor Set" {
        # "Argument"
        n115 = case shown="\"Busy\"" w294 {
          tunnel: w296 -> [w301 w303]
          tunnel: [w300 w302] -> w295
          frame "Idle", Default {
            n116 = call <vilib>:"Unset Busy.vi"("error in (no error)"=w301) -> ("error out"=w300:errorcluster)  [unwired: 10 in]
          }
          frame "Busy" {
            n117 = call <vilib>:"Set Busy.vi"("error in (no error)"=w303) -> ("error out"=w302:errorcluster)  [unwired: 9 in, 1 out]
          }
        }
        n118 = call <vilib>:"Add State(s) to Queue__jki_lib_state_machine.vi"("State(s) in (\"\")"=w299) -> ("States Out"=w298:string)  [unwired: 14 in]
      }
      frame "UI: Front Panel State" {
        # "Argument"
        n119 = Unbundle By Name(w307) -> ("Core.Current VI Reference"=w306:refnum<vi>)
        n120 = case shown="\"Open\", Default" w305 {
          tunnel: w309 -> [w315 w328]
          tunnel: [w317 w329] -> w308
          tunnel: w306 -> [w316 w326]
          frame "Open", Default {
            n121 = property class="VI"(reference=w316, error in=w315) -> (reference out=w313:refnum<vi>, error out=w314:errorcluster, "Front Panel.Open"=w312:bool)
            n122 = case shown="True" w312 {
              tunnel: [w318 w321] -> w317
              tunnel: w314 -> [w318 w320]
              tunnel: w313 -> [_ w319]
              frame False {
              }
              frame True {
                n123 = invoke class="VI" method="FP.Open"(reference=w319, error in=w320, "Activate"=TRUE, "State"=T13."Maximized") -> (error out=w321:errorcluster)  [unwired: 1 in, 4 out]
              }
            }
          }
          frame "Close" {
            n124 = property class="VI"(reference=w326, error in=w328) -> (reference out=w325:refnum<vi>, error out=w327:errorcluster, "Front Panel.Open"=w324:bool)
            n125 = case shown="True" w324 {
              tunnel: [w330 w333] -> w329
              tunnel: w327 -> [w330 w332]
              tunnel: w325 -> [_ w331]
              frame False {
              }
              frame True {
                n126 = invoke class="VI" method="FP.Close"(reference=w331, error in=w332) -> (error out=w333:errorcluster)  [unwired: 1 in, 2 out]
              }
            }
          }
        }
        n127 = local write "Start DAQ Loop"(TRUE ("Start DAQ Loop")) -> ()
        n128 = call <vilib>:"Add State(s) to Queue__jki_lib_state_machine.vi"("State(s) in (\"\")"=w311) -> ("States Out"=w310:string)  [unwired: 14 in]
      }
      frame "---------- Macro ----------" {
        # "Do not put any code in this frame.\n(It is a separator no-op. You can make a copy of this frame to create a new Macro frame)"
        n129 = call <vilib>:"Add State(s) to Queue__jki_lib_state_machine.vi"("State(s) in (\"\")"=w337) -> ("States Out"=w336:string)  [unwired: 14 in]
      }
      frame "Macro: Initialize" {
        w338 = "Data: Initialize\nRead Configuration File\nInitialize Core Data\nUI: Initialize\nShow Station Labels\nUI: Front Panel State >> Open"  # Data: Initialize Read Configuration File Initialize Core Data UI: Initialize Show Station Labels UI: Front Panel State >> Open
        n130 = call <vilib>:"Add State(s) to Queue__jki_lib_state_machine.vi"("State(s) in Front (\"\")"=w338, "State(s) in (\"\")"=w342) -> ("States Out"=w341:string)  [unwired: 13 in]
      }
      frame "Macro: Exit" {
        n131 = Unbundle By Name(w349) -> ("Core.Close Panel on Exit?"=w348:bool)
        n132 = Select(t="UI: Front Panel State >> Close", s=w348, f="") -> (s? t:f=w345:string)
        n133 = call <vilib>:"Add State(s) to Queue__jki_lib_state_machine.vi"("State(s) in (\"\")"=w345, "State(s) at Back (\"\")"="Data: Cleanup\nExit") -> ("States Out"=w343:string)  [unwired: 13 in]
        n134 = call <vilib>:"Add State(s) to Queue__jki_lib_state_machine.vi"("State(s) in Front (\"\")"=w343, "State(s) in (\"\")"=w352) -> ("States Out"=w351:string)  [unwired: 13 in]
      }
      frame "---------- New Category ----------" {
        # "Template Separator\n(You can make a copy of, or modify, this frame)"
        n135 = call <vilib>:"Add State(s) to Queue__jki_lib_state_machine.vi"("State(s) in (\"\")"=w356) -> ("States Out"=w355:string)  [unwired: 14 in]
      }
      frame "Update Status 1" {
        # "Updated to extract both GEA2 and ERD network\nvariables"
        n136 = Unbundle By Name(w371) -> ("Network Var Set"=w357:u8, "Array"=w364:T1[], "Station IDs"=w359:string[])
        n137 = local read "Current"() -> (w367:dbl[])
        n138 = local read "Save Array"() -> (w366:bool[])
        n139 = call "HCC Extract Rows.vi"("Station Group"=HCC_Station_Group."Station 1-6", "error in (no error)"=w360, "String"=w359, "Saving"=w366, "Board Index"=w367) -> ("error out"=w362:errorcluster, "String Output"=w358:string[], "Board Index"=w368:dbl[])  [unwired: 3 in, 1 out]
        n140 = call "HCC Extract Newtwork Variable.vi"("Network Var Set"=w357, "Station IDs"=w358, "Current"=w368, "Network Variable Location"=i32[] [0, 1, 2, 3, 4, 5] ("Board Index"), "Input"=w364) -> ("Output"=w363:T1[])  [unwired: 5 in, 1 out]
        n141 = local write "Array"(w363) -> ()
        n142 = Bundle By Name(cluster=w371, "Array"=w363) -> (w370:T14)
        n143 = call <vilib>:"Add State(s) to Queue__jki_lib_state_machine.vi"("State(s) in (\"\")"=w369) -> ("States Out"=w372:string)  [unwired: 14 in]
      }
      frame "Update Status 2" {
        # "Updated to extract both GEA2 and ERD network\nvariables"
        n144 = Unbundle By Name(w387) -> ("Network Var Set"=w373:u8, "Array 2"=w380:T1[], "Station IDs"=w375:string[])
        n145 = local read "Current"() -> (w383:dbl[])
        n146 = local read "Save Array"() -> (w382:bool[])
        n147 = call "HCC Extract Rows.vi"("Station Group"=HCC_Station_Group."Station 7-12", "error in (no error)"=w376, "String"=w375, "Saving"=w382, "Board Index"=w383) -> ("error out"=w378:errorcluster, "String Output"=w374:string[], "Board Index"=w384:dbl[])  [unwired: 3 in, 1 out]
        n148 = call "HCC Extract Newtwork Variable.vi"("Network Var Set"=w373, "Station IDs"=w374, "Current"=w384, "Network Variable Location"=i32[] [6, 7, 8, 9, 10, 11] ("Board Index"), "Input"=w380) -> ("Output"=w379:T1[])  [unwired: 5 in, 1 out]
        n149 = local write "Array 2"(w379) -> ()
        n150 = Bundle By Name(cluster=w387, "Array 2"=w379) -> (w386:T14)
        n151 = call <vilib>:"Add State(s) to Queue__jki_lib_state_machine.vi"("State(s) in (\"\")"=w385) -> ("States Out"=w388:string)  [unwired: 14 in]
      }
      frame "Update Status 3" {
        # "Updated to extract both GEA2 and ERD network\nvariables"
        n152 = Unbundle By Name(w403) -> ("Network Var Set"=w389:u8, "Array 3"=w396:T1[], "Station IDs"=w391:string[])
        n153 = local read "Current"() -> (w399:dbl[])
        n154 = local read "Save Array"() -> (w398:bool[])
        n155 = call "HCC Extract Rows.vi"("Station Group"=HCC_Station_Group."Station 13-18", "error in (no error)"=w392, "String"=w391, "Saving"=w398, "Board Index"=w399) -> ("error out"=w394:errorcluster, "String Output"=w390:string[], "Board Index"=w400:dbl[])  [unwired: 3 in, 1 out]
        n156 = call "HCC Extract Newtwork Variable.vi"("Network Var Set"=w389, "Station IDs"=w390, "Current"=w400, "Network Variable Location"=i32[] [12, 13, 14, 15, 16, 17] ("Board Index"), "Input"=w396) -> ("Output"=w395:T1[])  [unwired: 5 in, 1 out]
        n157 = local write "Array 3"(w395) -> ()
        n158 = Bundle By Name(cluster=w403, "Array 3"=w395) -> (w402:T14)
        n159 = call <vilib>:"Add State(s) to Queue__jki_lib_state_machine.vi"("State(s) in (\"\")"=w401) -> ("States Out"=w404:string)  [unwired: 14 in]
      }
      frame "Update Status 4" {
        # "Updated to extract both GEA2 and ERD network\nvariables"
        n160 = Unbundle By Name(w419) -> ("Network Var Set"=w405:u8, "Array 4"=w412:T1[], "Station IDs"=w407:string[])
        n161 = local read "Current"() -> (w415:dbl[])
        n162 = local read "Save Array"() -> (w413:bool[])
        n163 = call "HCC Extract Rows.vi"("Station Group"=HCC_Station_Group."Station 19-24", "error in (no error)"=w408, "String"=w407, "Saving"=w413, "Board Index"=w415) -> ("error out"=w410:errorcluster, "String Output"=w406:string[], "Board Index"=w417:dbl[])  [unwired: 3 in, 1 out]
        n164 = call "HCC Extract Newtwork Variable.vi"("Network Var Set"=w405, "Station IDs"=w406, "Current"=w417, "Network Variable Location"=i32[] [18, 19, 20, 21, 22, 23] ("Board Index"), "Input"=w412) -> ("Output"=w414:T1[])  [unwired: 5 in, 1 out]
        n165 = local write "Array 4"(w414) -> ()
        n166 = Bundle By Name(cluster=w419, "Array 4"=w414) -> (w418:T14)
        n167 = call <vilib>:"Add State(s) to Queue__jki_lib_state_machine.vi"("State(s) in (\"\")"=w416) -> ("States Out"=w420:string)  [unwired: 14 in]
      }
      frame "Open Newfi Panel" {
        n168 = Unbundle By Name(w425) -> ("Open Panel.Display Data (RLT).Board ID Display"=w423:string, "Network Var Set"=w421:u8)
        n169 = case shown="2" w421 {
          tunnel: w423 -> [w427 w428]
          frame 1, Default {
            n170 = shared-variable ".\\Test Lib.lvlib\\Board ID"(w427) -> ()  [unwired: 1 in, 1 out]
          }
          frame 2 {
            n171 = shared-variable "My Computer\\Test Lib.lvlib\\Board ID-2"(w428) -> ()  [unwired: 1 in, 1 out]
          }
        }
        n172 = call <vilib>:"Add State(s) to Queue__jki_lib_state_machine.vi"("State(s) in (\"\")"=w422) -> ("States Out"=w426:string)  [unwired: 14 in]
      }
    }
    n173 = case shown="True" "Debug" {
      tunnel: w12 -> [_ w27]
      tunnel: w13 -> [w25 w28]
      tunnel: [w25 w26] -> w11
      frame False {
      }
      frame True {
        n174 = Build Array (concatenate)(w28, w27) -> (w26:string[])
        "Main Loop" <- w26
      }
    }
  }
  n175 = while "Agilent DAQ and Save" {
    shift-right: [w439] -> _
    shift-left: _ -> [w438]
    shift-right: [w441] -> _
    shift-left: w4 -> [w442]
    tunnel: "error in (no error)" -> [w436]
    tunnel: [w437] -> w7
    shift-right: [w433] -> _
    shift-left: string[] [] -> [w435]
    stop <- w440 stop-if-true
    # "Agilent DAQ and Save"
    n176 = local read "Agilent Scan Rate (Seconds)"() -> (w431:i32)
    n177 = local read "Debug"() -> (w432:bool)
    n178 = call <vilib>:"Parse State Queue__JKI_lib_State_Machine.vi"("State Queue"=w442, "Error In (no error)"=w436) -> ("Remaining States"=w443:string, "Current State"=w434:string)  [unwired: 11 in, 1 out]
    n179 = Multiply(x=w431, y=1000) -> (x*y=w429:i32)
    n180 = case shown="\"Agilent DAQ\"" w434 {
      selector: w434 -> [_ _ _ _ _ w510 _ _ _ _ _]
      tunnel: w443 -> [w454 w476 w481 w490 w507 w518 w522 w538 w548 w809 w814]
      tunnel: w438 -> [w452 w474 w479 _ w505 w516 w520 w536 w543 w807 w812]
      tunnel: [w453 w475 w480 w489 w506 w517 w521 w537 w547 w808 w813] -> w441
      tunnel: [_ _ _ _ _ _ _ _ _ TRUE TRUE] -> w440
      tunnel: [w451 w474 w479 w488 w504 w516 w520 w535 w543 w807 w812] -> w439
      tunnel: w429 -> [w450 _ _ _ _ _ _ _ _ _ _]
      tunnel: w436 -> [w449 w473 w477 w486 w502 w509 w519 w531 w546 w805 w810]
      tunnel: [w448 w473 w477 w486 w496 w508 w519 w530 w546 w805 w810] -> w437
      frame "", "Idle" {
        n181 = event shown="[0] Timeout" {
          selector: _ -> [_ _]
          dyn-events: _ -> [_ _]
          timeout: w450 -> [_ _]
          tunnel: w454 -> [w461 w472]
          tunnel: [w460 w471] -> w453
          tunnel: w452 -> [w459 w469]
          tunnel: [w459 w469] -> w451
          tunnel: [w456 w466] -> w448
          tunnel: w449 -> [w456 w467]
          event Timeout {
            n182 = event-data() -> ()  [unwired: 1 in, 1 out]
            n183 = local write "Collecting Agilent Data"(FALSE ("Collecting Agilent Data")) -> ()
            n184 = case shown="True" "Disable Agilent Collection" {
              tunnel: ["Agilent DAQ\nSave Agilent Data" ""] -> w458
              frame False {
              }
              frame True {
                n185 = local write "Current"(dbl[] [0.0, 0.0, 0.0, 0.0, 0.0, 0.0, 0.0, 0.0, 0.0, 0.0, 0.0, 0.0, 0.0, 0.0, 0.0, 0.0, 0.0, 0.0, 0.0, 0.0, 0.0, 0.0, 0.0, 0.0] ("Current")) -> ()
                n186 = local write "Save Array"(bool[] [FALSE, FALSE, FALSE, FALSE, FALSE, FALSE, FALSE, FALSE, FALSE, FALSE, FALSE, FALSE, FALSE, FALSE, FALSE, FALSE, FALSE, FALSE, FALSE, FALSE, FALSE, FALSE, FALSE, FALSE] ("Save Array")) -> ()
              }
            }
            n187 = call <vilib>:"Add State(s) to Queue__jki_lib_state_machine.vi"("State(s) in Front (\"\")"=w458, "State(s) in (\"\")"=w461) -> ("States Out"=w460:string)  [unwired: 13 in]
          }
          event "Quit": Value Change {
            n188 = event-data() -> ()  [unwired: 1 in, 6 out]
            n189 = Unbundle By Name(w469) -> ("34972-1"=w468:refnum<visa-resource-name>)
            n190 = call "Close.vi"("VISA Resource Name"=w468, "error in (no error)"=w467) -> ("error out"=w466:errorcluster)  [unwired: 13 in]
            n191 = call <vilib>:"Add State(s) to Queue__jki_lib_state_machine.vi"("State(s) in Front (\"\")"="Exit", "State(s) in (\"\")"=w472) -> ("States Out"=w471:string)  [unwired: 13 in]
          }
        }
      }
      frame "------Initialize------" {
        # "Initialization Macro\n(This is called once, when the VI starts)"
        n192 = call <vilib>:"Add State(s) to Queue__jki_lib_state_machine.vi"("State(s) in (\"\")"=w476) -> ("States Out"=w475:string)  [unwired: 14 in]
      }
      frame "Macro: Initialize" {
        # "Initialization Macro\n(This is called once, when the VI starts)"
        n193 = call <vilib>:"Add State(s) to Queue__jki_lib_state_machine.vi"("State(s) in Front (\"\")"="Data: Initialize\nInit Agilent", "State(s) in (\"\")"=w481) -> ("States Out"=w480:string)  [unwired: 13 in]
      }
      frame "Data: Initialize" {
        w482 = dbl[] []  # Voltage
        w487 = dbl[] []  # Current
        n194 = while {
          tunnel: ["34972-1"] -> w483
          tunnel: ["Agilent Scan Rate (Seconds)"] -> w485
          tunnel: [w491] -> w484
          stop <- w494 stop-if-true
          # "Wait for Main loop initialization"
          n195 = Wait Until Next ms Multiple(millisecond multiple=u32 100) -> ()  [unwired: 1 out]
          n196 = local read "Agilent Channels DAQ"() -> (w491:string)
          n197 = local read "Start DAQ Loop"() -> (w494:bool)
        }
        n198 = Bundle("34972-1"=w483, "Agilent Scan Rate (Seconds)"=w485, "Current"=w487, "Voltage"=w482, "Agilent Channels DAQ"=w484) -> (w488:T15)  [unwired: 1 in]
        n199 = call <vilib>:"Add State(s) to Queue__jki_lib_state_machine.vi"("State(s) in (\"\")"=w490) -> ("States Out"=w489:string)  [unwired: 14 in]
      }
      frame "Init Agilent" {
        n200 = Unbundle By Name(w505) -> ("34972-1"=w503:refnum<visa-resource-name>, "Agilent Channels DAQ"=w500:string)
        n201 = call "Error Query (Multiple).vi"("VISA Resource Name"=w503, "error in (no error)"=w502) -> ("VISA Resource Name Out"=w498:refnum<visa-resource-name>, "error out"=w501:errorcluster)  [unwired: 10 in, 2 out]
        n202 = call "DOE Agilent Setup SUB.vi"("Analog Channels-List"=w500, "error in (no error)"=w501, "Agilent Gain"=1.0, "VISA Refnum in"=w498) -> ("error out"=w496:errorcluster, "Clean Analog Scan List"=w499:string)  [unwired: 5 in, 1 out]
        n203 = Bundle By Name(cluster=w505, "34972-1"=w498, "Agilent Channels DAQ"=w499) -> (w504:T15)
        n204 = call <vilib>:"Add State(s) to Queue__jki_lib_state_machine.vi"("State(s) in (\"\")"=w507) -> ("States Out"=w506:string)  [unwired: 14 in]
      }
      frame Default {
        w512 = 42 items=["No error", "Argument error", "Memory is full", "Out of zone", "End of file", "File already open", "Generic file I/O error", "File not found", "File permission error", "Disk is full", "Duplicate path", "Too many files open", "System feature not enabled", "Resource file not found", "Cannot add resource", "Resource not found", "Image not found", "Image memory error", "Pen does not exist", "Config type invalid", "Config token not found", "Config parse error", "Config memory error", "Bad external code format", "Bad external code offset", "External code not present", "Null window", "Destroy window error", "Null menu", "Print aborted", "Bad print record", "Print driver error", "Windows error during printing", "Memory error during printing", "Print dialog error", "Generic print error", "Invalid device refnum", "Device not found", "Device parameter error", "Device unit error", "Cannot open device", "Device call aborted", "Generic error", "Cancelled by user", "Object ID too low", "Object ID too high", "Object not in heap", "Unknown heap", "Unknown object (invalid DefProc)", "Unknown object (DefProc not in table)", "Message out of range", "Invalid (null) method", "Unknown message", "Manager call not supported", "Bad address", "Network operation in progress", "Network operation timed out", "Connection is busy", "Network attribute not supported", "Network error", "Address in use", "System out of memory", "Connection aborted", "Connection refused", "Not connected", "Already connected", "Connection closed", "Initialization error (interapplication manager)", "Bad occurrence", "Wait on unbound occurrence handler", "Occurrence queue overflow", "Datalog type conflict", "Unused", "Unrecognized type (interapplication manager)", "Memory corrupt", "Failed to make temporary DLL", "Old CIN version", "Drag socket not found", "Failed to load drop-object", "Failed to register OLE object", "Failed to release OLE object", "Format specifier type mismatch", "Unknown format specifier", "Too few format specifiers", "Too many format specifiers", "Scan failed", "Newer CIN version", "Error converting to variant", "Runtime menu error", "Password tampered", "Variant attribute not found", "Incompatible variant data type", "Event data is not available", "Event Store is not present", "Occurrence is not found", "Event Queue is not created", "Event info is not available", "Refnum passed is NULL", "Error retrieving Class GUID", "Error retrieving CoClass GUID", "Error retrieving TypeLib GUID.", "Bad built application magic bytes.", "Specific driver is different from the specific driver associated with the Logical Name.", "There is no session opened to the class driver.", "Max Error", "MAX - Error with config objects", "MAX - Error loading configuration", "MAX - Group not supported"]
        # "Handle mistyped state name (developer tool)"
        # "Do not put any code in this frame.\n(it is a separator no-op)"
        n205 = Format Into String(format string="Software Exception: Unhandled State \"%s\"." ("message"), error in=w509, w510) -> (resulting string=w513:string, error out=w514:errorcluster)  [unwired: 1 in]
        n206 = call <vilib>:"Error Cluster From Error Code.vi"("show call chain? (False)"=TRUE, "error in (no error)"=w514, "error message (\"\")"=w513, "error code (0)"=w512) -> ("error out"=w508:errorcluster)  [unwired: 5 in]
        n207 = call <vilib>:"Add State(s) to Queue__jki_lib_state_machine.vi"("State(s) in (\"\")"=w518) -> ("States Out"=w517:string)  [unwired: 14 in]
      }
      frame "-----Data Collection----" {
        n208 = call <vilib>:"Add State(s) to Queue__jki_lib_state_machine.vi"("State(s) in (\"\")"=w522) -> ("States Out"=w521:string)  [unwired: 14 in]
      }
      frame "Agilent DAQ" {
        # "Reset Agilent if \nfailure"
        n209 = Unbundle By Name(w536) -> ("34972-1"=w529:refnum<visa-resource-name>, "Agilent Channels DAQ"=w528:string)
        n210 = call "Agilent 34970 Get Data Main.vi"("error in (no error)"=w531, "Analog Channels-List"=w528, "VISA Refnum in"=w529) -> ("error out"=w530:errorcluster, "read buffer"=→"read buffer":string, "Sorted Data"=w524:dbl[], "UnSorted Data"=→"Unsorted Data":dbl[])  [unwired: 3 in, 2 out]
        "Raw Data (Scaled)" <- w524
        n211 = local read "Voltage Indexes"() -> (w526:i32[])
        n212 = local read "Disable Channel = True"() -> (w532:bool[])
        n213 = call "HCC Filter NonUsed Agilent Channels.vi"("Disable Channel = True"=w532, "Input Current"=w524, "Voltage Indexes"=w526) -> ("Output Voltage"=w525:dbl[], "Output Current"=w533:dbl[])  [unwired: 6 in, 1 out]
        "Current" <- w533
        "Voltage" <- w525
        n214 = Bundle By Name(cluster=w536, "Current"=w533, "Voltage"=w525) -> (w535:T15)
        n215 = call <vilib>:"Add State(s) to Queue__jki_lib_state_machine.vi"("State(s) in (\"\")"=w538) -> ("States Out"=w537:string)  [unwired: 14 in]
        "Collecting Agilent Data" <- TRUE
      }
      frame "Save Agilent Data" {
        # "Extract the network current path location from the \nLaundry Lab Program and save in this program. This allows\nruntime save"
        n216 = local read "Network Var Set"() -> (w539:u8)
        n217 = Unbundle By Name(w543) -> ("Current"=w545:dbl[], "Voltage"=w540:dbl[])
        n218 = local read "Timer 2"() -> (w542:dbl)
        n219 = for {
          tunnel: w545 -> [w554] mode=indexing
          tunnel: [w553] -> w544 mode=indexing
          tunnel: w542 -> [w552]
          tunnel: w540 -> [w550] mode=indexing
          tunnel: w539 -> [w549]
          i -> [w551]
          n220 = case shown="2" w549 {
            tunnel: w554 -> [w559 w684]
            tunnel: [w558 w681] -> w553
            tunnel: w552 -> [w557 w682]
            tunnel: w551 -> [w556 w680]
            tunnel: w550 -> [w555 w683]
            frame 1, Default {
              n221 = case shown="23" w556 {
                tunnel: w559 -> [w563 w568 w573 w578 w583 w588 w593 w598 w603 w608 w613 w618 w623 w628 w633 w638 w643 w648 w653 w658 w663 w668 w673 w678]
                tunnel: [w564 w569 w574 w579 w584 w589 w594 w599 w604 w609 w614 w619 w624 w629 w634 w639 w644 w649 w654 w659 w664 w669 w674 w679] -> w558
                tunnel: w557 -> [w562 w567 w572 w577 w582 w587 w592 w597 w602 w607 w612 w617 w622 w627 w632 w637 w642 w647 w652 w657 w662 w667 w672 w677]
                tunnel: w555 -> [w561 w565 w570 w575 w580 w585 w590 w595 w600 w605 w610 w615 w620 w625 w630 w635 w640 w645 w650 w655 w660 w665 w670 w675]
                frame 0, Default {
                  n222 = shared-variable "My Computer\\Test Lib.lvlib\\Filepath 0"() -> (w560:T16)  [unwired: 1 in, 1 out]
                  n223 = call "Save File Save Current.vi"("Timer Seconds"=w562, "Voltage"=w561, "File Locations"=w560, "Current"=w563) -> ("Saving"=w564:bool)  [unwired: 7 in]
                }
                frame 1 {
                  n224 = shared-variable "My Computer\\Test Lib.lvlib\\Filepath 1"() -> (w566:T16)  [unwired: 1 in, 1 out]
                  n225 = call "Save File Save Current.vi"("Timer Seconds"=w567, "Voltage"=w565, "File Locations"=w566, "Current"=w568) -> ("Saving"=w569:bool)  [unwired: 7 in]
                }
                frame 2 {
                  n226 = shared-variable "My Computer\\Test Lib.lvlib\\Filepath 2"() -> (w571:T16)  [unwired: 1 in, 1 out]
                  n227 = call "Save File Save Current.vi"("Timer Seconds"=w572, "Voltage"=w570, "File Locations"=w571, "Current"=w573) -> ("Saving"=w574:bool)  [unwired: 7 in]
                }
                frame 3 {
                  n228 = shared-variable "My Computer\\Test Lib.lvlib\\Filepath 3"() -> (w576:T16)  [unwired: 1 in, 1 out]
                  n229 = call "Save File Save Current.vi"("Timer Seconds"=w577, "Voltage"=w575, "File Locations"=w576, "Current"=w578) -> ("Saving"=w579:bool)  [unwired: 7 in]
                }
                frame 4 {
                  n230 = shared-variable "My Computer\\Test Lib.lvlib\\Filepath 4"() -> (w581:T16)  [unwired: 1 in, 1 out]
                  n231 = call "Save File Save Current.vi"("Timer Seconds"=w582, "Voltage"=w580, "File Locations"=w581, "Current"=w583) -> ("Saving"=w584:bool)  [unwired: 7 in]
                }
                frame 5 {
                  n232 = shared-variable "My Computer\\Test Lib.lvlib\\Filepath 5"() -> (w586:T16)  [unwired: 1 in, 1 out]
                  n233 = call "Save File Save Current.vi"("Timer Seconds"=w587, "Voltage"=w585, "File Locations"=w586, "Current"=w588) -> ("Saving"=w589:bool)  [unwired: 7 in]
                }
                frame 6 {
                  n234 = shared-variable "My Computer\\Test Lib.lvlib\\Filepath 6"() -> (w591:T16)  [unwired: 1 in, 1 out]
                  n235 = call "Save File Save Current.vi"("Timer Seconds"=w592, "Voltage"=w590, "File Locations"=w591, "Current"=w593) -> ("Saving"=w594:bool)  [unwired: 7 in]
                }
                frame 7 {
                  n236 = shared-variable "My Computer\\Test Lib.lvlib\\Filepath 7"() -> (w596:T16)  [unwired: 1 in, 1 out]
                  n237 = call "Save File Save Current.vi"("Timer Seconds"=w597, "Voltage"=w595, "File Locations"=w596, "Current"=w598) -> ("Saving"=w599:bool)  [unwired: 7 in]
                }
                frame 8 {
                  n238 = shared-variable "My Computer\\Test Lib.lvlib\\Filepath 8"() -> (w601:T16)  [unwired: 1 in, 1 out]
                  n239 = call "Save File Save Current.vi"("Timer Seconds"=w602, "Voltage"=w600, "File Locations"=w601, "Current"=w603) -> ("Saving"=w604:bool)  [unwired: 7 in]
                }
                frame 9 {
                  n240 = shared-variable "My Computer\\Test Lib.lvlib\\Filepath 9"() -> (w606:T16)  [unwired: 1 in, 1 out]
                  n241 = call "Save File Save Current.vi"("Timer Seconds"=w607, "Voltage"=w605, "File Locations"=w606, "Current"=w608) -> ("Saving"=w609:bool)  [unwired: 7 in]
                }
                frame 10 {
                  n242 = shared-variable "My Computer\\Test Lib.lvlib\\Filepath 10"() -> (w611:T16)  [unwired: 1 in, 1 out]
                  n243 = call "Save File Save Current.vi"("Timer Seconds"=w612, "Voltage"=w610, "File Locations"=w611, "Current"=w613) -> ("Saving"=w614:bool)  [unwired: 7 in]
                }
                frame 11 {
                  n244 = shared-variable "My Computer\\Test Lib.lvlib\\Filepath 11"() -> (w616:T16)  [unwired: 1 in, 1 out]
                  n245 = call "Save File Save Current.vi"("Timer Seconds"=w617, "Voltage"=w615, "File Locations"=w616, "Current"=w618) -> ("Saving"=w619:bool)  [unwired: 7 in]
                }
                frame 12 {
                  n246 = shared-variable "My Computer\\Test Lib.lvlib\\Filepath 12"() -> (w621:T16)  [unwired: 1 in, 1 out]
                  n247 = call "Save File Save Current.vi"("Timer Seconds"=w622, "Voltage"=w620, "File Locations"=w621, "Current"=w623) -> ("Saving"=w624:bool)  [unwired: 7 in]
                }
                frame 13 {
                  n248 = shared-variable "My Computer\\Test Lib.lvlib\\Filepath 13"() -> (w626:T16)  [unwired: 1 in, 1 out]
                  n249 = call "Save File Save Current.vi"("Timer Seconds"=w627, "Voltage"=w625, "File Locations"=w626, "Current"=w628) -> ("Saving"=w629:bool)  [unwired: 7 in]
                }
                frame 14 {
                  n250 = shared-variable "My Computer\\Test Lib.lvlib\\Filepath 14"() -> (w631:T16)  [unwired: 1 in, 1 out]
                  n251 = call "Save File Save Current.vi"("Timer Seconds"=w632, "Voltage"=w630, "File Locations"=w631, "Current"=w633) -> ("Saving"=w634:bool)  [unwired: 7 in]
                }
                frame 15 {
                  n252 = shared-variable "My Computer\\Test Lib.lvlib\\Filepath 15"() -> (w636:T16)  [unwired: 1 in, 1 out]
                  n253 = call "Save File Save Current.vi"("Timer Seconds"=w637, "Voltage"=w635, "File Locations"=w636, "Current"=w638) -> ("Saving"=w639:bool)  [unwired: 7 in]
                }
                frame 16 {
                  n254 = shared-variable "My Computer\\Test Lib.lvlib\\Filepath 16"() -> (w641:T16)  [unwired: 1 in, 1 out]
                  n255 = call "Save File Save Current.vi"("Timer Seconds"=w642, "Voltage"=w640, "File Locations"=w641, "Current"=w643) -> ("Saving"=w644:bool)  [unwired: 7 in]
                }
                frame 17 {
                  n256 = shared-variable "My Computer\\Test Lib.lvlib\\Filepath 17"() -> (w646:T16)  [unwired: 1 in, 1 out]
                  n257 = call "Save File Save Current.vi"("Timer Seconds"=w647, "Voltage"=w645, "File Locations"=w646, "Current"=w648) -> ("Saving"=w649:bool)  [unwired: 7 in]
                }
                frame 18 {
                  n258 = shared-variable "My Computer\\Test Lib.lvlib\\Filepath 18"() -> (w651:T16)  [unwired: 1 in, 1 out]
                  n259 = call "Save File Save Current.vi"("Timer Seconds"=w652, "Voltage"=w650, "File Locations"=w651, "Current"=w653) -> ("Saving"=w654:bool)  [unwired: 7 in]
                }
                frame 19 {
                  n260 = shared-variable "My Computer\\Test Lib.lvlib\\Filepath 19"() -> (w656:T16)  [unwired: 1 in, 1 out]
                  n261 = call "Save File Save Current.vi"("Timer Seconds"=w657, "Voltage"=w655, "File Locations"=w656, "Current"=w658) -> ("Saving"=w659:bool)  [unwired: 7 in]
                }
                frame 20 {
                  n262 = shared-variable "My Computer\\Test Lib.lvlib\\Filepath 20"() -> (w661:T16)  [unwired: 1 in, 1 out]
                  n263 = call "Save File Save Current.vi"("Timer Seconds"=w662, "Voltage"=w660, "File Locations"=w661, "Current"=w663) -> ("Saving"=w664:bool)  [unwired: 7 in]
                }
                frame 21 {
                  n264 = shared-variable "My Computer\\Test Lib.lvlib\\Filepath 21"() -> (w666:T16)  [unwired: 1 in, 1 out]
                  n265 = call "Save File Save Current.vi"("Timer Seconds"=w667, "Voltage"=w665, "File Locations"=w666, "Current"=w668) -> ("Saving"=w669:bool)  [unwired: 7 in]
                }
                frame 22 {
                  n266 = shared-variable "My Computer\\Test Lib.lvlib\\Filepath 22"() -> (w671:T16)  [unwired: 1 in, 1 out]
                  n267 = call "Save File Save Current.vi"("Timer Seconds"=w672, "Voltage"=w670, "File Locations"=w671, "Current"=w673) -> ("Saving"=w674:bool)  [unwired: 7 in]
                }
                frame 23 {
                  n268 = shared-variable "My Computer\\Test Lib.lvlib\\Filepath 23"() -> (w676:T16)  [unwired: 1 in, 1 out]
                  n269 = call "Save File Save Current.vi"("Timer Seconds"=w677, "Voltage"=w675, "File Locations"=w676, "Current"=w678) -> ("Saving"=w679:bool)  [unwired: 7 in]
                }
              }
            }
            frame 2 {
              n270 = case shown="18" w680 {
                tunnel: w684 -> [w688 w693 w698 w703 w708 w713 w718 w723 w728 w733 w738 w743 w748 w753 w758 w763 w768 w773 w778 w783 w788 w793 w798 w803]
                tunnel: [w689 w694 w699 w704 w709 w714 w719 w724 w729 w734 w739 w744 w749 w754 w759 w764 w769 w774 w779 w784 w789 w794 w799 w804] -> w681
                tunnel: w682 -> [w687 w692 w697 w702 w707 w712 w717 w722 w727 w732 w737 w742 w747 w752 w757 w762 w767 w772 w777 w782 w787 w792 w797 w802]
                tunnel: w683 -> [w686 w691 w696 w701 w706 w711 w716 w721 w726 w731 w736 w741 w746 w751 w756 w761 w766 w771 w776 w781 w786 w791 w796 w801]
                frame 0, Default {
                  n271 = shared-variable "My Computer\\Test Lib.lvlib\\Filepath 24"() -> (w685:T16)  [unwired: 1 in, 1 out]
                  n272 = call "Save File Save Current.vi"("Timer Seconds"=w687, "Voltage"=w686, "File Locations"=w685, "Current"=w688) -> ("Saving"=w689:bool)  [unwired: 7 in]
                }
                frame 1 {
                  n273 = shared-variable "My Computer\\Test Lib.lvlib\\Filepath 25"() -> (w690:T16)  [unwired: 1 in, 1 out]
                  n274 = call "Save File Save Current.vi"("Timer Seconds"=w692, "Voltage"=w691, "File Locations"=w690, "Current"=w693) -> ("Saving"=w694:bool)  [unwired: 7 in]
                }
                frame 2 {
                  n275 = shared-variable "My Computer\\Test Lib.lvlib\\Filepath 26"() -> (w695:T16)  [unwired: 1 in, 1 out]
                  n276 = call "Save File Save Current.vi"("Timer Seconds"=w697, "Voltage"=w696, "File Locations"=w695, "Current"=w698) -> ("Saving"=w699:bool)  [unwired: 7 in]
                }
                frame 3 {
                  n277 = shared-variable "My Computer\\Test Lib.lvlib\\Filepath 27"() -> (w700:T16)  [unwired: 1 in, 1 out]
                  n278 = call "Save File Save Current.vi"("Timer Seconds"=w702, "Voltage"=w701, "File Locations"=w700, "Current"=w703) -> ("Saving"=w704:bool)  [unwired: 7 in]
                }
                frame 4 {
                  n279 = shared-variable "My Computer\\Test Lib.lvlib\\Filepath 28"() -> (w705:T16)  [unwired: 1 in, 1 out]
                  n280 = call "Save File Save Current.vi"("Timer Seconds"=w707, "Voltage"=w706, "File Locations"=w705, "Current"=w708) -> ("Saving"=w709:bool)  [unwired: 7 in]
                }
                frame 5 {
                  n281 = shared-variable "My Computer\\Test Lib.lvlib\\Filepath 29"() -> (w710:T16)  [unwired: 1 in, 1 out]
                  n282 = call "Save File Save Current.vi"("Timer Seconds"=w712, "Voltage"=w711, "File Locations"=w710, "Current"=w713) -> ("Saving"=w714:bool)  [unwired: 7 in]
                }
                frame 6 {
                  n283 = shared-variable "My Computer\\Test Lib.lvlib\\Filepath 30"() -> (w715:T16)  [unwired: 1 in, 1 out]
                  n284 = call "Save File Save Current.vi"("Timer Seconds"=w717, "Voltage"=w716, "File Locations"=w715, "Current"=w718) -> ("Saving"=w719:bool)  [unwired: 7 in]
                }
                frame 7 {
                  n285 = shared-variable "My Computer\\Test Lib.lvlib\\Filepath 31"() -> (w720:T16)  [unwired: 1 in, 1 out]
                  n286 = call "Save File Save Current.vi"("Timer Seconds"=w722, "Voltage"=w721, "File Locations"=w720, "Current"=w723) -> ("Saving"=w724:bool)  [unwired: 7 in]
                }
                frame 8 {
                  n287 = shared-variable "My Computer\\Test Lib.lvlib\\Filepath 32"() -> (w725:T16)  [unwired: 1 in, 1 out]
                  n288 = call "Save File Save Current.vi"("Timer Seconds"=w727, "Voltage"=w726, "File Locations"=w725, "Current"=w728) -> ("Saving"=w729:bool)  [unwired: 7 in]
                }
                frame 9 {
                  n289 = shared-variable "My Computer\\Test Lib.lvlib\\Filepath 33"() -> (w730:T16)  [unwired: 1 in, 1 out]
                  n290 = call "Save File Save Current.vi"("Timer Seconds"=w732, "Voltage"=w731, "File Locations"=w730, "Current"=w733) -> ("Saving"=w734:bool)  [unwired: 7 in]
                }
                frame 10 {
                  n291 = shared-variable "My Computer\\Test Lib.lvlib\\Filepath 34"() -> (w735:T16)  [unwired: 1 in, 1 out]
                  n292 = call "Save File Save Current.vi"("Timer Seconds"=w737, "Voltage"=w736, "File Locations"=w735, "Current"=w738) -> ("Saving"=w739:bool)  [unwired: 7 in]
                }
                frame 11 {
                  n293 = shared-variable "My Computer\\Test Lib.lvlib\\Filepath 35"() -> (w740:T16)  [unwired: 1 in, 1 out]
                  n294 = call "Save File Save Current.vi"("Timer Seconds"=w742, "Voltage"=w741, "File Locations"=w740, "Current"=w743) -> ("Saving"=w744:bool)  [unwired: 7 in]
                }
                frame 12 {
                  n295 = shared-variable "My Computer\\Test Lib.lvlib\\Filepath 36"() -> (w745:T16)  [unwired: 1 in, 1 out]
                  n296 = call "Save File Save Current.vi"("Timer Seconds"=w747, "Voltage"=w746, "File Locations"=w745, "Current"=w748) -> ("Saving"=w749:bool)  [unwired: 7 in]
                }
                frame 13 {
                  n297 = shared-variable "My Computer\\Test Lib.lvlib\\Filepath 37"() -> (w750:T16)  [unwired: 1 in, 1 out]
                  n298 = call "Save File Save Current.vi"("Timer Seconds"=w752, "Voltage"=w751, "File Locations"=w750, "Current"=w753) -> ("Saving"=w754:bool)  [unwired: 7 in]
                }
                frame 14 {
                  n299 = shared-variable "My Computer\\Test Lib.lvlib\\Filepath 38"() -> (w755:T16)  [unwired: 1 in, 1 out]
                  n300 = call "Save File Save Current.vi"("Timer Seconds"=w757, "Voltage"=w756, "File Locations"=w755, "Current"=w758) -> ("Saving"=w759:bool)  [unwired: 7 in]
                }
                frame 15 {
                  n301 = shared-variable "My Computer\\Test Lib.lvlib\\Filepath 39"() -> (w760:T16)  [unwired: 1 in, 1 out]
                  n302 = call "Save File Save Current.vi"("Timer Seconds"=w762, "Voltage"=w761, "File Locations"=w760, "Current"=w763) -> ("Saving"=w764:bool)  [unwired: 7 in]
                }
                frame 16 {
                  n303 = shared-variable "My Computer\\Test Lib.lvlib\\Filepath 40"() -> (w765:T16)  [unwired: 1 in, 1 out]
                  n304 = call "Save File Save Current.vi"("Timer Seconds"=w767, "Voltage"=w766, "File Locations"=w765, "Current"=w768) -> ("Saving"=w769:bool)  [unwired: 7 in]
                }
                frame 17 {
                  n305 = shared-variable "My Computer\\Test Lib.lvlib\\Filepath 41"() -> (w770:T16)  [unwired: 1 in, 1 out]
                  n306 = call "Save File Save Current.vi"("Timer Seconds"=w772, "Voltage"=w771, "File Locations"=w770, "Current"=w773) -> ("Saving"=w774:bool)  [unwired: 7 in]
                }
                frame 18 {
                  n307 = shared-variable "My Computer\\Test Lib.lvlib\\Filepath 42"() -> (w775:T16)  [unwired: 1 in, 1 out]
                  n308 = call "Save File Save Current.vi"("Timer Seconds"=w777, "Voltage"=w776, "File Locations"=w775, "Current"=w778) -> ("Saving"=w779:bool)  [unwired: 7 in]
                }
                frame 19 {
                  n309 = shared-variable "My Computer\\Test Lib.lvlib\\Filepath 43"() -> (w780:T16)  [unwired: 1 in, 1 out]
                  n310 = call "Save File Save Current.vi"("Timer Seconds"=w782, "Voltage"=w781, "File Locations"=w780, "Current"=w783) -> ("Saving"=w784:bool)  [unwired: 7 in]
                }
                frame 20 {
                  n311 = shared-variable "My Computer\\Test Lib.lvlib\\Filepath 44"() -> (w785:T16)  [unwired: 1 in, 1 out]
                  n312 = call "Save File Save Current.vi"("Timer Seconds"=w787, "Voltage"=w786, "File Locations"=w785, "Current"=w788) -> ("Saving"=w789:bool)  [unwired: 7 in]
                }
                frame 21 {
                  n313 = shared-variable "My Computer\\Test Lib.lvlib\\Filepath 45"() -> (w790:T16)  [unwired: 1 in, 1 out]
                  n314 = call "Save File Save Current.vi"("Timer Seconds"=w792, "Voltage"=w791, "File Locations"=w790, "Current"=w793) -> ("Saving"=w794:bool)  [unwired: 7 in]
                }
                frame 22 {
                  n315 = shared-variable "My Computer\\Test Lib.lvlib\\Filepath 46"() -> (w795:T16)  [unwired: 1 in, 1 out]
                  n316 = call "Save File Save Current.vi"("Timer Seconds"=w797, "Voltage"=w796, "File Locations"=w795, "Current"=w798) -> ("Saving"=w799:bool)  [unwired: 7 in]
                }
                frame 23 {
                  n317 = shared-variable "My Computer\\Test Lib.lvlib\\Filepath 47"() -> (w800:T16)  [unwired: 1 in, 1 out]
                  n318 = call "Save File Save Current.vi"("Timer Seconds"=w802, "Voltage"=w801, "File Locations"=w800, "Current"=w803) -> ("Saving"=w804:bool)  [unwired: 7 in]
                }
              }
            }
          }
        }
        "Save Array" <- w544
        n319 = call <vilib>:"Add State(s) to Queue__jki_lib_state_machine.vi"("State(s) in Front (\"\")"="" ("State(s) in Front (\"\")"), "State(s) in (\"\")"=w548) -> ("States Out"=w547:string)  [unwired: 13 in]
      }
      frame "------Exit Routine------" {
        n320 = call <vilib>:"Add State(s) to Queue__jki_lib_state_machine.vi"("State(s) in (\"\")"=w809) -> ("States Out"=w808:string)  [unwired: 14 in]
      }
      frame "Exit" {
        n321 = call <vilib>:"Add State(s) to Queue__jki_lib_state_machine.vi"("State(s) in (\"\")"=w814) -> ("States Out"=w813:string)  [unwired: 14 in]
      }
    }
    n322 = case shown="True" w432 {
      tunnel: w434 -> [_ w446]
      tunnel: w435 -> [w444 w447]
      tunnel: [w444 w445] -> w433
      frame False {
      }
      frame True {
        n323 = Build Array (concatenate)(w447, w446) -> (w445:string[])
        "DAQ Loop" <- w445
      }
    }
  }
  "error out" <- w7
